vi "resha arc - v1.vi"() -> ()   [LabVIEW 2015]
doc: "This is the interface, the one VI which loads all the others. Run this one first.\n\n(the line below ensures settings are saved)\n[Red Tweezers Save Settings]"
uses:
  Matt Fall 2018 files/Matt working/Red Tweezers Image Processing Final 1-19/subvis/line_trapping.ctl
  Matt Fall 2018 files/Matt working/Red Tweezers Image Processing Final 1-19/subvis/spot.ctl
  <vilib>/userdefined/High Color/IMAQdx.ctl
  Matt Fall 2018 files/Matt working/Red Tweezers Image Processing Final 1-19/subvis/selection_element.ctl
  <vilib>/Analysis/Matrix/Datatypes/RealMatrix.ctl
  Matt Fall 2018 files/Matt working/Red Tweezers Image Processing Final 1-19/subvis/mouse_info.ctl
  <vilib>/Analysis/baseanly.llb/Real A x B.vi
  Matt Fall 2018 files/Matt working/Red Tweezers Image Processing Final 1-19/subvis/red_tweezers_globals_INTERNAL_VOLATILE.vi
  Matt Fall 2018 files/Matt working/Red Tweezers Image Processing Final 1-19/subvis/red_tweezers_globals.vi
  <vilib>/Analysis/Matrix/Numeric/Multiply/Multiply - RM,R.vi
  <vilib>/Analysis/Matrix/Numeric/Multiply/Multiply - R,RM.vi
  <vilib>/Analysis/NI_AALBase.lvlib
  <vilib>/vision/driver/NI_Vision_Acquisition_Software.lvlib
  <vilib>/vision/NI_Vision_Development_Module.lvlib
  <vilib>/Analysis/Matrix/NI_Matrix.lvlib
panel:
  out "Specific Point":cluster{i32, i32}
  out "bottomrx 3":dbl
  out "toply 3":dbl
  out "bottomry 3":dbl
  out "toplx 3":dbl
  out "Circles 2":T1(array[cluster]) {"Position"."Y" format="%.2f"; "Position"."X" format="%.2f"}
  out "Spot Storage":T2[](array[typedef]) {"Amplitude Correction" step=0.1; "Line Trapping"."Phase Gradient" step=0.05; "Line Trapping"."Vector"."x" step=1e-06 format="%#_6p"; "Line Trapping"."Vector"."y" step=1e-06 format="%#_6p"; "Line Trapping"."Vector"."z" step=1e-06 format="%#_6p"; "NA Position"."r" step=1e-06; "NA Position"."y" step=1e-06; "NA Position"."x" step=1e-06; "Position"."z" step=1e-06; "Position"."y" step=1e-06; "Position"."x" step=1e-06; "Phase" step=0.7753; "Intensity" step=0.1}
  out "# selected":i16
  out "Last Pattern":T2[](array[typedef]) {"Amplitude Correction" step=0.1; "Line Trapping"."Phase Gradient" step=0.05; "Line Trapping"."Vector"."x" step=1e-06 format="%#_6p"; "Line Trapping"."Vector"."y" step=1e-06 format="%#_6p"; "Line Trapping"."Vector"."z" step=1e-06 format="%#_6p"; "NA Position"."r" step=1e-06; "NA Position"."y" step=1e-06; "NA Position"."x" step=1e-06; "Position"."z" step=1e-06; "Position"."y" step=1e-06; "Position"."x" step=1e-06; "Phase" step=0.7753; "Intensity" step=0.1}
  out "Plugins":T4(array[cluster])=[{"Name"="ASI Stage", "Folder"=path "C:/Users/Richard Bowman/Dropbox/red_tweezers_1_4_rc4/plugins/ASI Stage.llb", "vi reference"=refnum, "Needs to be run"=TRUE, "Error"={"status"=FALSE, "code"=0, "source"=""}}, {"Name"="iTweezers", "Folder"=path "C:/Users/Richard Bowman/Dropbox/red_tweezers_1_4_rc4/plugins/iTweezers.llb", "vi reference"=refnum, "Needs to be run"=TRUE, "Error"={"status"=FALSE, "code"=0, "source"=""}}, {"Name"="MightexLED", "Folder"=path "C:/Users/Richard Bowman/Dropbox/red_tweezers_1_4_rc4/plugins/MightexLED.llb", "vi reference"=refnum, "Needs to be run"=TRUE, "Error"={"status"=FALSE, "code"=0, "source"=""}}]
  in  "Tab":T5(tab)
  out "Play Pressed":bool
  out "Y":dbl
  out "X":dbl
  in  "O Button":bool
  in  "OK Button":bool
  in  "Bubble Size":dbl=50.0002
  out "Hit Indicator":bool
  in  "On":bool
  out "Induce check":bool
  out "Area+ Buffer":dbl
  in  "Area to check":dbl=0.00025
  out "Prev Current Spot":dbl
  out "spots selected 2":i32=4
  out "Spot # Check":dbl
  out "Orig Y SC":dbl
  out "Orig X SC":dbl
  out "ID num check":dbl
  out "Value Check":dbl
  out "ID":dbl[](array[numeric])
  out "Null array":dbl[](array[numeric])
  out "Potential Collisions":dbl
  out "What to Check":dbl[](array[numeric])
  out "Num":dbl
  out "Old Y":dbl
  out "Old X":dbl
  out "init":dbl
  out "Looper":bool
  in  "Output to SLM":bool
  out "Maximum":dbl
  out "Projected Distance":dbl
  out "Previous Distance":dbl
  out "Group ID #":dbl
  in  "Buffer Zone":dbl=7e-05
  out "# of Spots":dbl
  out "Distance":dbl
  out "Hit":bool
  out "Y Displacement":dbl
  out "X Displacement":dbl
  out "Current Spot #":dbl
  out "spots selected":i32=4
  in  "lock aspect ratio":bool=TRUE
  in  "Size":cluster{"x":dbl, "y":dbl, "z":dbl} {"z" step=1e-06 format="%#_4p"; "y" step=1e-06 format="%#_4p"; "x" step=1e-06 format="%#_4p"}
  in  "phase":dbl step=0.7753
  in  "Vortex Charge":i8
  in  "Intensity":dbl=1.0 step=0.1
  in  "add to selection":bool
  in  "random position":bool
  in  "new spot":bool
  in  "delete":bool
  in  "rotate":bool
  in  "Rotation Axis":u16(ring)=2 items=["Z", "X", "Y", "Custom"]
  in  "Angle (degrees)":dbl=2.0
  in  "Custom Axis":cluster{dbl, dbl, dbl}
  in  "Spot Shape":enum32{"Normal", "Line", "NA", "Mixed"}(tab)=enum."Mixed"
  in  "Line Trapping":T3 {"Phase Gradient" step=0.05; "Vector"."x" step=1e-06 format="%#_4p"; "Vector"."y" step=1e-06 format="%#_4p"; "Vector"."z" step=1e-06 format="%#_4p"}
  in  "Scale back aperture":dbl=1.1 step=0.1
  in  "Scale BA":bool
  in  "Position on back aperture":cluster{"x":dbl, "y":dbl}={"x"=-5.84327907697451e-18, "y"=0.0} {"y" step=0.1 format="%#_4p"; "x" step=0.1 format="%#_4p"}
  in  "Radius on back aperture":dbl=1.1 step=0.1
  in  "Generate":bool
  in  "Pattern":T6(tab)
  in  "Spots across centre":i32=5
  in  "Reference Array?":bool
  in  "Fraction of SLM":dbl=1.0
  in  "Spots across centre":i32=5
  in  "N":cluster{i32, i32}
  in  "spacing/m":dbl=2.0
  in  "Iterations":i32=10
  out "non-uniformity":dbl(slide)=0.031119223416512406 scale=0.0..0.2
  out "efficiency":dbl(slide)=0.8985936267644501 scale=0.0..1.0
  in  "Optimise":bool
  in  "Reset Phase/Amplitude":bool
  in  "Fall-off/m":dbl=0.00025 min=0.0 step=1e-06 format="%#_4p"
  in  "Abort Plugin":bool
  in  "Plugin:":u16(ring)=1 items=["ASI Stage", "iTweezers", "MightexLED"]
  in  "Save Video":bool
  in  "Global ROI (requires restart)":i32[](array[numeric])=[0, 0, 1280, 512]
  in  "Zoom":bool
  in  "Draw ROI":bool
  in  "Zoom to Fit":bool
  out "Image Information":string="640x480 1.93X 8-bit image 255    (0,0)"
  in  "Camera":T7
  in  "Time per Frame (ms)":dbl
  in  "Edit Sequence Mode":bool
  in  "Manual Edit":bool
  in  "Bubble ID to Empty":dbl
  in  "Clearance Button":bool
  in  "Manual Sequence":bool
  in  "Play Sequence":bool
  in  "Reset":bool
  out "Sequence Instances":dbl
  out "Counter":dbl
  in  "Save State":bool
  out "Sequence On?":bool
  in  "Sequence Order":dbl
  out "Selection/Group":T8[](array[typedef])
  in  "Sequence Storer":T2[][](array[typedef]) {"Amplitude Correction" step=0.1; "Line Trapping"."Phase Gradient" step=0.05; "Line Trapping"."Vector"."x" step=1e-06 format="%#_6p"; "Line Trapping"."Vector"."y" step=1e-06 format="%#_6p"; "Line Trapping"."Vector"."z" step=1e-06 format="%#_6p"; "NA Position"."r" step=1e-06; "NA Position"."y" step=1e-06; "NA Position"."x" step=1e-06; "Position"."z" step=1e-06; "Position"."y" step=1e-06; "Position"."x" step=1e-06; "Phase" step=0.7753; "Intensity" step=0.1}
  in  "Object New Y":dbl
  in  "Object New X":dbl
  in  "Input Object Location":bool
  out "Time Elapsed(ms)":i32
  out "Start":i32
  out "Stop":i32
  out "Insert End":bool
  out "NewXYRates":dbl[][](array[numeric])
  out "NewXYArraySize":dbl
  out "NewXYArray":dbl[][](array[numeric])
  in  "Rates":dbl
  out "LCS Y":dbl
  out "LCS X":dbl
  in  "LCS":dbl
  in  "Play":bool
  out "Initiate Creation 2":dbl
  in  "Max Number of Bubbles 2":dbl
  in  "Number of Planned Sequence Frames 2":dbl
  in  "Add Additional Frames":bool
  in  "Frame Location":dbl
  in  "Additional Frames Wanted":dbl
  in  "Tab Control":enum32{"Line", "Arc"}(tab)
  out "X Rate":dbl
  out "Y Rate":dbl
  out "Original\nRadius":dbl
  out "Original\nD-Y":dbl
  out "Original\nD-X":dbl
  out "Original \nTheta":dbl
  out "Center Y":dbl
  out "Center X":dbl
  out "Center location":dbl[][](array[numeric])
  out "Degree Rate":dbl
  out "ROI-X":dbl
  out "ROI-Y":dbl
  in  "Lock Current Spot":bool
  out "Locked Current Spot":dbl
  out "Numeric":dbl
  out "probe":dbl
  in  "Insert":bool
  in  "Start at Which Frame?":dbl
  out "Original Y":dbl
  out "Original X":dbl
  in  "Mark Original Position":bool
  in  "How Many Frames?":dbl
  out "New Y":dbl
  out "New X":dbl
  out "Spot Storage 2":T2[](array[typedef]) {"Amplitude Correction" step=0.1; "Line Trapping"."Phase Gradient" step=0.05; "Line Trapping"."Vector"."x" step=1e-06 format="%#_6p"; "Line Trapping"."Vector"."y" step=1e-06 format="%#_6p"; "Line Trapping"."Vector"."z" step=1e-06 format="%#_6p"; "NA Position"."r" step=1e-06; "NA Position"."y" step=1e-06; "NA Position"."x" step=1e-06; "Position"."z" step=1e-06; "Position"."y" step=1e-06; "Position"."x" step=1e-06; "Phase" step=0.7753; "Intensity" step=0.1}
  in  "Numeric 2":dbl
  in  "Save":bool
  in  "Load":bool
  out "Current Y":dbl
  out "Current X":dbl
  out "Calc New  Y":dbl
  out "Calc New X":dbl
  out "distance bw y and rad":dbl
  out "distance  bw x and rad":dbl
  out "Object Y":dbl
  out "Object X":dbl
  in  "Camera Capture 2":bool
  out "Object y":dbl
  out "Object x":dbl
  out "Number of Matches Returned 2":dbl
  out "bottomry 2":dbl
  out "toply 2":dbl
  out "bottomrx 2":dbl
  out "toplx 2":dbl
  in  "Send Data":bool
  out "Camera 3":T9(plugin-control)
  in  "Circle Descriptor 2":cluster{"Min Radius":dbl, "Max Radius":dbl}={"Min Radius"=3.0, "Max Radius"=500.0}
  out "Video Frame Rate":dbl(knob)=50.00000000000003 scale=0.0..100.0 scale format="%.1f"
  out "Interface Frame Rate":dbl(knob)=97.23240312927678 scale=0.0..100.0 scale format="%.1f"
  in  "stop":bool=TRUE
  out "Numeric 4":dbl
  in  "Position":cluster{"x":dbl, "y":dbl, "z":dbl}={"x"=1e-06, "y"=-6.3e-06, "z"=0.0} {"z" step=1e-06 format="%#_4p"; "y" step=1e-06 format="%#_4p"; "x" step=1e-06 format="%#_4p"}
  out "Numeric 3":dbl
  out "ROI 1":T10
  out "ROI 0":T10
  out "MOP pressed":bool
  out "MOP pressed After":bool
  out "X Pos every 10 sec":dbl
  out "Elapsed Time":dbl
  out "Position Indicator":string
  out "Spot Checker":T2[](array[typedef]) {"Amplitude Correction" step=0.1; "Line Trapping"."Phase Gradient" step=0.05; "Line Trapping"."Vector"."x" step=1e-06 format="%#_6p"; "Line Trapping"."Vector"."y" step=1e-06 format="%#_6p"; "Line Trapping"."Vector"."z" step=1e-06 format="%#_6p"; "NA Position"."r" step=1e-06; "NA Position"."y" step=1e-06; "NA Position"."x" step=1e-06; "Position"."z" step=1e-06; "Position"."y" step=1e-06; "Position"."x" step=1e-06; "Phase" step=0.7753; "Intensity" step=0.1}
  out "Image":T9(plugin-control)
  # "Notes:\n\nIf you are doing non-sequence controls,\nthe delete function can be used as intended.\nHowever, do not use the delete function after\nrunning a sequence! Using it will prevent\nthe bubbles from appearing as the\nnumber of spots will change, which is\nessential for the sequence to work (it would\nbe displaying the maximum number of\nbubbles). \n\nIf you happen to delete a bubble, it can be \nrestored by inserting a new spot. Once enough\nspots have been restored, click on manual edit\nto correct the # of spots tracker. It should \nbe restored to where it originally was."
  # "The SLM can be used to shape spots; here you can restrict the NA of a spot (so it comes only from part of the back aperture), or create a line-trap"
  # "The traps do not have any spot-shaping applied (so they should just be diffraction-limited focal spots)."
  # "This shapes the amplitude (and phase) of the beam to create extended line traps.  The \"Phase Gradient\" control allows the Poynting vector to push things along the line.  Unfortunately, some work is needed on the scaling factors so the phase gradient control will need tweaking if the line trap has a nonzero z component."
  # "By default,each spot comes from the whole back aperture.  Here, you can limit a spot to come from a specific part of the back aperture."
  # "The control below allows you to scale the whole back aperture (i.e. the position and size of all the apertures).  It's a one-time operation, i.e. only changes things when you push \"ok\"."
  # "A Combination of line-trapping and NA restriction has been applied to these traps.  You can get at the line trap or NA parameters on the other tabs, switching to the NA tab does not delete the line-trap settings."
  # "This tab generates Shack-Hartmann type holograms, which are often useful when aligning the system, and arrays of spots."
  # "The controls above only work when using the \"IMAQdx with ROI Buttons\" case in the bottom loop.  You can save video regardless of camera code though."
  # "Manual Edit allows a user to\ngo to a specific sequence frame."
  # "To clear the sequence, you must\nclear the array. Right click on sequence\nstorer to do this."
  # "Use this to \"clear\" a \nspecific bubble. If\nworking on a sequence,\nuse this as your delete\nbutton! You can update\nthe view by using manual edit."
  # "Use the reset button\nto clear counter.\nIt becomes necessary\nwhen you clear the array,\nespecially in manual mode."
  # "Use the sequence creator tab to specify the\nnumber of bubbles you want along with\nthe number of frames.\n\nTo save at a specific interval, the sequence\norder can be used to place the state. If used\nto correct something, it will replace the\nentire sequence frame.\n\n\"Sequence On?\" is only used in auto mode."
  # "Multiple bubbles can  be done with the\nline function. One bubble at a time for the arc\nfunction."
  # "Using the Load/Save function:\n\nRed Tweezers itself is unable to save long \nsequences, but a separate program is able to\naccomplish this. To do this, follow these\nsteps:\n\n1. After creating your sequence, press the save\nbutton below.\n\n2. Then, go to the subvi folder and find\nSequenceSaver.vi.\n\n3. At the control \"Sequence Storer,\" right-click\nthe dimensions part of the array and go to\ndata operations.\n\n4. Press \"Make Current Values Default\" and save\nthe sequence.\n\n5. The next time you load the program, simply\npress load to re-acquire the sequence. You\nwill need to insert the bubbles again, but after\nthe first frame can be recovered by using\nSequenceControl.vi."
types:
  T1 = cluster{"Position":cluster{"X":sgl, "Y":sgl}, "Radius":dbl, "Score":dbl}[]
  T2 = typedef "spot.ctl" = cluster{"Position":cluster{"x":dbl, "y":dbl, "z":dbl}, "Intensity":dbl, "Vortex Charge":i8, "Phase":dbl, "NA Position":cluster{"x":dbl, "y":dbl, "r":dbl}, "Line Trapping":T3, "Amplitude Correction":dbl}
  T3 = typedef "line_trapping.ctl" = cluster{"Vector":cluster{"x":dbl, "y":dbl, "z":dbl}, "Phase Gradient":dbl}
  T4 = cluster{"Name":string, "Folder":path, "vi reference":refnum<vi>, "Needs to be run":bool, "Error":errorcluster}[]
  T5 = enum32{"Current Spot", "Rotate", "Spot Shape", "Patterns", "Plugins", "Video", "Sequence", "Sequence Creator", "Spot Control", "Load/Save", "Image Process"}
  T6 = enum32{"HCP Shack-Hartmann", "Square Shack-Hartmann", "Rectangular Grid"}
  T7 = typedef "IMAQdx.ctl" = refnum<k21>
  T8 = typedef "selection_element.ctl" = cluster{"Group ID":i32, "Selected":bool}
  T9 = typedef "IMAQ Image.ctl" = refnum<image>
  T10 = typedef "NI_Matrix.lvlib/RealMatrix.ctl" = dbl[][]
  T11 = typedef "mouse_info.ctl" = cluster{"Button Down":bool, "Dragging":bool, "Position (Image Pixels)":cluster{"X":dbl, "Y":dbl}, "Previous Position (Image Pixels)":cluster{"X":dbl, "Y":dbl}, "Button":u16, "Mods":cluster{"Double Click":bool, "Menu Key":bool}, "PlatMods":cluster{"Shift":bool, "Ctrl":bool, "Alt":bool, "Cmd":bool, "Opt":bool}}
  T12 = cluster{"Desired Font (Application)":enum16{"User-specified Font", "Application Font", "System Font", "Dialog Font"}, "[User-specified Font]":cluster{"Font Name":string, "Size":i16, "Strikeout?":bool, "Italic?":bool, "Underline?":bool, "Outline?":bool, "Shadow?":bool, "Bold?":bool, "Rotation Angle":dbl}, "Horizontal Alignment":i16, "Vertical Alignment":i16}
  T13 = cluster{"Position":cluster{"x":dbl, "y":dbl, "z":dbl}, "Intensity":dbl, "Vortex Charge":i8, "Phase":dbl, "NA Position":cluster{"x":dbl, "y":dbl, "r":dbl}, "Line Trapping":T3, "Amplitude Correction":dbl}
  T14 = enum16{"Set guide visibility", "Set grid visibility", "Show front panel", "Render on image"}
  T15 = enum32{"Current Spot", "Rotate", "Spot Shape", "Patterns", "Plugins", "Video"}
  T16 = enum16{"Left Button", "Center Button", "Right Button", "Window Close"}
  T17 = typedef "Image Type" = u32
  T18 = cluster{"number: 0 to 1":dbl, "number: 0 to 1":dbl}
  T19 = typedef "overlay_element.ctl" = cluster{"Tool":enum16{"Lines", "Oval", "Rectangle", "Text"}, "Points":cluster{"X":dbl, "Y":dbl}[], "Drawing Mode":u32, "Color":u32, "String":string}
  T20 = enum32{"Current Spot", "Rotate", "Spot Shape", "Patterns", "Plugins", "Video", "Particle Tracking", "Clamping", "Blank"}[]
  T21 = typedef "LVMenuShortCut.ctl" = cluster{"include Shift key?":bool, "include Ctrl key?":bool, "shortcut key":string}
  T22 = typedef "LVPoint32TypeDef.ctl" = cluster{"Horizontal":i32, "Vertical":i32}
  T23 = cluster{"Shift":bool, "Ctrl":bool, "Alt":bool, "Cmd":bool, "Opt":bool}
  T24 = cluster{"Button Down":bool, "Dragging":bool, "Mouse Coords (image pixels)":cluster{dbl, dbl}, "Mouse Coords (image pixels)":cluster{dbl, dbl}, "Button":u16, "Mods":cluster{"Double Click":bool, "Menu Key":bool}, "PlatMods":cluster{"Shift":bool, "Ctrl":bool, "Alt":bool, "Cmd":bool, "Opt":bool}}
  T25 = cluster{"Position":cluster{"X":sgl, "Y":sgl}, "Radius":dbl, "Score":dbl}
  T26 = cluster{"Global Rectangle":i32[], "Contours":cluster{"Contour Type":u32, "ROI Type":u32, "Points":i32[]}[]}
  T27 = cluster{"Contour Type":u32, "ROI Type":u32, "Points":i32[]}[]
  T28 = cluster{"Contour Type":u32, "ROI Type":u32, "Points":i32[]}
  T29 = cluster{"[0]":dbl, "[1]":dbl, "[2]":dbl, "[3]":dbl}
  T30 = cluster{"NewXYArray[0]":dbl, "NewXYArray[1]":dbl, "NewXYArray[2]":dbl, "NewXYArray[3]":dbl, "NewXYArray[4]":dbl, "NewXYArray[5]":dbl, "NewXYArray[6]":dbl, "NewXYArray[7]":dbl, "NewXYArray[8]":dbl}
  T31 = cluster{"Average Frame Time":dbl, "millisecond timer value":u32}
  T32 = cluster{"Position":cluster{"x":dbl, "y":dbl, "z":dbl}, "Intensity":dbl, "Vortex Charge":i8, "Phase":dbl, "NA Position":cluster{"x":dbl, "y":dbl, "r":dbl}, "Line Trapping":T3, "Amplitude Correction":dbl}[]
  T33 = enum32{"Bad", "Idle", "Run top level", "Running"}
  T34 = typedef "AviRefnum.ctl" = refnum<k1>
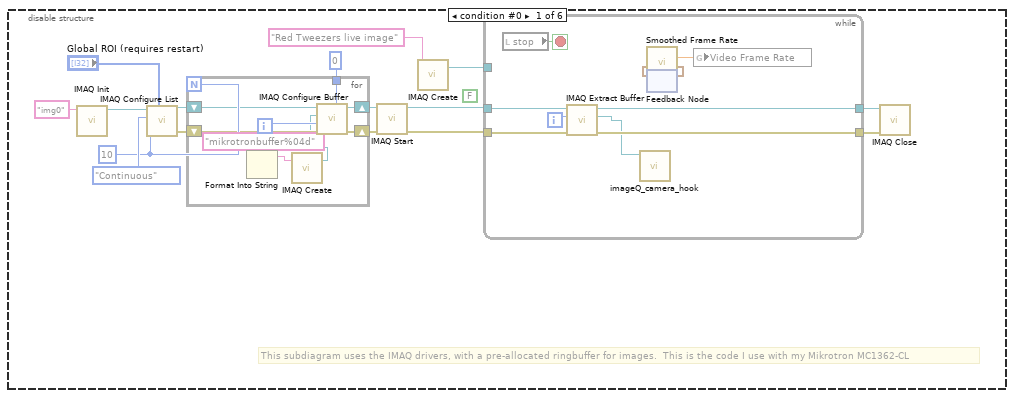
[diagram p3: hidden frame]
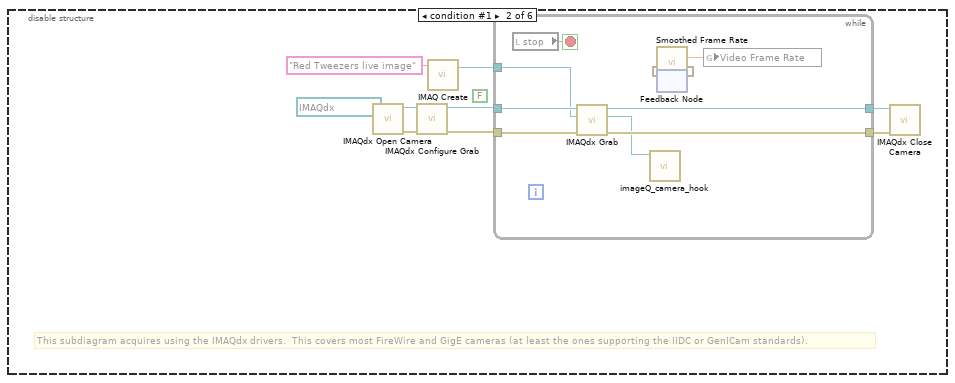
[diagram p4: hidden frame]
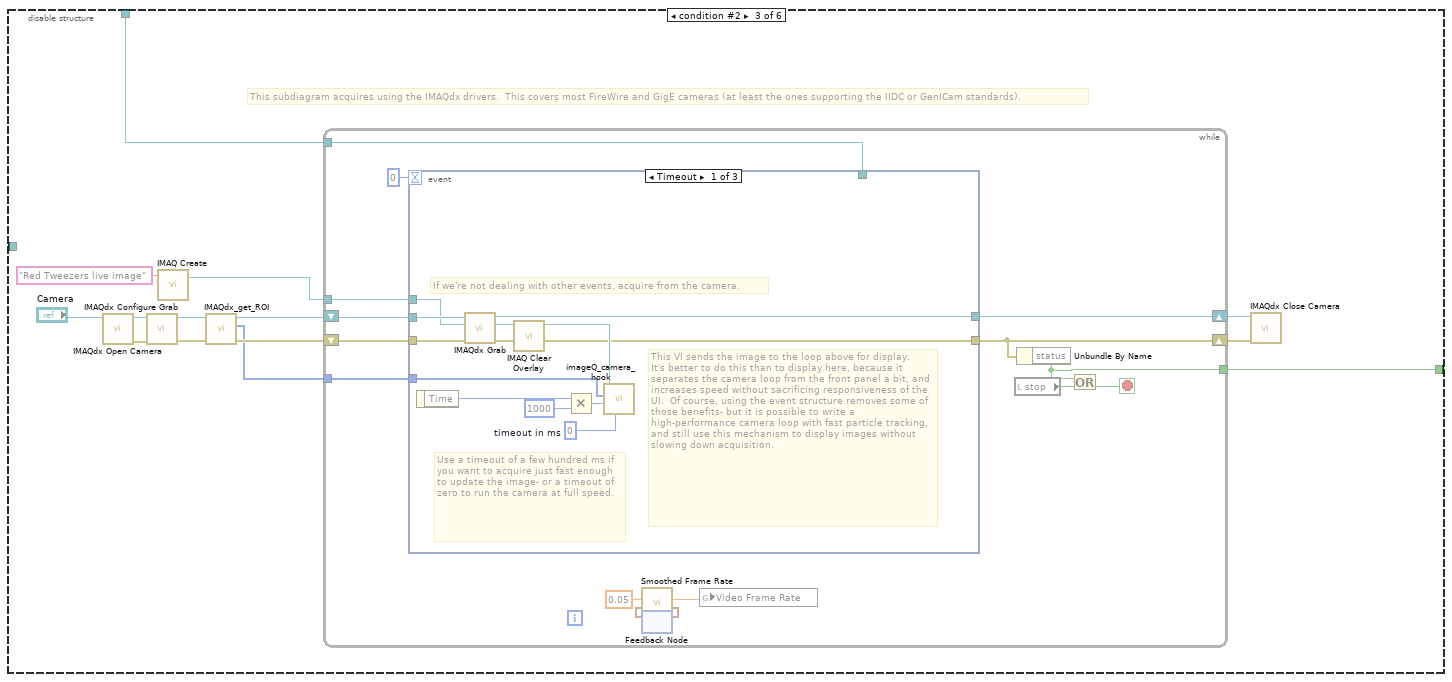
[diagram p5: hidden frame]
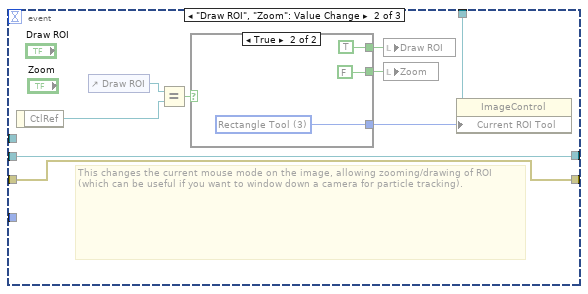
[diagram p6: hidden frame]
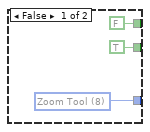
[diagram p7: hidden frame]
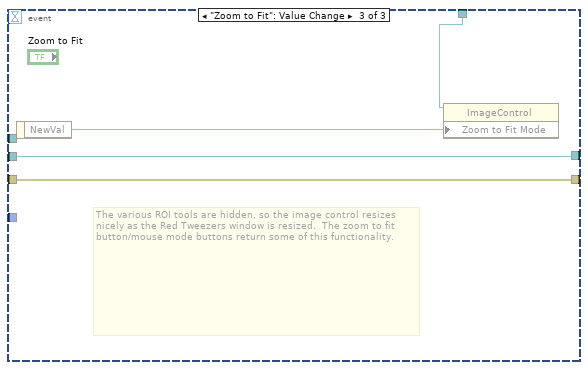
[diagram p8: hidden frame]
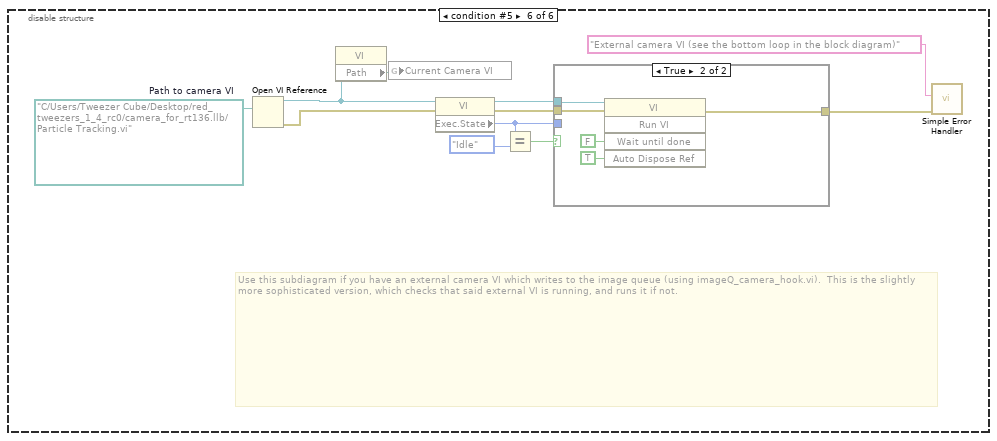
[diagram p10: hidden frame]
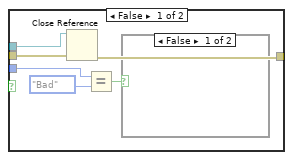
[diagram p11: hidden frame]
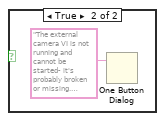
[diagram p12: hidden frame]
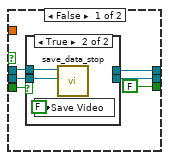
[diagram p13: hidden frame]
diagram:
  w11 = "red_tweezers_display_imageQ" ("Queue Name")
  w23 = T11 {"Button Down"=FALSE, "Dragging"=FALSE, "Position (Image Pixels)"={"X"=0.0, "Y"=0.0}, "Previous Position (Image Pixels)"={"X"=0.0, "Y"=0.0}, "Button"=0, "Mods"={"Double Click"=FALSE, "Menu Key"=FALSE}, "PlatMods"={"Shift"=FALSE, "Ctrl"=FALSE, "Alt"=FALSE, "Cmd"=FALSE, "Opt"=FALSE}}  # Mouse Information
  w24 = refnum<vi> refnum  # Image
  # "The funny looking feedback-node structure is deliberate (if odd).  We want to reload settings from the last used file (stored in the registry) only if this program has not been run since it was last loaded from file/recompiled.  That's why I use an uninitialised shift register: every time the program runs, it increments.  So, if it is zero, this is our first run (or we've been recently recompiled)."
  # "This loop handles the video that is displayed on-screen and saved to file."
  # "Initially, we only register to be told when the user clicks the image"
  # "This is the actual image control"
  # "This is a generic reference.\nIt is just a placeholder, so we can register for events later."
  # "This version of red tweezers uses two coordinate systems: \n1. Real Coordinates - corresponding to physical distances in 3D in microns\n2. Image Coordinates - position on the camera image, relative to the top left of the CURRENT ROI, measured in pixels. If the ROI changes, the relationship between \"real units\" and \"image pixels\" may change, so all values should be stored and presented to the user in REAL units unless there is a good reason to do otherwise."
  n1 = control-ref of="Plugin Pnl"() -> (w20:refnum<vi>)
  n2 = flat-sequence {
    tunnel: [w27] -> w6
    tunnel: w4 -> [_]
    frame #0 {
      n3 = vi-ref "red_tweezers_globals_INTERNAL.vi"() -> (w28:refnum<vi>)
      n4 = property class="VI"(reference=w28) -> ("Path"=w27:path)  [unwired: 1 in, 2 out]
      n5 = global write "red_tweezers_globals_INTERNAL_VOLATILE.vi" "Current Camera VI"(w27) -> ()
    }
  }
  n6 = control-ref of="Plugin:"() -> (w21:refnum<vi>)
  n7 = feedback #1() -> (w14:dbl)  [unwired: 1 in]
  n8 = Equal To 0?(x=w14) -> (x = 0?=w13:bool)
  n9 = Increment(x=w14) -> (x+1=w12:dbl)
  n10 = feedback-in #1(w12) -> ()
  n11 = call "plugins_load.vi"("Sub Panel"=w20, "Plugin Chooser"=w21) -> ("error out"=w15:errorcluster, "Plugins"=w17:T4)  [unwired: 2 in, 2 out]
  "Plugins" <- w17
  n12 = control-ref of="Image"() -> (w5:refnum<vi>)
  n13 = case shown="True" w13 {
    tunnel: w15 -> [_ w29]
    tunnel: [_ w29] -> w4
    frame False {
    }
    frame True {
      n14 = call "settings_load_default_file.vi"("error out"=w29) -> ()
    }
  }
  n15 = flat-sequence {
    tunnel: w4 -> [_]
    tunnel: w2 -> [w31]
    frame #0 {
      # "ensure we don't accidentally start saving video, and run UDP Sender to set up the hologram window."
      n16 = local write "Save Video"(FALSE ("background subtraction")) -> ()
      n17 = call "UDP Sender generic_2.vi"("Spots"=w31) -> ()  [unwired: 2 in, 1 out]
    }
  }
  n18 = global read "red_tweezers_globals.vi" "Selection/Group"() -> (w22:T8[])
  n19 = register-events(w5, w24, w24, w24) -> (reference out=w25:refnum<event-registration>)  [unwired: 2 in, 1 out]
  n20 = global read "red_tweezers_globals.vi" "Spots"() -> (w2:T2[])
  n21 = local write "stop"(FALSE ("STOP")) -> ()
  n22 = call "ensure_selection_matches_spots.vi"("Selection and Groups in"=w22, "Spots"=w2) -> ("Selection and Groups out"=w26:T8[], "Spots (duplicate)"=w1:T2[])  [unwired: 4 in]
  n23 = call "IMAQ Create"("Image Name"=w11) -> ("New Image"=w9:T9)  [unwired: 4 in, 1 out]
  n24 = call "imageQ_create_return_queue.vi"("Queue Name"=w11) -> ("queue out"=w10:refnum<queue>)
  n25 = while {
    shift-right: [w142] -> _
    shift-left: w1 -> [w162]
    shift-right: [w161] -> _
    shift-left: w26 -> [w160]
    shift-right: [w164] -> _
    shift-left: _ -> [w155]
    shift-right: [w163] -> _
    shift-left: _ -> [w154]
    tunnel: w5 -> [w159]
    shift-right: [w153] -> _
    shift-left: w23 -> [w152]
    shift-right: [w156] -> _
    shift-left: w25 -> [w157]
    border: errorcluster {"status"=FALSE, "code"=0, "source"=""} ("error out") -> [_]
    tunnel: [errorcluster {"status"=FALSE, "code"=0, "source"=""} ("error in (no error)")] -> w18
    border: w17 -> [_]
    tunnel: w1 -> [w143]
    stop <- w144 stop-if-true
    w59 = 7 items=["Red", "Green", "Blue", "Hue", "Saturation", "Luminance", "Value", "Intensity"] ("Color Plane")
    w62 = T17 0 items=["Grayscale (U8)", "Grayscale (I16)", "Grayscale (SGL)", "Complex (CSG)", "RGB (U32)", "HSL (U32)", "RGB (U64)", "Grayscale (U16)"] ("Image Type")
    # "ARRAY INICATORS ARE HIDDEN ON THE FRON PANNEL"
    # "CYCLE THROUGH THE NUMBERS ie. 0-6 \nFOR THE CASE OF 6 COORDINATES\nCURRENT CASE HAS 2 SETS OF COORDINATES"
    # "CASE STRUCTURE TO PLACE CODE INTO THE ARRAY"
    # "This is the calculation for the center of the detected circle, not sure where to put for now"
    # "This Play Function inserts bubbles from a given .mat file into the sequence storer"
    # "The function inserts the newly generated sequence for the automatic sequence generator. It also contains the code\nthe code necessary to check whether the bubbles will intersect with each other in the sequence."
    # "This calculates the size of the area including the buffer zone length.\nThe bubble diameter will also be included in the near future."
    # "The statement to the right controls the area that are being chcecked and checks\nwhich bubbles need to be checked.  There are two instances where this activates\nin this case:\n\nWhen a new bubble is selected\nWhen a bubble is deselected, reverting to the last current spot #\n\nThe other case, when the bubble moves out of the area specified, is located\ninside the while loop controlling the bubble movement with a mouse."
    # "Timer function example"
    # "These functions help with the calculations for the sequence generator."
    # "This loads the sequence from the \"saver\" VI. The save function below \"saves\" the sequence into the saver VI."
    # "The VI above is SequenceSaver.vi which contains the\ncode necessary to create a sequence."
    # "This case structure is the Save State structure. This stores\nthe current state of the bubbles (ie position)."
    # "Reset sets the counter back to zero. This is particularly useful \nwhen using the manual sequence."
    # "This case structure helps to continue the sequence.\nThis takes the true case of the Sequence On? function\nor the true case for the Manual Sequence function\nin order to go to the next sequence frame."
    # "This case structure allows for the playing of the sequence.\nThe amount of time it takes to go through the sequence\ncan be edited on the current spot menu."
    # "We only write to the image overlay when we are in one of the tabs, to prevent it disappearing when we are (for example) using the mouse."
    # "These wires control saving undo info. See the VI below's tip strips for details."
    # "Setting these wires to false means:\n(1) dragging moves the selection\n(2) clicking spots changes selection\nset them to true to stop the default mouse behaviour, don't wire them straight through!"
    n26 = event shown="[6] <Image>: Mouse Move" {
      selector: w157 -> [w618 w1289 w1294 w1516 w1544 w1561 w1658 _]
      dyn-events: [w618 w1288 w1294 w1514 w1541 w1562 w1658 _] -> w156
      timeout: 0 -> [_ _ _ _ _ _ _ _]
      tunnel: [w626 _ w1296 w1511 w1546 w1553 w1645 _] -> w164
      tunnel: [w625 _ w1295 w1510 w1545 w1552 w1649 _] -> w163
      tunnel: [w624 _ _ _ _ _ _ _] -> w115
      tunnel: w162 -> [w623 w1284 w1301 w1506 w1539 w1558 w1653 w1976]
      tunnel: [w622 w1284 w1299 w1506 w1539 w1549 w1651 w1976] -> w150
      tunnel: [w621 w1283 w1298 w1495 w1538 w1559 w1641 w1975] -> w149
      tunnel: w160 -> [w620 w1283 w1300 w1495 w1538 w1557 w1652 w1975]
      tunnel: w159 -> [w619 w1285 w1291 w1505 w1542 w1560 w1654 _]
      tunnel: [w617 _ w1293 w1515 T11 {"Button Down"=FALSE, "Dragging"=FALSE, "Position (Image Pixels)"={"X"=0.0, "Y"=0.0}, "Previous Position (Image Pixels)"={"X"=0.0, "Y"=0.0}, "Button"=0, "Mods"={"Double Click"=FALSE, "Menu Key"=FALSE}, "PlatMods"={"Shift"=FALSE, "Ctrl"=FALSE, "Alt"=FALSE, "Cmd"=FALSE, "Opt"=FALSE}} T11 {"Button Down"=FALSE, "Dragging"=FALSE, "Position (Image Pixels)"={"X"=0.0, "Y"=0.0}, "Previous Position (Image Pixels)"={"X"=0.0, "Y"=0.0}, "Button"=0, "Mods"={"Double Click"=FALSE, "Menu Key"=FALSE}, "PlatMods"={"Shift"=FALSE, "Ctrl"=FALSE, "Alt"=FALSE, "Cmd"=FALSE, "Opt"=FALSE}} w1657 _] -> w153
      tunnel: w152 -> [w617 _ w1293 _ _ w1556 w1648 _]
      tunnel: w155 -> [_ _ w1296 w1511 w1546 w1553 w1645 _]
      tunnel: w154 -> [_ _ w1295 w1510 w1545 w1552 w1649 _]
      tunnel: [w616 _ _ _ _ _ _ _] -> w151
      tunnel: [_ _ w1292 _ _ _ TRUE _] -> w148
      tunnel: [_ _ _ TRUE TRUE TRUE FALSE _] -> w147
      tunnel: [TRUE _ _ _ _ _ _ _] -> w145
      tunnel: [_ _ _ _ _ _ _ "stop"] -> w144
      tunnel: w143 -> [_ _ _ _ _ _ w1642 _]
      event Timeout {
        n27 = event-data() -> ()  [unwired: 1 in, 1 out]
        n28 = case shown="\"Current Spot\", Default" "Tab" {
          tunnel: [w641 w909 w1056 w1158 w1239 w1277] -> w622
          tunnel: w623 -> [w638 w911 w1057 w1160 w1239 w1277]
          tunnel: w620 -> [w627 w910 w1054 w1159 w1238 w1276]
          tunnel: [w640 w908 w1055 w1157 w1238 w1276] -> w621
          tunnel: [w628 _ TRUE _ _ _] -> w626
          tunnel: [w628 _ _ _ _ _] -> w625
          tunnel: [_ _ _ FALSE _ _] -> w624
          tunnel: w619 -> [_ _ _ _ _ w1273]
          tunnel: w617 -> [_ _ w1036 _ _ _]
          tunnel: [_ _ w1038 _ _ _] -> w616
          frame "Current Spot", Default {
            w628 = FALSE
            # "The function below contains the code necessary to use the automatic sequence generator to create specific movements. It also helps translate cases where the point is entered in not dragged.\nThis prevents bubbles from intersecting if the bubble is told not to intersect."
            # "If it's out of date, update front panel"
            n29 = call "find_centroid.vi"("Selection and Groups"=w627, "Spots"=w638) -> ("Mean Values"=w636:T2, "size"=w630:cluster{"x":dbl, "y":dbl, "z":dbl}, "centroid"=w631:cluster{"x":dbl, "y":dbl, "z":dbl}, "# selected"=w629:i16)  [unwired: 2 in, 1 out]
            n30 = stacked-sequence {
              tunnel: w629 -> [_ w643]
              frame #0 {
                n31 = local read "spots selected"() -> (→"spots selected 2":i32)
              }
              frame #1 {
                "spots selected" <- w643
              }
            }
            n32 = feedback-in #2(w636) -> ()
            n33 = feedback #2() -> (w637:T2)  [unwired: 1 in]
            n34 = feedback #3() -> (w635:cluster{"x":dbl, "y":dbl, "z":dbl})  [unwired: 1 in]
            n35 = feedback-in #3(w630) -> ()
            n36 = Not Equal?(x=w637, y=w636) -> (x != y?=w634:bool)
            n37 = Not Equal?(x=w635, y=w630) -> (x != y?=w633:bool)
            n38 = Or(x=w634, y=w633) -> (x .or. y?=w632:bool)
            n39 = case shown="True" w632 {
              tunnel: w636 -> [_ w649]
              tunnel: w630 -> [_ w645]
              frame False {
              }
              frame True {
                n40 = Unbundle By Name(w649) -> ("Position"=w644:cluster{"x":dbl, "y":dbl, "z":dbl}, "Intensity"=w647:dbl, "Vortex Charge"=w646:i8, "Phase"=w648:dbl)
                n41 = local write "Size"(w645) -> ()
                n42 = local write "Vortex Charge"(w646) -> ()
                n43 = local write "Intensity"(w647) -> ()
                n44 = local write "Position"(w644) -> ()
                n45 = local write "phase"(w648) -> ()
                n46 = Unbundle By Name(w644) -> ()  [unwired: 2 out]
              }
            }
            n47 = local write "Selection/Group"(w627) -> ()
            n48 = event shown="[0] Timeout" {
              selector: _ -> [_ _ _ _ _ _ _ _]
              dyn-events: _ -> [_ _ _ _ _ _ _ _]
              timeout: 10 -> [_ _ _ _ _ _ _ _]
              tunnel: w638 -> [w651 w655 w669 w692 w796 w841 w867 w890]
              tunnel: w627 -> [w650 w654 w672 w699 w783 w838 w864 w888]
              tunnel: [w651 w653 w670 w691 w784 w839 w865 w889] -> w641
              tunnel: [w650 w652 w671 w699 w783 w838 w864 w888] -> w640
              tunnel: w631 -> [_ _ _ _ w795 _ _ _]
              event Timeout {
                n49 = event-data() -> ()  [unwired: 3 out]
              }
              event "delete": Value Change {
                n50 = event-data() -> ()  [unwired: 7 out]
                n51 = call "delete_selected_spots.vi"("Selection/Group 3"=w654, "Spots 3"=w655) -> ("Selection/Group 2"=w652:T8[], "Spots 2"=w653:T2[])  [unwired: 4 in]
              }
              event "new spot": Value Change {
                # "If we're not adding it to the selection, de-select all the other spots"
                n52 = event-data() -> ()  [unwired: 7 out]
                n53 = call "coords_ROI_currentimage.vi"() -> ("Mono ROI"=w656:i32[])
                n54 = case shown="False" "add to selection" {
                  tunnel: w672 -> [w685 w690]
                  tunnel: [w684 w690] -> w667
                  frame False {
                    n55 = for {
                      tunnel: w685 -> [w688] mode=indexing
                      tunnel: [w689] -> w684 mode=indexing
                      n56 = Unbundle(w688) -> ("Group ID"=w687:i32)  [unwired: 1 out]
                      n57 = Bundle(cluster=w688, "Group ID"=w687, "Selected"=FALSE ("Label.Visible")) -> (w689:T8)
                    }
                  }
                  frame True {
                  }
                }
                n58 = Index Array(array=w656) -> (element #1=w662:i32, element #2=w663:i32, element #3=w661:i32, element #4=w660:i32)  [unwired: 4 in]
                n59 = Bundle("Numeric"=w662, "Numeric"=w663) -> (w657:cluster{"Numeric":i32, "Numeric":i32})  [unwired: 1 in]
                n60 = Bundle("Numeric"=w661, "Numeric"=w660) -> (w659:cluster{"Numeric":i32, "Numeric":i32})  [unwired: 1 in]
                n61 = Subtract(x=w659, y=w657) -> (x-y=w658:cluster{"Numeric":i32, "Numeric":i32})
                n62 = case shown="True" "random position" {
                  tunnel: [w674 w680] -> w665
                  tunnel: w658 -> [_ w676]
                  tunnel: w657 -> [_ w675]
                  frame False {
                    n63 = call "replace_position.vi"("Position"=cluster{"x":dbl, "y":dbl, "z":dbl} {"x"=0.0, "y"=0.0, "z"=0.0}) -> ("Spot"=w674:T2)  [unwired: 1 in, 2 out]
                  }
                  frame True {
                    n64 = Random Number (0-1)() -> (number: 0 to 1=w682:dbl)
                    n65 = Random Number (0-1)() -> (number: 0 to 1=w683:dbl)
                    n66 = Bundle("number: 0 to 1"=w683, "number: 0 to 1"=w682) -> (w681:T18)  [unwired: 1 out]
                    n67 = Multiply(x=w681, y=w676) -> (x*y=w678:cluster{dbl, dbl})
                    n68 = Add(x=w678, y=w675) -> (x+y=w677:cluster{dbl, dbl})
                    n69 = call "coords_image_to_real_currentimage.vi"("Position (pixels on image)"=w677) -> ("Position (real coords)"=w679:cluster{dbl, dbl, "Z":dbl})  [unwired: 9 in]
                    n70 = call "replace_position.vi"("Position"=w679) -> ("Spot"=w680:T2)  [unwired: 1 in, 2 out]
                  }
                }
                n71 = Build Array (concatenate)(w669, w665) -> (w670:T2[])
                n72 = Build Array (concatenate)(w667, cluster{i32, "Label.Visible":bool} {0, "Label.Visible"=TRUE}) -> (w671:T8[])
              }
              event "Position": Value Change {
                # "If the position has changed, translate the spots"
                n73 = event-data() -> ("OldVal"=w697:cluster{"x":dbl, "y":dbl, "z":dbl}, "NewVal"=w698:cluster{"x":dbl, "y":dbl, "z":dbl})  [unwired: 5 out]
                n74 = flat-sequence {
                  tunnel: w699 -> [w703]
                  tunnel: w696 -> [w702]
                  tunnel: w692 -> [w701]
                  tunnel: [w700] -> w693
                  frame #0 {
                    n75 = for {
                      tunnel: w701 -> [w708] mode=indexing
                      tunnel: w703 -> [w705] mode=indexing
                      tunnel: [w707] -> w700 mode=indexing
                      tunnel: w702 -> [w706]
                      n76 = Unbundle(w705) -> ("Selected"=w704:bool)  [unwired: 1 out]
                      n77 = case shown="True" w704 {
                        tunnel: w708 -> [w709 w714]
                        tunnel: [w709 w713] -> w707
                        tunnel: w706 -> [_ w710]
                        frame False {
                        }
                        frame True {
                          n78 = call "extract_position.vi"("Spot"=w714) -> ("Position"=w711:cluster{"x":dbl, "y":dbl, "z":dbl})
                          n79 = Add(x=w711, y=w710) -> (x+y=w712:cluster{"x":dbl, "y":dbl, "z":dbl})
                          n80 = call "replace_position.vi"("Position"=w712, "Spot in"=w714) -> ("Spot"=w713:T2)  [unwired: 2 out]
                        }
                      }
                    }
                  }
                }
                n81 = Subtract(x=w698, y=w697) -> (x-y=w696:cluster{"x":dbl, "y":dbl, "z":dbl})
                n82 = local read "# of Spots"() -> (w695:dbl)
                n83 = stacked-sequence {
                  tunnel: w692 -> [_ w719 _]
                  tunnel: w693 -> [_ w718 _]
                  tunnel: w695 -> [_ w717 _]
                  tunnel: [_ _ w766] -> w694
                  tunnel: w693 -> [_ _ w765]
                  tunnel: w692 -> [_ _ w764]
                  tunnel: [_ _ w763] -> w691
                  frame #0 {
                    n84 = local write "Looper"(FALSE) -> ()
                    "init" <- 0
                  }
                  frame #1 {
                    n85 = for {
                      N: w717 -> [_]
                      tunnel: w719 -> [w724]
                      tunnel: w718 -> [w729]
                      stop <- w730 stop-if-true
                      n86 = local read "init"() -> (w723:dbl)
                      n87 = Index Array(array=w729, index=w723) -> (element=w728:T2)
                      n88 = Index Array(array=w724, index=w723) -> (element=w722:T2)
                      n89 = Unbundle By Name(w728) -> ("Position.x"=w727:dbl, "Position.y"=w726:dbl)
                      n90 = local read "# of Spots"() -> (w725:dbl)
                      n91 = Unbundle By Name(w722) -> ("Position.x"=→"Old X":dbl, "Position.y"=→"Old Y":dbl)
                      n92 = local write "New X"(w727) -> ()
                      n93 = local write "New Y"(w726) -> ()
                      n94 = stacked-sequence {
                        tunnel: w724 -> [w735 _]
                        tunnel: w727 -> [w734 _]
                        tunnel: w726 -> [w733 _]
                        tunnel: w725 -> [w732 _]
                        tunnel: w723 -> [w731 _]
                        frame #0 {
                          n95 = for {
                            N: w732 -> [_]
                            tunnel: w735 -> [w757]
                            tunnel: w734 -> [w756]
                            tunnel: w733 -> [w754]
                            tunnel: w731 -> [w739]
                            i -> [w741]
                            stop <- w740 stop-if-true
                            n96 = Index Array(array=w757, index=w741) -> (element=w758:T2)
                            n97 = Unbundle By Name(w758) -> ("Position.x"=w755:dbl, "Position.y"=w753:dbl)
                            n98 = Subtract(x=w756, y=w755) -> (x-y=w752:dbl)
                            n99 = Subtract(x=w754, y=w753) -> (x-y=w751:dbl)
                            n100 = Square(x=w752) -> (x^2=w750:dbl)
                            n101 = Square(x=w751) -> (x^2=w749:dbl)
                            n102 = local read "# of Spots"() -> (w743:dbl)
                            n103 = Add(x=w750, y=w749) -> (x+y=w748:dbl)
                            n104 = local read "Buffer Zone"() -> (w738:dbl)
                            n105 = Square Root(x=w748) -> (sqrt(x)=w747:dbl)
                            n106 = Multiply(x=2, y=w738) -> (x*y=w736:dbl)
                            n107 = Less?(x=w747, y=w736) -> (x < y?=w745:bool)
                            n108 = Not Equal?(x=w739, y=w741) -> (x != y?=w744:bool)
                            n109 = Equal?(x=w743, y=w741) -> (x = y?=w746:bool)
                            n110 = And(x=w744, y=w745) -> (x .and. y?=w742:bool)
                            "Looper" <- w742
                            n111 = Or(x=w742, y=w746) -> (x .or. y?=w740:bool)
                          }
                        }
                        frame #1 {
                          n112 = local read "Looper"() -> (w759:bool)
                          n113 = case shown="False" w759 {
                            frame False {
                              n114 = local read "init"() -> (w760:dbl)
                              n115 = Add(x=w760, y=1) -> (x+y=w762:dbl)
                              n116 = local write "init"(w762) -> ()
                            }
                            frame True {
                            }
                          }
                        }
                      }
                      n117 = local read "Looper"() -> (w730:bool)
                    }
                  }
                  frame #2 {
                    n118 = local read "Looper"() -> (w767:bool)
                    n119 = case shown="True" w767 {
                      tunnel: w765 -> [w771 _]
                      tunnel: w764 -> [_ w779]
                      tunnel: ["This is an acceptable entry." "ERROR: A bubble will intersect the buffer zone."] -> w766
                      tunnel: [w771 w779] -> w763
                      frame False {
                        n120 = local write "Looper"(FALSE) -> ()
                        n121 = local read "Current Spot #"() -> (w772:dbl)
                        n122 = Index Array(array=w771, index=w772) -> (element=w770:T2)
                        n123 = Unbundle By Name(w770) -> ("Position.x"=w769:dbl, "Position.y"=w768:dbl)
                        n124 = local write "New Y"(w768) -> ()
                        n125 = local write "New X"(w769) -> ()
                      }
                      frame True {
                        # "Restore original position"
                        n126 = local write "Looper"(FALSE) -> ()
                        n127 = local read "Old Y"() -> (w776:dbl)
                        n128 = local read "Old X"() -> (w777:dbl)
                        n129 = local read "Position"() -> (w775:cluster{"x":dbl, "y":dbl, "z":dbl})
                        n130 = Bundle By Name(cluster=w775, "x"=w777, "y"=w776) -> (w778:cluster{"x":dbl, "y":dbl, "z":dbl})
                        n131 = local write "Position"(w778) -> ()
                      }
                    }
                  }
                }
                "Position Indicator" <- w694
              }
              event "Size": Value Change {
                # "If we were constraining the aspect ratio, or preventing a divide by zero, the size control on the FP may be incorrect.  We refresh it in here to stop it displaying a wrong value."
                # "If the size has changed, scale the spots"
                n132 = event-data() -> ("OldVal"=w788:cluster{"x":dbl, "y":dbl, "z":dbl}, "NewVal"=w794:cluster{"x":dbl, "y":dbl, "z":dbl})  [unwired: 5 out]
                n133 = Not Equal?(x=w788, y=w794) -> (x != y?=w787:cluster{"x":bool, "y":bool, "z":bool})
                n134 = Divide(x=w794, y=w788) -> (x/y=w793:cluster{"x":dbl, "y":dbl, "z":dbl})
                n135 = Not Equal To 0?(x=w788) -> (x != 0?=w786:cluster{"x":bool, "y":bool, "z":bool})
                n136 = And(x=w787, y=w786) -> (x .and. y?=w785:cluster{"x":bool, "y":bool, "z":bool})
                n137 = Cluster To Array(cluster=w785) -> (array=w792:bool[])
                n138 = Cluster To Array(cluster=w793) -> (array=w791:dbl[])
                n139 = case shown="True" "lock aspect ratio" {
                  tunnel: w792 -> [w800 w817]
                  tunnel: w791 -> [w799 w815]
                  tunnel: [w797 w807] -> w790
                  frame False {
                    # "We are not constraining the aspect ratio here, so just check we're not introducing NAs"
                    n140 = for {
                      tunnel: w800 -> [w806] mode=indexing
                      tunnel: w799 -> [w802] mode=indexing
                      tunnel: [w804] -> w798 mode=indexing
                      n141 = Not A Number/Path/Refnum?(number/path/refnum=w802) -> (NaN/Path/Refnum?=w803:bool)
                      n142 = Compound Arithmetic op=AND(w806, invert w803) -> (w805:bool)
                      n143 = Select(t=w802, s=w805, f=1.0) -> (s? t:f=w804:dbl)
                    }
                    n144 = Array To Cluster(array=w798) -> (cluster=w797:cluster{"[0]":dbl, "[1]":dbl, "[2]":dbl})
                  }
                  frame True {
                    # "Pick the first element that changed and use it.  Also need to make sure (1) an element did change and (2) everything's valid (no divide by zeros)"
                    n145 = Search 1D Array(1D array=w817, element=TRUE) -> (index of element=w814:i32)  [unwired: 1 in]
                    n146 = Index Array(array=w815, index=w814) -> (element=w810:dbl)
                    n147 = Not A Number/Path/Refnum?(number/path/refnum=w810) -> (NaN/Path/Refnum?=w813:bool)
                    n148 = Less Than 0?(x=w814) -> (x < 0?=w812:bool)
                    n149 = Or(x=w813, y=w812) -> (x .or. y?=w811:bool)
                    n150 = Select(t=1.0, s=w811, f=w810) -> (s? t:f=w808:dbl)
                    n151 = Bundle("x"=w808, "x"=w808, "x"=w808) -> (w807:cluster{"x":dbl, "x":dbl, "x":dbl})  [unwired: 1 in]
                  }
                }
                n152 = for {
                  tunnel: w796 -> [w823] mode=indexing
                  tunnel: w783 -> [w820] mode=indexing
                  tunnel: [w822] -> w784 mode=indexing
                  tunnel: w790 -> [w821]
                  tunnel: w795 -> [w818]
                  n153 = Unbundle(w820) -> ("Selected"=w819:bool)  [unwired: 1 out]
                  n154 = case shown="True" w819 {
                    tunnel: w823 -> [w824 w832]
                    tunnel: [w824 w831] -> w822
                    tunnel: w821 -> [_ w830]
                    tunnel: w818 -> [_ w826]
                    frame False {
                    }
                    frame True {
                      n155 = call "extract_position.vi"("Spot"=w832) -> ("Position"=w828:cluster{"x":dbl, "y":dbl, "z":dbl})
                      n156 = Subtract(x=w828, y=w826) -> (x-y=w829:cluster{"x":dbl, "y":dbl, "z":dbl})
                      n157 = Multiply(x=w829, y=w830) -> (x*y=w827:cluster{"x":dbl, dbl, dbl})
                      n158 = Add(x=w826, y=w827) -> (x+y=w825:cluster{"x":dbl, dbl, dbl})
                      n159 = call "replace_position.vi"("Position"=w825, "Spot in"=w832) -> ("Spot"=w831:T2)  [unwired: 2 out]
                    }
                  }
                }
                n160 = call "find_centroid.vi"("Selection and Groups"=w783, "Spots"=w784) -> ("size"=w782:cluster{"x":dbl, "y":dbl, "z":dbl})  [unwired: 2 in, 4 out]
                n161 = local write "Size"(w782) -> ()
              }
              event "Intensity": Value Change {
                # "When  the user changes intensity, scale all the spots selected so the new mean is correct but keep the ratio between the selected spots.\n\nThe exception to this is when the mean intensity is zero, in which case multiplying makes no sense- in that case we just replace with the new value."
                n162 = event-data() -> ("NewVal"=w833:dbl, "OldVal"=w840:dbl)  [unwired: 5 out]
                n163 = Equal To 0?(x=w840) -> (x = 0?=w836:bool)
                n164 = Not A Number/Path/Refnum?(number/path/refnum=w840) -> (NaN/Path/Refnum?=w835:bool)
                n165 = Or(x=w836, y=w835) -> (x .or. y?=w834:bool)
                n166 = Divide(x=w833, y=w840) -> (x/y=w837:dbl)
                n167 = for {
                  tunnel: w841 -> [w846] mode=indexing
                  tunnel: w838 -> [w848] mode=indexing
                  tunnel: [w845] -> w839 mode=indexing
                  tunnel: w837 -> [w844]
                  tunnel: w834 -> [w843]
                  tunnel: w833 -> [w842]
                  n168 = Unbundle(w848) -> ("Selected"=w847:bool)  [unwired: 1 out]
                  n169 = case shown="True" w847 {
                    tunnel: w846 -> [w849 w856]
                    tunnel: [w849 w853] -> w845
                    tunnel: w844 -> [_ w852]
                    tunnel: w843 -> [_ w851]
                    tunnel: w842 -> [_ w850]
                    frame False {
                    }
                    frame True {
                      n170 = Unbundle By Name(w856) -> ("Intensity"=w854:dbl)
                      n171 = case shown="True" w851 {
                        tunnel: [w859 w860] -> w855
                        tunnel: w854 -> [w858 _]
                        tunnel: w852 -> [w857 _]
                        tunnel: w850 -> [_ w860]
                        frame False {
                          n172 = Multiply(x=w858, y=w857) -> (x*y=w859:dbl)
                        }
                        frame True {
                        }
                      }
                      n173 = Bundle By Name(cluster=w856, "Intensity"=w855) -> (w853:T2)
                    }
                  }
                }
              }
              event "phase": Value Change {
                # "When  the user changes phase, translate the phase of all spots selectedd"
                n174 = event-data() -> ("NewVal"=w862:dbl, "OldVal"=w866:dbl)  [unwired: 5 out]
                n175 = Not A Number/Path/Refnum?(number/path/refnum=w866) -> (NaN/Path/Refnum?=w861:bool)
                n176 = Subtract(x=w862, y=w866) -> (x-y=w863:dbl)
                n177 = for {
                  tunnel: w867 -> [w872] mode=indexing
                  tunnel: w864 -> [w874] mode=indexing
                  tunnel: [w871] -> w865 mode=indexing
                  tunnel: w863 -> [w870]
                  tunnel: w861 -> [w869]
                  tunnel: w862 -> [w868]
                  n178 = Unbundle(w874) -> ("Selected"=w873:bool)  [unwired: 1 out]
                  n179 = case shown="False" w873 {
                    tunnel: w872 -> [w875 w882]
                    tunnel: [w875 w879] -> w871
                    tunnel: w870 -> [_ w878]
                    tunnel: w869 -> [_ w877]
                    tunnel: w868 -> [_ w876]
                    frame False {
                    }
                    frame True {
                      n180 = Unbundle By Name(w882) -> ("Phase"=w880:dbl)
                      n181 = case shown="False" w877 {
                        tunnel: [w885 w886] -> w881
                        tunnel: w880 -> [w884 _]
                        tunnel: w878 -> [w883 _]
                        tunnel: w876 -> [_ w886]
                        frame False {
                          n182 = Add(x=w884, y=w883) -> (x+y=w885:dbl)
                        }
                        frame True {
                        }
                      }
                      n183 = Bundle By Name(cluster=w882, "Phase"=w881) -> (w879:T2)
                    }
                  }
                }
              }
              event "Vortex Charge": Value Change {
                # "When  the user changes l, just set all selected spots to have that value of l."
                n184 = event-data() -> ("NewVal"=w887:i8)  [unwired: 6 out]
                n185 = for {
                  tunnel: w890 -> [w893] mode=indexing
                  tunnel: w888 -> [w895] mode=indexing
                  tunnel: [w892] -> w889 mode=indexing
                  tunnel: w887 -> [w891]
                  n186 = Unbundle(w895) -> ("Selected"=w894:bool)  [unwired: 1 out]
                  n187 = case shown="True" w894 {
                    tunnel: w893 -> [w896 w899]
                    tunnel: [w896 w898] -> w892
                    tunnel: w891 -> [_ w897]
                    frame False {
                    }
                    frame True {
                      n188 = Bundle By Name(cluster=w899, "Vortex Charge"=w897) -> (w898:T2)
                    }
                  }
                }
              }
            }
          }
          frame "Spot Shape" {
            # "We update the spot shape tab only when spots have changed OUTSIDE this tab.  This avoids unnecessary jumping about of the tab control."
            n189 = call "find_centroid.vi"("Selection and Groups"=w910, "Spots"=w911) -> ("Mean Values"=w906:T2)  [unwired: 2 in, 4 out]
            n190 = Wait (ms)(milliseconds to wait=u32 10) -> ()  [unwired: 1 out]
            n191 = call "spots_shape.vi"("Selection and Groups"=w910, "Spots"=w911) -> ("Spot Shape"=w913:enum32{"Normal", "Line", "NA", "Mixed"})  [unwired: 7 in]
            n192 = feedback-in #4(w906) -> ()
            n193 = feedback #4() -> (w907:T2)  [unwired: 1 in]
            n194 = Not Equal?(x=w907, y=w906) -> (x != y?=w912:bool)
            n195 = feedback #5() -> (w902:enum32{"Normal", "Line", "NA", "Mixed"})  [unwired: 1 in]
            n196 = feedback #6() -> (w904:T2)  [unwired: 1 in]
            n197 = Not Equal?(x=w904, y=w906) -> (x != y?=w903:bool)
            n198 = case shown="False" w903 {
              tunnel: w913 -> [_ w1032]
              tunnel: ["Spot Shape" w1032] -> w901
              frame False {
              }
              frame True {
                n199 = local write "Spot Shape"(w1032) -> ()
              }
            }
            n200 = feedback-in #5(w901) -> ()
            n201 = Not Equal?(x=w901, y=w902) -> (x != y?=w900:bool)
            n202 = case shown="\"Normal\", Default" w901 {
              tunnel: w911 -> [w917 w934 w960 w1030]
              tunnel: w910 -> [w916 w933 w959 w1029]
              tunnel: [w916 w932 w957 w1029] -> w908
              tunnel: [w915 w931 w958 w1030] -> w909
              tunnel: w906 -> [_ w930 w956 _]
              tunnel: w912 -> [_ w929 w955 _]
              tunnel: w900 -> [_ w927 w953 _]
              frame "Normal", Default {
                # "If \"normal\" is selected, don't allow any NA or line-trapping stuff"
                n203 = for {
                  tunnel: w917 -> [w920] mode=indexing
                  tunnel: w916 -> [w919] mode=indexing
                  tunnel: [w921] -> w915 mode=indexing
                  n204 = Unbundle(w919) -> ("Selected"=w918:bool)  [unwired: 1 out]
                  n205 = case shown="True" w918 {
                    tunnel: [w922 w926] -> w921
                    tunnel: w920 -> [w922 w925]
                    frame False {
                    }
                    frame True {
                      n206 = Bundle By Name(cluster=w925, "NA Position"=cluster{"x":dbl, "y":dbl, "r":dbl} {"x"=0.0, "y"=0.0, "r"=1.0} ("x"), "Line Trapping"=T3 {"Vector"={"x"=0.0, "y"=0.0, "z"=0.0}, "Phase Gradient"=0.0}) -> (w926:T2)
                    }
                  }
                }
              }
              frame "Line" {
                # "If it's out of date, update front panel"
                n207 = Or(x=w929, y=w927) -> (x .or. y?=w928:bool)
                n208 = case shown="True" w928 {
                  tunnel: w930 -> [_ w937]
                  frame False {
                  }
                  frame True {
                    n209 = Unbundle By Name(w937) -> ("Line Trapping"=w936:T3)
                    n210 = local write "Line Trapping"(w936) -> ()
                  }
                }
                n211 = event shown="[1] \"Line Trapping\": Value Change" {
                  selector: _ -> [_ _]
                  dyn-events: _ -> [_ _]
                  timeout: 10 -> [_ _]
                  tunnel: w934 -> [w939 w943]
                  tunnel: w933 -> [w938 w941]
                  tunnel: [w939 w942] -> w931
                  tunnel: [w938 w941] -> w932
                  event Timeout {
                    n212 = event-data() -> ()  [unwired: 3 out]
                  }
                  event Value Change {
                    # "If the line vector has changed, update it"
                    n213 = event-data() -> ("NewVal"=w940:T3)  [unwired: 6 out]
                    n214 = for {
                      tunnel: w943 -> [w948] mode=indexing
                      tunnel: w941 -> [w945] mode=indexing
                      tunnel: [w947] -> w942 mode=indexing
                      tunnel: w940 -> [w946]
                      n215 = Unbundle(w945) -> ("Selected"=w944:bool)  [unwired: 1 out]
                      n216 = case shown="True" w944 {
                        tunnel: w948 -> [w949 w951]
                        tunnel: [w949 w952] -> w947
                        tunnel: w946 -> [_ w950]
                        frame False {
                        }
                        frame True {
                          n217 = Bundle By Name(cluster=w951, "Line Trapping"=w950) -> (w952:T2)
                        }
                      }
                    }
                  }
                }
              }
              frame "NA" {
                n218 = Or(x=w953, y=w955) -> (x .or. y?=w954:bool)
                n219 = case shown="True" w954 {
                  tunnel: w956 -> [_ w965]
                  frame False {
                  }
                  frame True {
                    n220 = Unbundle By Name(w965) -> ("NA Position"=w964:cluster{"x":dbl, "y":dbl, "r":dbl})
                    n221 = call "xyz_to_xy.vi"("Position"=w964) -> ("Position (2D)"=w963:cluster{"x":dbl, "y":dbl}, "z"=w962:dbl)  [unwired: 6 out]
                    n222 = local write "Position on back aperture"(w963) -> ()
                    n223 = local write "Radius on back aperture"(w962) -> ()
                  }
                }
                n224 = event shown="[3] \"Scale BA\": Value Change" {
                  selector: _ -> [_ _ _ _]
                  dyn-events: _ -> [_ _ _ _]
                  timeout: 10 -> [_ _ _ _]
                  tunnel: w960 -> [w967 w973 w994 w1016]
                  tunnel: w959 -> [w966 w971 w991 w1017]
                  tunnel: [w967 w972 w992 w1014] -> w958
                  tunnel: [w966 w971 w991 w1017] -> w957
                  event Timeout {
                    n225 = event-data() -> ()  [unwired: 3 out]
                  }
                  event "Position on back aperture": Value Change {
                    # "If the position has changed, translate the spots"
                    n226 = event-data() -> ("OldVal"=w969:cluster{"x":dbl, "y":dbl}, "NewVal"=w970:cluster{"x":dbl, "y":dbl})  [unwired: 5 out]
                    n227 = Subtract(x=w970, y=w969) -> (x-y=w968:cluster{"x":dbl, "y":dbl})
                    n228 = for {
                      tunnel: w973 -> [w978] mode=indexing
                      tunnel: w971 -> [w975] mode=indexing
                      tunnel: [w977] -> w972 mode=indexing
                      tunnel: w968 -> [w976]
                      n229 = Unbundle(w975) -> ("Selected"=w974:bool)  [unwired: 1 out]
                      n230 = case shown="True" w974 {
                        tunnel: w978 -> [w979 w981]
                        tunnel: [w979 w982] -> w977
                        tunnel: w976 -> [_ w983]
                        frame False {
                        }
                        frame True {
                          n231 = Unbundle By Name(w981) -> ("NA Position"=w985:cluster{"x":dbl, "y":dbl, "r":dbl})
                          n232 = call "xy_to_xyz.vi"("Position (2D)"=w983) -> ("Position (3D)"=w984:cluster{dbl, dbl, dbl})  [unwired: 1 in, 2 out]
                          n233 = Add(x=w985, y=w984) -> (x+y=w980:cluster{dbl, dbl, dbl})
                          n234 = Bundle By Name(cluster=w981, "NA Position"=w980) -> (w982:T2)
                        }
                      }
                    }
                  }
                  event "Radius on back aperture": Value Change {
                    # "When  the user changes intensity, scale all the spots selected so the new mean is correct but keep the ratio between the selected spots.\n\nThe exception to this is when the mean intensity is zero, in which case multiplying makes no sense- in that case we just replace with the new value."
                    n235 = event-data() -> ("NewVal"=w986:dbl, "OldVal"=w993:dbl)  [unwired: 5 out]
                    n236 = Equal To 0?(x=w993) -> (x = 0?=w989:bool)
                    n237 = Not A Number/Path/Refnum?(number/path/refnum=w993) -> (NaN/Path/Refnum?=w988:bool)
                    n238 = Or(x=w989, y=w988) -> (x .or. y?=w987:bool)
                    n239 = Divide(x=w986, y=w993) -> (x/y=w990:dbl)
                    n240 = for {
                      tunnel: w994 -> [w999] mode=indexing
                      tunnel: w991 -> [w1001] mode=indexing
                      tunnel: [w998] -> w992 mode=indexing
                      tunnel: w990 -> [w997]
                      tunnel: w987 -> [w996]
                      tunnel: w986 -> [w995]
                      n241 = Unbundle(w1001) -> ("Selected"=w1000:bool)  [unwired: 1 out]
                      n242 = case shown="True" w1000 {
                        tunnel: w999 -> [w1002 w1009]
                        tunnel: [w1002 w1006] -> w998
                        tunnel: w997 -> [_ w1005]
                        tunnel: w996 -> [_ w1004]
                        tunnel: w995 -> [_ w1003]
                        frame False {
                        }
                        frame True {
                          n243 = Unbundle By Name(w1009) -> ("NA Position.r"=w1007:dbl)
                          n244 = case shown="False" w1004 {
                            tunnel: [w1012 w1013] -> w1008
                            tunnel: w1007 -> [w1011 _]
                            tunnel: w1005 -> [w1010 _]
                            tunnel: w1003 -> [_ w1013]
                            frame False {
                              n245 = Multiply(x=w1011, y=w1010) -> (x*y=w1012:dbl)
                            }
                            frame True {
                            }
                          }
                          n246 = Bundle By Name(cluster=w1009, "NA Position.r"=w1008) -> (w1006:T2)
                        }
                      }
                    }
                  }
                  event "Scale BA": Value Change {
                    n247 = event-data() -> ()  [unwired: 7 out]
                    n248 = for {
                      tunnel: w1017 -> [w1022] mode=indexing
                      tunnel: w1016 -> [w1020] mode=indexing
                      tunnel: "Scale back aperture" -> [w1019]
                      tunnel: [w1018] -> w1014 mode=indexing
                      n249 = Unbundle(w1022) -> ("Selected"=w1021:bool)  [unwired: 1 out]
                      n250 = case shown="True" w1021 {
                        tunnel: w1020 -> [w1023 w1024]
                        tunnel: w1019 -> [_ w1027]
                        tunnel: [w1023 w1025] -> w1018
                        frame False {
                        }
                        frame True {
                          n251 = Unbundle By Name(w1024) -> ("NA Position"=w1028:cluster{"x":dbl, "y":dbl, "r":dbl})
                          n252 = Multiply(x=w1027, y=w1028) -> (x*y=w1026:cluster{"x":dbl, "y":dbl, "r":dbl})
                          n253 = Bundle By Name(cluster=w1024, "NA Position"=w1026) -> (w1025:T2)
                        }
                      }
                    }
                  }
                }
              }
              frame "Mixed" {
              }
            }
            n254 = call "find_centroid.vi"("Selection and Groups"=w908, "Spots"=w909) -> ("Mean Values"=w905:T2)  [unwired: 2 in, 4 out]
            n255 = feedback-in #6(w905) -> ()
          }
          frame "Rotate" {
            w1043 = u32 0 items=["Frame", "Fill", "Highlight"] ("Drawing Mode")
            w1042 = u32 0 ("Color")
            w1039 = i16 100 ("radius")
            # "It's necessary to check this has changed to stop us unintentionally \"spinning\" the spots..."
            # "Draw the centroid as a spot, then a large circle+cross"
            # "It's important that this loop doesn't go too fast- it hogs the CPU.  However, each tab can have a different loop speed."
            n256 = Unbundle By Name(w1036) -> ("Position (Image Pixels)"=w1052:cluster{"X":dbl, "Y":dbl}, "Previous Position (Image Pixels)"=w1051:cluster{"X":dbl, "Y":dbl}, "Dragging"=w1053:bool)
            n257 = feedback-in #7(w1036) -> ()
            n258 = feedback #7() -> (w1037:T11)  [unwired: 1 in]
            n259 = call "find_centroid.vi"("Selection and Groups"=w1054, "Spots"=w1057) -> ("centroid"=w1050:cluster{"x":dbl, "y":dbl, "z":dbl})  [unwired: 2 in, 4 out]
            n260 = Not Equal?(x=w1036, y=w1037) -> (x != y?=w1034:bool)
            n261 = Wait (ms)(milliseconds to wait=u32 10) -> ()  [unwired: 1 out]
            n262 = And(x=w1034, y=w1053) -> (x .and. y?=w1035:bool)
            n263 = call "coords_real_to_image_currentview.vi"("Position (real coords)"=w1050) -> ("Position (pixels, relative to the top left of the image)"=w1033:cluster{dbl, dbl})  [unwired: 7 in, 1 out]
            n264 = case shown="True" w1035 {
              tunnel: w1057 -> [w1066 w1110]
              tunnel: [w1068 w1109] -> w1056
              tunnel: w1054 -> [w1067 w1111]
              tunnel: [w1067 w1111] -> w1055
              tunnel: w1050 -> [w1065 w1102]
              tunnel: w1052 -> [_ w1101]
              tunnel: w1051 -> [_ w1100]
              tunnel: w1033 -> [_ w1099]
              frame False {
                n265 = event shown="[1] Timeout" {
                  selector: _ -> [_ _]
                  dyn-events: _ -> [_ _]
                  timeout: 10 -> [_ _]
                  tunnel: [w1081 w1098] -> w1068
                  tunnel: w1067 -> [w1080 _]
                  tunnel: w1066 -> [w1079 w1098]
                  tunnel: w1065 -> [w1075 _]
                  event "rotate": Value Change {
                    n266 = event-data() -> ()  [unwired: 6 out]
                    n267 = case shown="3" "Rotation Axis" {
                      tunnel: [cluster{dbl, dbl, dbl} {0.0, 0.0, 1.0} ("Custom Axis") cluster{dbl, dbl, dbl} {1.0, 0.0, 0.0} ("Custom Axis") cluster{dbl, dbl, dbl} {0.0, 1.0, 0.0} ("Custom Axis") "Custom Axis"] -> w1076
                      frame 0, Default {
                        # "Z"
                      }
                      frame 1 {
                        # "X"
                      }
                      frame 2 {
                        # "Y"
                      }
                      frame 3 {
                      }
                    }
                    n268 = call "normalise_3d_vector.vi"("Vector"=w1076) -> ("Unit Vector"=w1078:cluster{dbl, dbl, dbl})  [unwired: 3 out]
                    n269 = Divide(x=6.283185307179586, y=360.0) -> (x/y=w1073:dbl)
                    n270 = Multiply(x="Angle (degrees)", y=w1073) -> (x*y=w1070:dbl)
                    n271 = call "arb_rotation_matrix.vi"("Unit Vector"=w1078, "theta"=w1070) -> ("Real Matrix"=w1082:T10)
                    n272 = for {
                      tunnel: w1080 -> [w1092] mode=indexing
                      tunnel: w1079 -> [w1087] mode=indexing
                      tunnel: [w1088] -> w1081 mode=indexing
                      tunnel: w1075 -> [w1090]
                      tunnel: w1082 -> [w1089]
                      n273 = Unbundle(w1092) -> ("Selected"=w1091:bool)  [unwired: 1 out]
                      n274 = case shown="True" w1091 {
                        tunnel: w1090 -> [_ w1097]
                        tunnel: [w1093 w1096] -> w1088
                        tunnel: w1087 -> [w1093 w1095]
                        tunnel: w1089 -> [_ w1094]
                        frame False {
                        }
                        frame True {
                          n275 = call "apply_matrix_transformation_to_spots.vi"("Transform centre (i.e. transform about this point)"=w1097, "Transformation Matrix (3x3)"=w1094, "Spot In"=w1095) -> ("Spot Out"=w1096:T2)  [unwired: 5 out]
                        }
                      }
                    }
                  }
                  event Timeout {
                    n276 = event-data() -> ()  [unwired: 4 out]
                  }
                }
              }
              frame True {
                # "if the mouse has not moved, stuff will be NaN, so let's make like a leopard and not change our spots"
                # "the magnitude of the change in our direction vector gives the rotation angle in radians"
                # "If it's within 100px of the centroid, pretend the mouse is on the surface of a sphere, and synthesize Z accordingly (z^2=100^2-x^2-y^2).  This allows rotation in 3d :)  The output should always be a unit vector."
                n277 = Build Array(w1101, w1100) -> (w1116:cluster{"X":dbl, "Y":dbl}[])
                n278 = for {
                  tunnel: w1099 -> [w1149]
                  tunnel: w1116 -> [w1145] mode=indexing
                  tunnel: [w1135] -> w1115 mode=indexing
                  n279 = Subtract(x=w1145, y=w1149) -> (x-y=w1140:cluster{dbl, dbl})
                  n280 = Divide(x=w1140, y=100.0 ("x")) -> (x/y=w1141:cluster{dbl, dbl})
                  n281 = Square(x=w1141) -> (x^2=w1148:cluster{dbl, dbl})
                  n282 = Unbundle(w1148) -> (w1146:dbl, w1147:dbl)
                  n283 = Add(x=w1146, y=w1147) -> (x+y=w1137:dbl)
                  n284 = Subtract(x=1.0, y=w1137) -> (x-y=w1143:dbl)
                  n285 = Square Root(x=w1137) -> (sqrt(x)=w1138:dbl)
                  n286 = Greater Than 0?(x=w1143) -> (x > 0?=w1144:bool)
                  n287 = case shown="False" w1144 {
                    tunnel: w1143 -> [_ w1156]
                    tunnel: [0.0 w1155] -> w1134
                    tunnel: w1141 -> [w1153 w1154]
                    tunnel: w1138 -> [w1152 _]
                    tunnel: [w1151 w1154] -> w1136
                    frame False {
                      n288 = Divide(x=w1153, y=w1152) -> (x/y=w1151:cluster{dbl, dbl})
                    }
                    frame True {
                      n289 = Square Root(x=w1156) -> (sqrt(x)=w1155:dbl)
                    }
                  }
                  n290 = call "xy_to_xyz.vi"("z"=w1134, "Position (2D)"=w1136) -> ("Position (3D)"=w1135:cluster{dbl, dbl, dbl})  [unwired: 2 out]
                }
                n291 = Index Array(array=w1115) -> (element #1=w1114:cluster{dbl, dbl, dbl}, element #2=w1105:cluster{dbl, dbl, dbl})  [unwired: 2 in]
                n292 = Add(x=w1114, y=w1105) -> (x+y=w1104:cluster{dbl, dbl, dbl})
                n293 = Subtract(x=w1114, y=w1105) -> (x-y=w1103:cluster{dbl, dbl, dbl})
                n294 = call "cross_product.vi"("b"=w1104, "a"=w1103) -> ("a cross b"=w1113:cluster{dbl, dbl, dbl})
                n295 = call "normalise_3d_vector.vi"("Vector"=w1113) -> ("Unit Vector"=w1112:cluster{dbl, dbl, dbl})  [unwired: 3 out]
                n296 = call "normalise_3d_vector.vi"("Vector"=w1103) -> ("magnitude"=w1107:dbl)  [unwired: 3 out]
                n297 = Not Equal To 0?(x=w1107) -> (x != 0?=w1106:bool)
                n298 = call "arb_rotation_matrix.vi"("Unit Vector"=w1112, "theta"=w1107) -> ("Real Matrix"=w1108:T10)
                n299 = case shown="True" w1106 {
                  tunnel: w1111 -> [_ w1122]
                  tunnel: w1110 -> [w1117 w1121]
                  tunnel: [w1117 w1120] -> w1109
                  tunnel: w1108 -> [_ w1119]
                  tunnel: w1102 -> [_ w1118]
                  frame False {
                  }
                  frame True {
                    n300 = for {
                      tunnel: w1122 -> [w1128] mode=indexing
                      tunnel: w1121 -> [w1125] mode=indexing
                      tunnel: [w1124] -> w1120 mode=indexing
                      tunnel: w1119 -> [w1126]
                      tunnel: w1118 -> [w1123]
                      n301 = Unbundle(w1128) -> ("Selected"=w1127:bool)  [unwired: 1 out]
                      n302 = case shown="True" w1127 {
                        tunnel: [w1129 w1132] -> w1124
                        tunnel: w1125 -> [w1129 w1133]
                        tunnel: w1126 -> [_ w1130]
                        tunnel: w1123 -> [_ w1131]
                        frame False {
                        }
                        frame True {
                          n303 = call "apply_matrix_transformation_to_spots.vi"("Transform centre (i.e. transform about this point)"=w1131, "Transformation Matrix (3x3)"=w1130, "Spot In"=w1133) -> ("Spot Out"=w1132:T2)  [unwired: 5 out]
                        }
                      }
                    }
                  }
                }
              }
            }
            n304 = call "coords_real_to_image_currentview.vi"("Position (real coords)"=w1050) -> ("Position (pixels, relative to the top left of the image)"=w1045:cluster{dbl, dbl}, "z (real coords)"=w1049:dbl)  [unwired: 7 in]
            n305 = expression code="z*1e7+20"(w1049) -> (w1061:dbl)
            n306 = In Range and Coerce(upper limit=100.0, x=w1061, lower limit=2.0) -> (coerced(x)=w1048:dbl)  [unwired: 1 out]
            n307 = Bundle("upper limit"=w1048, "upper limit"=w1048) -> (w1041:cluster{"upper limit":dbl, "upper limit":dbl})  [unwired: 1 in]
            n308 = call "myoverlay_oval.vi"("Color"=w1042, "Drawing Mode"=w1043, "Size"=w1041, "Centre Position (pixels on image)"=w1045) -> ("Overlay Elements Out"=w1047:T19[])  [unwired: 5 in]
            n309 = Bundle("radius"=w1039, "radius"=w1039) -> (w1040:cluster{"radius":i16, "radius":i16})  [unwired: 1 in]
            n310 = call "myoverlay_oval.vi"("Color"=w1042, "Drawing Mode"=w1043, "Size"=w1040, "Centre Position (pixels on image)"=w1045, "Overlay Elements In"=w1047) -> ("Overlay Elements Out"=w1046:T19[])  [unwired: 4 in]
            n311 = Multiply(x=w1039, y=cluster{dbl, dbl}[] [{0.0, 0.0}, {1.0, 0.0}, {0.0, 0.0}, {0.0, 1.0}, {0.0, 0.0}, {-1.0, 0.0}, {0.0, 0.0}, {0.0, -1.0}, {0.0, 0.0}]) -> (x*y=w1058:cluster{dbl, dbl}[])
            n312 = Add(x=w1045, y=w1058) -> (x+y=w1044:cluster{dbl, dbl}[])
            n313 = call "myoverlay_lines.vi"("Color"=w1042, "Drawing Mode"=w1043, "Line Endpoints"=w1044, "Overlay Elements In"=w1046) -> ("Overlay Elements Out"=w1038:T19[])  [unwired: 5 in]
          }
          frame "Patterns" {
            n314 = event shown="[3] \"Optimise\": Value Change" {
              selector: _ -> [_ _ _ _ _]
              dyn-events: _ -> [_ _ _ _ _]
              timeout: u32 10 ("milliseconds to wait") -> [_ _ _ _ _]
              tunnel: [w1175 w1205 w1209 w1212 w1223] -> w1158
              tunnel: [w1174 w1206 w1208 w1215 w1224] -> w1157
              tunnel: w1160 -> [w1173 w1205 w1209 w1213 w1222]
              tunnel: w1159 -> [w1172 w1206 w1208 w1215 w1224]
              event "Generate": Value Change {
                # "If there were previous spots, centre the pattern on the spots"
                n315 = event-data() -> ()  [unwired: 1 in, 1 out]
                n316 = call "find_centroid.vi"("Selection and Groups"=w1172, "Spots"=w1173) -> ("size"=w1168:cluster{"x":dbl, "y":dbl, "z":dbl}, "centroid"=w1164:cluster{"x":dbl, "y":dbl, "z":dbl}, "# selected"=w1170:i16)  [unwired: 2 in, 2 out]
                n317 = Greater?(x=w1170, y=i16 1) -> (0:w1165:bool)
                n318 = case shown="False" w1165 {
                  tunnel: w1168 -> [_ w1191]
                  tunnel: [cluster{"x":dbl, "y":dbl, "z":dbl} {"x"=2e-05, "y"=2e-05, "z"=2e-05} ("size") w1191] -> w1167
                  frame False {
                  }
                  frame True {
                  }
                }
                n319 = case shown="\"HCP Shack-Hartmann\"" "Pattern" {
                  tunnel: [w1193 w1196 w1202] -> w1166
                  tunnel: w1167 -> [_ w1195 _]
                  frame "Square Shack-Hartmann" {
                    n320 = call "patterns_square_shack_hartmann.vi"("N"="Spots across centre") -> ("Spots"=w1193:T2[])
                  }
                  frame "HCP Shack-Hartmann" {
                    n321 = Unbundle By Name(w1195) -> ("x"=w1194:dbl)
                    n322 = call "pattern_hcp_shack_hartmann.vi"("Width"=w1194, "Reference Array?"="Reference Array?", "Fraction of SLM"="Fraction of SLM", "N"="Spots across centre") -> ("Shack-Hartmann Spots"=w1196:T2[])  [unwired: 7 in]
                  }
                  frame "Rectangular Grid" {
                    n323 = call "patterns_rectangular_grid.vi"("spacing/m"="spacing/m", "N"="N") -> ("Spots"=w1202:T2[])
                  }
                }
                n324 = local write "Generate"(FALSE ("Generate")) -> ()
                n325 = case shown="True" w1165 {
                  tunnel: w1166 -> [w1178 w1182]
                  tunnel: w1164 -> [_ w1184]
                  tunnel: [w1178 w1180] -> w1176
                  frame False {
                  }
                  frame True {
                    n326 = call "find_centroid.vi"("Spots"=w1182) -> ("centroid"=w1183:cluster{"x":dbl, "y":dbl, "z":dbl}, "# selected"=→"# selected":i16)  [unwired: 3 in, 3 out]
                    n327 = Subtract(x=w1184, y=w1183) -> (x-y=w1181:cluster{"x":dbl, "y":dbl, "z":dbl})
                    n328 = for {
                      tunnel: w1182 -> [w1187] mode=indexing
                      tunnel: w1181 -> [w1186]
                      tunnel: [w1185] -> w1180 mode=indexing
                      n329 = call "extract_position.vi"("Spot"=w1187) -> ("Position"=w1188:cluster{"x":dbl, "y":dbl, "z":dbl})
                      n330 = Add(x=w1188, y=w1186) -> (x+y=w1189:cluster{"x":dbl, "y":dbl, "z":dbl})
                      n331 = call "replace_position.vi"("Position"=w1189, "Spot in"=w1187) -> ("Spot"=w1185:T2)  [unwired: 2 out]
                    }
                  }
                }
                "Last Pattern" <- w1176
                n332 = call "ensure_selection_matches_spots.vi"("Select All (default: no)"=TRUE ("Select All (default: true)"), "Spots"=w1176) -> ("Selection and Groups out"=w1174:T8[], "Spots (duplicate)"=w1175:T2[])  [unwired: 4 in]
              }
              event "Spots across centre", "Fraction of SLM", "Reference Array?", "N", "spacing/m", "Spots across centre": Value Change {
                n333 = event-data() -> ()  [unwired: 1 in, 1 out]
                n334 = local read "Last Pattern"() -> (w1204:T2[])
                n335 = Equal?(x=w1205, y=w1204) -> (x = y?=w1203:bool)
                n336 = case shown="True" w1203 {
                  selector: w1203 -> [_ w1207]
                  frame False {
                  }
                  frame True {
                    n337 = property on="Generate" class="Bool (strict)"("Val(Sgnl)"=w1207) -> ()  [unwired: 2 in, 2 out]
                  }
                }
              }
              event Timeout {
                n338 = event-data() -> ()  [unwired: 1 in, 1 out]
              }
              event "Optimise": Value Change {
                n339 = event-data() -> ()  [unwired: 1 in, 1 out]
                n340 = for {
                  N: "Iterations" -> [_]
                  tunnel: 203 ("Optimisation Resolution") -> [w1219]
                  shift-right: [w1220] -> w1212
                  shift-left: w1213 -> [w1221]
                  tunnel: "Fall-off/m" -> [w1216]
                  n341 = call "do_gsw_step.vi"("Optimisation Resolution"=w1219, "Sinc Zero"=w1216, "Spots In"=w1221) -> ("non-uniformity"=→"non-uniformity":dbl, "efficiency"=→"efficiency":dbl, "Spots Out"=w1220:T2[])  [unwired: 6 in]
                }
              }
              event "Reset Phase/Amplitude": Value Change {
                n342 = event-data() -> ()  [unwired: 1 in, 1 out]
                n343 = for {
                  tunnel: [w1227] -> w1223 mode=indexing
                  tunnel: w1222 -> [w1228] mode=indexing
                  n344 = Bundle By Name(cluster=w1228, "Phase"=0.0, "Amplitude Correction"=0.0) -> (w1227:T2)
                }
              }
            }
          }
          frame "Plugins" {
            # "The local variable ensures the references are  correct when they make it through to the \"close plugins\" block."
            # "This is the error from loading/unloading VIs on the front panel"
            n345 = control-ref of="Plugin Pnl"() -> (w1232:refnum<vi>)
            n346 = Wait (ms)(milliseconds to wait=u32 10) -> ()  [unwired: 1 out]
            n347 = feedback #8() -> (w1231:T4)
            n348 = feedback #9() -> (w1233:errorcluster)
            n349 = event shown="[1] \"Plugin:\": Value Change" {
              selector: _ -> [_ _ _]
              dyn-events: _ -> [_ _ _]
              timeout: 10 -> [_ _ _]
              tunnel: "Abort Plugin" -> [w1240 _ _]
              tunnel: "Plugin:" -> [w1245 _ w1261]
              tunnel: w1233 -> [w1244 w1259 w1263]
              tunnel: [w1243 w1254 w1262] -> w1234
              tunnel: [w1242 w1255 w1265] -> w1230
              tunnel: w1231 -> [w1246 w1256 w1264]
              tunnel: w1232 -> [_ w1257 _]
              event Timeout {
                n350 = event-data() -> ()  [unwired: 1 in, 2 out]
                n351 = Not(x=w1240) -> (.not. x?=w1241:bool)
                n352 = case shown="True" w1241 {
                  tunnel: w1246 -> [w1248 w1253]
                  tunnel: w1245 -> [_ w1252]
                  tunnel: w1244 -> [w1247 w1251]
                  tunnel: [w1247 w1250] -> w1243
                  tunnel: [w1248 w1249] -> w1242
                  frame False {
                  }
                  frame True {
                    n353 = call "plugins_run.vi"("Error In"=w1251, "Plugin Index"=w1252, "Plugins In"=w1253) -> ("Error Out"=w1250:errorcluster, "Plugins"=w1249:T4)  [unwired: 7 in]
                  }
                }
              }
              event "Plugin:": Value Change {
                n354 = event-data() -> ("NewVal"=w1258:u16)  [unwired: 1 in]
                n355 = call "plugins_switch.vi"("error in"=w1259, "Plugin Pnl"=w1257, "Plugin Index"=w1258, "Plugins In"=w1256) -> ("error out"=w1254:errorcluster, "Plugins Out"=w1255:T4)  [unwired: 4 in]
              }
              event "Abort Plugin": Value Change {
                n356 = event-data() -> ("NewVal"=w1260:bool)  [unwired: 1 in]
                n357 = case shown="True" w1260 {
                  tunnel: [w1267 w1272] -> w1265
                  tunnel: w1264 -> [w1267 w1271]
                  tunnel: w1263 -> [w1266 w1270]
                  tunnel: [w1266 w1269] -> w1262
                  tunnel: w1261 -> [_ w1268]
                  frame False {
                  }
                  frame True {
                    n358 = call "plugins_abort.vi"("Error In"=w1270, "Plugin Index"=w1268, "Plugins In"=w1271) -> ("Error Out"=w1269:errorcluster, "Plugins Out"=w1272:T4)  [unwired: 7 in]
                  }
                }
              }
            }
            n359 = feedback-in #8(w1230) -> ()
            n360 = feedback-in #9(w1234) -> ()
            n361 = local write "Plugins"(w1230) -> ()
          }
          frame "Video" {
            # "All the controls on this tab are in the bottom (camera) loop."
            n362 = Wait (ms)(milliseconds to wait=u32 10) -> ()  [unwired: 1 out]
            n363 = property on="Property Node" class="ImageControl"(reference=w1273) -> ("Image Information String"=→"Image Information":string)  [unwired: 1 in, 2 out]
          }
        }
      }
      event "Tab": Value Change {
        w1281 = T20 [enum."Video", enum."Particle Tracking"] items=["Current Spot", "Rotate", "Spot Shape", "Patterns", "Plugins", "Video", "Particle Tracking", "Clamping", "Blank"]
        w1286 = refnum<vi> refnum  # Image
        # "This allows us to disable custom mouse-handling for certain tabs.  It can also be done from within the \"mouse down\" event case."
        n364 = event-data() -> ("NewVal"=w1282:T5)  [unwired: 1 in, 3 out]
        n365 = Equal?(x=w1281, y=w1282) -> (x = y?=w1280:bool[])
        n366 = Or Array Elements(Boolean array=w1280) -> (logical OR=w1279:bool)
        n367 = Not(x=w1279) -> (.not. x?=w1278:bool)
        n368 = Select(t=w1285, s=w1278, f=w1286) -> (s? t:f=w1287:refnum<vi>)
        n369 = register-events(reference=w1289, w1287, w1286, w1286, w1286) -> (reference out=w1288:refnum<event-registration>)  [unwired: 1 in, 1 out]
      }
      event Menu Selection (User) {
        n370 = event-data() -> ("ItemTag"=w1297:string, "MenuRef"=w1290:refnum<k9>)  [unwired: 1 in]
        n371 = case shown="\"ToggleSavingData\"" w1297 {
          tunnel: w1301 -> [w1305 w1315 w1324 w1338 w1357 w1361 w1364 w1371 w1378 w1380 w1383 w1412 w1438 w1459 w1470 w1481 w1484 w1486 w1491 w1494]
          tunnel: w1300 -> [w1304 w1314 w1323 w1347 w1356 w1360 w1362 w1369 w1377 w1379 w1382 w1411 w1437 w1458 w1469 w1480 w1483 w1487 w1492 w1493]
          tunnel: [w1305 w1315 w1324 w1338 w1355 w1358 w1364 w1371 w1378 w1380 w1383 w1412 w1438 w1459 w1470 w1481 w1484 w1486 w1491 w1494] -> w1299
          tunnel: [w1304 w1314 w1323 w1347 w1354 w1359 w1363 w1370 w1376 w1381 w1384 w1411 w1437 w1458 w1469 w1480 w1483 w1487 w1492 w1493] -> w1298
          tunnel: [_ _ _ _ TRUE _ _ _ _ _ _ _ _ _ _ _ _ _ _ _] -> w1292
          tunnel: w1291 -> [_ _ _ _ _ _ _ _ _ _ _ w1410 w1436 w1450 _ _ _ _ _ _]
          tunnel: w1290 -> [_ _ _ _ _ _ _ _ _ _ _ w1401 w1430 w1453 w1464 w1475 _ _ _ _]
          frame "ToggleSavingData" {
            # "Data is saved from the middle loop: look there for an explanation."
            n372 = local read "Save Video"() -> (w1303:bool)
            n373 = Not(x=w1303) -> (.not. x?=w1302:bool)
            n374 = local write "Save Video"(w1302) -> ()
          }
          frame "SaveStateToFile" {
            # "Save the current settings (i.e. the values of all the controls in VIs that have [Red Tweezers Save Settings] in their documentation string) to a file."
            n375 = call "File Dialog"("prompt"="Please select a location to save the settings", "button label"="Save", "default name"="red_tweezers_settings.xml", "pattern (all files)"="*.xml" ("pattern label"), "pattern label"="XML Settings Files") -> ("selected path"=w1313:path, "cancelled"=w1306:bool)  [unwired: 7 in, 2 out]
            n376 = Not(x=w1306) -> (.not. x?=w1307:bool)
            n377 = case shown="True" w1307 {
              tunnel: w1313 -> [_ w1317]
              frame False {
              }
              frame True {
                n378 = Path To String(path=w1317) -> (string=w1316:string)
                n379 = call "settings_save_to_file.vi"("XML File Path"=w1317) -> ()  [unwired: 11 in]
                n380 = call "settings_filename_to_registry.vi"("Last Used Settings File"=w1316) -> ()  [unwired: 11 in]
              }
            }
          }
          frame "SaveStateToCurrentFile" {
            # "As SaveStateToFile, but using the current file (i.e. Save not Save As...)."
            n381 = global read "red_tweezers_globals_INTERNAL_VOLATILE.vi" "Current Settings File"() -> (w1322:path)
            n382 = call <vilib>:"Check if File or Folder Exists.vi"("path"=w1322) -> ("file or folder exists?"=w1321:bool, "dup path"=w1320:path)  [unwired: 8 in, 1 out]
            n383 = case shown="True" w1321 {
              selector: w1321 -> [_ w1335]
              tunnel: w1320 -> [_ w1336]
              tunnel: [w1327 w1336] -> w1319
              tunnel: [w1328 w1335] -> w1318
              frame False {
                n384 = call "File Dialog3"("prompt"="Please select a location to save the settings", "button label"="Save", "default name"="red_tweezers_settings.xml", "pattern (all files)"="*.xml" ("pattern label"), "pattern label"="XML Settings Files") -> ("selected path"=w1327:path, "cancelled"=w1334:bool)  [unwired: 7 in, 2 out]
                n385 = Not(x=w1334) -> (.not. x?=w1328:bool)
              }
              frame True {
              }
            }
            n386 = case shown="True" w1318 {
              tunnel: w1319 -> [_ w1326]
              frame False {
              }
              frame True {
                n387 = Path To String(path=w1326) -> (string=w1325:string)
                n388 = call "settings_save_to_file.vi"("XML File Path"=w1326) -> ()  [unwired: 11 in]
                n389 = call "settings_filename_to_registry.vi"("Last Used Settings File"=w1325) -> ()  [unwired: 11 in]
              }
            }
          }
          frame "LoadStateFromFile" {
            # "Load a file, and use it to reset the values of all the front panel controls."
            # "We need to re-run the initialisation stuff in UDP sender after changing settings\n(for example, this synchronises the settings like camera pixel size with the\nrelevant global variable)"
            n390 = call "File Dialog2"("prompt"="Please select a settings file", "button label"="Open", "default name"="red_tweezers_settings.xml", "pattern (all files)"="*.xml" ("pattern label"), "pattern label"="XML Settings Files") -> ("selected path"=w1339:path, "cancelled"=w1346:bool)  [unwired: 7 in, 2 out]
            n391 = Not(x=w1346) -> (.not. x?=w1345:bool)
            n392 = case shown="False" w1345 {
              selector: w1345 -> [w1348 w1349]
              tunnel: w1339 -> [_ w1350]
              tunnel: [w1348 w1349] -> w1337
              frame False {
              }
              frame True {
                n393 = call "settings_load_from_file.vi"("XML File Path"=w1350) -> ()  [unwired: 9 in, 2 out]
                n394 = Path To String(path=w1350) -> (string=w1351:string)
                n395 = call "settings_filename_to_registry.vi"("Last Used Settings File"=w1351) -> ()  [unwired: 11 in]
              }
            }
            n396 = call "UDP Sender generic_2.vi"("re-initialise"=w1337, "Spots"=w1338) -> ()  [unwired: 1 in, 1 out]
          }
          frame "Undo" {
            # "This should get the last undo vector and replace the spots with it :)"
            n397 = call "red_tweezers_UNDO.vi"("Selection/Group"=w1356, "Undo/Store (store, False)"=TRUE, "Spots"=w1357) -> ("Selection/Group Out (Undo only)"=w1354:T8[], "Spots Out (Undo only)"=w1355:T2[])  [unwired: 7 in]
          }
          frame "Delete" {
            n398 = call "delete_selected_spots.vi"("Selection/Group 3"=w1360, "Spots 3"=w1361) -> ("Selection/Group 2"=w1359:T8[], "Spots 2"=w1358:T2[])  [unwired: 4 in]
          }
          frame "SelectAllSpots" {
            n399 = for {
              tunnel: w1362 -> [w1367] mode=indexing
              tunnel: [w1368] -> w1363 mode=indexing
              n400 = Unbundle(w1367) -> ("Group ID"=w1366:i32)  [unwired: 1 out]
              n401 = Bundle(cluster=w1367, "Group ID"=w1366, "Selected"=TRUE ("Label.Visible")) -> (w1368:T8)
            }
          }
          frame "SelectNoSpots" {
            n402 = for {
              tunnel: w1369 -> [w1374] mode=indexing
              tunnel: [w1375] -> w1370 mode=indexing
              n403 = Unbundle(w1374) -> ("Group ID"=w1373:i32)  [unwired: 1 out]
              n404 = Bundle(cluster=w1374, "Group ID"=w1373, "Selected"=FALSE ("Label.Visible")) -> (w1375:T8)
            }
          }
          frame "SelectSpecificSpots" {
            n405 = call "select_by_id.vi"("Selection/Group"=w1377, "Spots"=w1378) -> ("Selection/Group Out"=w1376:T8[])  [unwired: 9 in]
          }
          frame "Group" {
            # "Group the currently selected spots"
            n406 = call "group_selected_spots.vi"("Selection/Group 2"=w1379) -> ("Array"=w1381:T8[])
          }
          frame "Ungroup" {
            # "Ungroup the currently selected spots"
            n407 = for {
              tunnel: [w1388] -> w1384 mode=indexing
              tunnel: w1382 -> [w1387] mode=indexing
              tunnel: 0 -> [w1386]
              n408 = Unbundle(w1387) -> ("Selected"=w1389:bool)  [unwired: 1 out]
              n409 = case shown="False" w1389 {
                tunnel: [w1390 w1393] -> w1388
                tunnel: w1387 -> [w1390 w1392]
                tunnel: w1386 -> [_ w1391]
                frame False {
                }
                frame True {
                  n410 = Unbundle(w1392) -> ("Selected"=w1394:bool)  [unwired: 1 out]
                  n411 = Bundle(cluster=w1392, "Group ID"=w1391, "Selected"=w1394) -> (w1393:T8)
                }
              }
            }
          }
          frame "ZoomIn" {
            w1395 = "ZoomToFit" ("item tag")
            # "turn off \"zoom to fit\""
            n412 = property class="ImageControl"(reference=w1410) -> (reference out=w1404:refnum<vi>, "ZoomSingle"=w1409:cluster{"X":sgl, "Y":sgl}, "Image Center Position"=w1402:cluster{"X":u32, "Y":u32})  [unwired: 1 in, 1 out]
            n413 = Unbundle(w1409) -> ("X"=w1407:sgl)  [unwired: 1 out]
            n414 = Round To Nearest(number=w1407) -> (nearest integer value=w1403:sgl)
            n415 = Greater Than 0?(x=w1403) -> (x > 0?=w1408:bool)
            n416 = case shown="True" w1408 {
              tunnel: w1407 -> [w1417 w1420]
              tunnel: [w1416 w1418] -> w1406
              frame False {
                n417 = Reciprocal(x=w1417) -> (1/x=w1414:sgl)
                n418 = Round Toward +Infinity(x=w1414) -> (ceil(x): smallest int >= x=w1415:sgl)
                n419 = Decrement(x=w1415) -> (x-1=w1413:sgl)
                n420 = Reciprocal(x=w1413) -> (1/x=w1416:sgl)
              }
              frame True {
                n421 = Round Toward -Infinity(1:w1420) -> (0:w1419:sgl)
                n422 = Increment(x=w1419) -> (x+1=w1418:sgl)
              }
            }
            n423 = Bundle(w1406, w1406) -> (w1405:cluster{sgl, sgl})  [unwired: 1 in]
            n424 = property class="ImageControl"(reference=w1404, "ZoomSingle"=w1405, "Image Center Position"=w1402) -> ()  [unwired: 1 in, 2 out]
            n425 = Get Menu Item Info(7:w1395, 11:w1401) -> (1:w1398:bool, 2:w1399:string, 3:w1400:refnum<k9>, 6:w1397:T21)  [unwired: 1 in, 3 out]
            n426 = Set Menu Item Info(4:w1397, 6:FALSE ("checked"), 7:w1395, 9:w1398, 10:w1399, 11:w1400) -> ()  [unwired: 1 in, 2 out]
          }
          frame "ZoomOut" {
            w1424 = "ZoomToFit" ("item tag")
            # "turn off \"zoom to fit\""
            n427 = property class="ImageControl"(reference=w1436) -> (reference out=w1432:refnum<vi>, "ZoomSingle"=w1435:cluster{"X":sgl, "Y":sgl}, "Image Center Position"=w1431:cluster{"X":u32, "Y":u32})  [unwired: 1 in, 1 out]
            n428 = Unbundle(w1435) -> ("X"=w1421:sgl)  [unwired: 1 out]
            n429 = Greater?(x=w1421, y=1.0) -> (0:w1423:bool)
            n430 = case shown="False" w1423 {
              tunnel: w1421 -> [w1445 w1448]
              tunnel: [w1444 w1446] -> w1434
              frame False {
                n431 = Reciprocal(x=w1445) -> (1/x=w1442:sgl)
                n432 = Add(x=w1442, y=sgl 0.01 ("x")) -> (x+y=w1440:sgl)
                n433 = Round Toward -Infinity(1:w1440) -> (0:w1443:sgl)
                n434 = Increment(x=w1443) -> (x+1=w1441:sgl)
                n435 = Reciprocal(x=w1441) -> (1/x=w1444:sgl)
              }
              frame True {
                n436 = Round Toward +Infinity(x=w1448) -> (ceil(x): smallest int >= x=w1447:sgl)
                n437 = Decrement(x=w1447) -> (x-1=w1446:sgl)
              }
            }
            n438 = Bundle(w1434, w1434) -> (w1433:cluster{sgl, sgl})  [unwired: 1 in]
            n439 = property class="ImageControl"(reference=w1432, "ZoomSingle"=w1433, "Image Center Position"=w1431) -> ()  [unwired: 1 in, 2 out]
            n440 = Get Menu Item Info(7:w1424, 11:w1430) -> (1:w1427:bool, 2:w1428:string, 3:w1429:refnum<k9>, 6:w1426:T21)  [unwired: 1 in, 3 out]
            n441 = Set Menu Item Info(4:w1426, 6:FALSE ("checked"), 7:w1424, 9:w1427, 10:w1428, 11:w1429) -> ()  [unwired: 1 in, 2 out]
          }
          frame "ZoomToFit" {
            w1454 = "ZoomToFit" ("item tag")
            # "and make sure the image obeys the result"
            # "Toggle menu checkmark"
            n442 = Get Menu Item Info(7:w1454, 11:w1453) -> (1:w1452:bool, 2:w1456:string, 3:w1457:refnum<k9>, 4:w1451:bool, 6:w1455:T21)  [unwired: 1 in, 2 out]
            n443 = Not(x=w1451) -> (.not. x?=w1449:bool)
            n444 = Set Menu Item Info(4:w1455, 6:w1449, 7:w1454, 9:w1452, 10:w1456, 11:w1457) -> ()  [unwired: 1 in, 2 out]
            n445 = property class="ImageControl"(reference=w1450, "Zoom to Fit Mode"=w1449) -> ()  [unwired: 1 in, 2 out]
          }
          frame "ShowGrid" {
            w1465 = "ShowGrid" ("item tag")
            # "Toggle menu checkmark"
            n446 = Get Menu Item Info(7:w1465, 11:w1464) -> (1:w1463:bool, 2:w1467:string, 3:w1468:refnum<k9>, 4:w1462:bool, 6:w1466:T21)  [unwired: 1 in, 2 out]
            n447 = Not(x=w1462) -> (.not. x?=w1461:bool)
            n448 = Set Menu Item Info(4:w1466, 6:w1461, 7:w1465, 9:w1463, 10:w1467, 11:w1468) -> ()  [unwired: 1 in, 2 out]
            n449 = call "grid_and_guides.vi"("Boolean"=w1461, "Operation"=T14."Set grid visibility") -> ()  [unwired: 9 in, 1 out]
          }
          frame "ShowGuides" {
            w1476 = "ShowGuides" ("item tag")
            # "Toggle menu checkmark"
            n450 = Get Menu Item Info(7:w1476, 11:w1475) -> (1:w1474:bool, 2:w1478:string, 3:w1479:refnum<k9>, 4:w1473:bool, 6:w1477:T21)  [unwired: 1 in, 2 out]
            n451 = Not(x=w1473) -> (.not. x?=w1472:bool)
            n452 = Set Menu Item Info(4:w1477, 6:w1472, 7:w1476, 9:w1474, 10:w1478, 11:w1479) -> ()  [unwired: 1 in, 2 out]
            n453 = call "grid_and_guides.vi"("Boolean"=w1472, "Operation"=T14."Set guide visibility") -> ()  [unwired: 9 in, 1 out]
          }
          frame "ConfigureGridAndGuides" {
            n454 = call "grid_and_guides.vi"("Operation"=T14."Show front panel") -> ()  [unwired: 10 in, 1 out]
          }
          frame "ShowSettings" {
            n455 = call "UDP Sender generic_2.vi"("Show panel"=TRUE, "Spots"=w1486) -> ()  [unwired: 1 in, 1 out]
          }
          frame "CameraSettings" {
            n456 = global read "red_tweezers_globals_INTERNAL_VOLATILE.vi" "Current Camera VI"() -> (w1489:path)
            n457 = Open VI Reference(vi path=w1489) -> (vi reference=w1488:refnum<vi>)  [unwired: 5 in, 1 out]
            n458 = property class="VI"(reference=w1488, "Front Panel.Open"=TRUE ("Front Panel Window:Open")) -> ()  [unwired: 1 in, 2 out]
          }
          frame Default {
          }
        }
      }
      event Mouse Down? {
        # "We don't process clicks when the user is on the video tab, so that we can set ROIs."
        # "When the mouse button goes down over the image, we save where it went down, etc. and wait to see what happens next.  We also register to be told when the mouse leaves the control, goes up, or moves.  \"click\" or \"drag\" are only detected once the mouse moves or goes up."
        n459 = event-data() -> ("Coords"=w1509:T22, "Button"=w1504:u16, "Mods"=w1513:cluster{"Double Click":bool, "Menu Key":bool}, "PlatMods"=w1512:T23)  [unwired: 1 in]
        n460 = call "mouse_to_image_coords.vi"("Mouse Coords (screen/pane units)"=w1509, "Image Control"=w1505) -> ("Cursor is on Display Area"=w1503:bool, "Mouse Coords (image pixels)"=w1508:cluster{dbl, dbl})  [unwired: 4 in]
        n461 = disable-structure shown="Enabled" {
          disable-tunnel: w1504 -> [w1521 _]
          disable-tunnel: w1503 -> [w1519 w1522]
          disable-tunnel: [w1518 w1522] -> w1499
          frame Enabled {
            n462 = Equal?(x=u16 1, y=w1521) -> (x = y?=w1520:bool)
            n463 = And(x=w1519, y=w1520) -> (x .and. y?=w1518:bool)
          }
          frame Disabled {
            # "use other pane to allow right-clicking on image"
          }
        }
        n464 = local read "Tab"() -> (w1500:T5)
        n465 = Not Equal?(x=w1500, y=T15."Video" ("Tab")) -> (x != y?=w1498:bool)
        n466 = And(x=w1499, y=w1498) -> (x .and. y?=w1497:bool)
        n467 = case shown="False" w1497 {
          tunnel: w1516 -> [w1525 w1536]
          tunnel: [T11 {"Button Down"=FALSE, "Dragging"=FALSE, "Position (Image Pixels)"={"X"=0.0, "Y"=0.0}, "Previous Position (Image Pixels)"={"X"=0.0, "Y"=0.0}, "Button"=0, "Mods"={"Double Click"=FALSE, "Menu Key"=FALSE}, "PlatMods"={"Shift"=FALSE, "Ctrl"=FALSE, "Alt"=FALSE, "Cmd"=FALSE, "Opt"=FALSE}} w1535] -> w1515
          tunnel: [w1525 w1532] -> w1514
          tunnel: w1504 -> [_ w1531]
          tunnel: w1513 -> [_ w1530]
          tunnel: w1512 -> [_ w1529]
          tunnel: w1508 -> [_ w1528]
          tunnel: [FALSE TRUE] -> w1507
          tunnel: w1505 -> [_ w1526]
          frame False {
            # "If the user clicked on a scrollbar, ignore it and let LabVIEW handle it. (this keeps the scrollbars working)"
          }
          frame True {
            w1534 = FALSE  # Dragging
            w1533 = TRUE  # Button Down
            n468 = register-events(reference=w1536, w1526, w1526, w1526, w1526) -> (reference out=w1532:refnum<event-registration>)  [unwired: 1 in, 1 out]
            n469 = Bundle("Button Down"=w1533, "Dragging"=w1534, "Mouse Coords (image pixels)"=w1528, "Mouse Coords (image pixels)"=w1528, "Button"=w1531, "Mods"=w1530, "PlatMods"=w1529) -> (w1535:T24)  [unwired: 1 in]
          }
        }
        n470 = Array Size(array=w1495) -> (size(s)=w1496:i32)
        n471 = local write "# of Spots"(w1496) -> ()
        n472 = local write "Selection/Group"(w1495) -> ()
        n473 = event-data("Discard?"=w1507) -> ()  [unwired: 4 in, 1 out]
      }
      event Mouse Leave {
        w1543 = refnum<vi> refnum  # Dummy
        # "When the mouse leaves, we reset things."
        n474 = event-data() -> ()  [unwired: 1 in, 2 out]
        n475 = register-events(reference=w1544, w1542, w1543, w1543, w1543) -> (reference out=w1541:refnum<event-registration>)  [unwired: 1 in, 1 out]
      }
      event Mouse Up {
        w1563 = refnum<vi> refnum  # Dummy
        # "Double clicking adds a spot at the mouse position."
        # "deregister"
        # "If we get here the mouse has gone down and up again.  If we've not moved in between, we have a Click.\nEither way we're no longer interested in mouse leave/move/up events."
        n476 = event-data() -> ("Mods"=w1550:cluster{"Double Click":bool, "Menu Key":bool})  [unwired: 1 in, 5 out]
        n477 = Unbundle By Name(w1556) -> ("Dragging"=w1565:bool)
        n478 = Unbundle By Name(w1550) -> ("Double Click"=w1547:bool)
        n479 = Not(x=w1565) -> (.not. x?=w1564:bool)
        n480 = Not(x=w1552) -> (.not. x?=w1554:bool)
        n481 = And(x=w1564, y=w1554) -> (x .and. y?=w1548:bool)
        n482 = case shown="True" w1548 {
          tunnel: w1556 -> [_ w1571]
          tunnel: w1558 -> [w1566 w1570]
          tunnel: w1557 -> [w1567 w1573]
          tunnel: [w1567 w1572] -> w1559
          tunnel: w1547 -> [_ w1568]
          tunnel: [w1566 w1569] -> w1549
          frame False {
          }
          frame True {
            n483 = case shown="True" w1568 {
              tunnel: w1573 -> [w1580 w1630]
              tunnel: [w1578 w1636] -> w1572
              tunnel: w1570 -> [w1574 w1637]
              tunnel: w1571 -> [w1577 w1632]
              tunnel: [w1574 w1628] -> w1569
              frame False {
                w1584 = 400.0  # 20^2 px
                # "If the user clicked, determine which spots should be selected: if we've clicked a spot/group then select it.  Shift-clicking toggles selection for that spot, and leaves the rest of the selection unchanged."
                # "check we're close enough"
                # "find closest"
                n484 = Unbundle By Name(w1577) -> ("Position (Image Pixels)"=w1576:cluster{"X":dbl, "Y":dbl}, "PlatMods.Shift"=w1575:bool)
                n485 = for {
                  tunnel: [w1620] -> w1582 mode=indexing
                  tunnel: w1576 -> [w1619]
                  tunnel: w1574 -> [w1618] mode=indexing
                  # "calculate distances between mouse position and spot positions"
                  n486 = call "extract_position.vi"("Spot"=w1618) -> ("Position"=w1617:cluster{"x":dbl, "y":dbl, "z":dbl})
                  n487 = call "coords_real_to_image_currentview.vi"("Position (real coords)"=w1617) -> ("Position (pixels, relative to the top left of the image)"=w1616:cluster{dbl, dbl})  [unwired: 7 in, 1 out]
                  n488 = Subtract(x=w1616, y=w1619) -> (x-y=w1623:cluster{dbl, dbl})
                  n489 = Multiply(x=w1623, y=w1623) -> (x*y=w1622:cluster{dbl, dbl})
                  n490 = Cluster To Array(cluster=w1622) -> (array=w1621:dbl[])
                  n491 = Add Array Elements(numeric array=w1621) -> (sum=w1620:dbl)
                }
                n492 = Array Max & Min(array=w1582) -> (min value=w1583:dbl, min index (indices)=w1579:i32)  [unwired: 2 out]
                n493 = Less Or Equal?(x=w1583, y=w1584) -> (x <= y?=w1581:bool)
                n494 = case shown="True" w1581 {
                  tunnel: w1580 -> [w1585 w1592]
                  tunnel: w1579 -> [_ w1586]
                  tunnel: w1575 -> [_ w1588]
                  tunnel: [w1585 w1587] -> w1578
                  frame False {
                    # "If we didn't click a spot, do nothing."
                  }
                  frame True {
                    # "If the spot is in a group, act on all spots in that group, not just the spot we clicked."
                    # "This case statement toggles the selection of the spot/group we clicked, and leaves other spots unchanged if we're holding shift.  Otherwise, we select the spot/group that was clicked and deselect everything else."
                    n495 = stacked-sequence {
                      tunnel: w1586 -> [_ w1594]
                      frame #0 {
                        n496 = local read "Current Spot #"() -> (→"Prev Current Spot":dbl)
                      }
                      frame #1 {
                        "Current Spot #" <- w1594
                      }
                    }
                    n497 = Index Array(array=w1592, index=w1586) -> (element=w1591:T8)
                    n498 = Unbundle(w1591) -> ("Group ID"=w1589:i32)  [unwired: 1 out]
                    n499 = Greater Than 0?(x=w1589) -> (x > 0?=w1590:bool)
                    n500 = for {
                      tunnel: w1592 -> [w1605] mode=indexing
                      tunnel: w1590 -> [w1602]
                      tunnel: w1589 -> [w1601]
                      tunnel: w1586 -> [w1600]
                      tunnel: w1588 -> [w1598]
                      tunnel: [w1596] -> w1587 mode=indexing
                      i -> [w1599]
                      n501 = Unbundle(w1605) -> ("Group ID"=w1595:i32, "Selected"=w1603:bool)
                      n502 = case shown="True" w1602 {
                        tunnel: w1595 -> [_ w1609]
                        tunnel: [w1607 w1611] -> w1597
                        tunnel: w1601 -> [_ w1610]
                        tunnel: w1600 -> [w1608 _]
                        tunnel: w1599 -> [w1606 _]
                        frame False {
                          n503 = Equal?(x=w1606, y=w1608) -> (x = y?=w1607:bool)
                        }
                        frame True {
                          n504 = Equal?(x=w1609, y=w1610) -> (x = y?=w1611:bool)
                        }
                      }
                      n505 = case shown="True" w1598 {
                        tunnel: [w1612 w1613] -> w1604
                        tunnel: w1603 -> [_ w1614]
                        tunnel: w1597 -> [w1612 w1615]
                        frame False {
                        }
                        frame True {
                          n506 = Exclusive Or(1:w1615, 2:w1614) -> (0:w1613:bool)
                        }
                      }
                      n507 = Bundle("Group ID"=w1595, w1604) -> (w1596:cluster{"Group ID":i32, bool})  [unwired: 1 out]
                    }
                  }
                }
              }
              frame True {
                # "convert mouse position to real coords, and add a spot there."
                # "Double-click detected"
                n508 = Unbundle By Name(w1632) -> ("Position (Image Pixels)"=w1631:cluster{"X":dbl, "Y":dbl})
                n509 = for {
                  tunnel: w1630 -> [w1640] mode=indexing
                  tunnel: [w1639] -> w1629 mode=indexing
                  n510 = Bundle(cluster=w1640, "Selected"=FALSE) -> (w1639:T8)  [unwired: 1 in]
                }
                n511 = call "coords_image_to_real_currentimage.vi"("Position (pixels on image)"=w1631) -> ("Position (real coords)"=w1633:cluster{dbl, dbl, "Z":dbl})  [unwired: 9 in]
                n512 = call "replace_position.vi"("Position"=w1633) -> ("Spot"=w1635:T2)  [unwired: 3 in]
                n513 = Build Array (concatenate)(w1637, w1635) -> (w1628:T2[])
                n514 = Build Array (concatenate)(w1629, T8 {"Group ID"=0, "Selected"=TRUE} ("selection_element")) -> (w1636:T8[])
                n515 = Array Size(array=w1628) -> (size(s)=w1627:i32)
                n516 = local write "Induce check"(TRUE) -> ()
                n517 = Subtract(x=w1627, y=1) -> (x-y=w1626:i32)
                n518 = local write "Current Spot #"(w1626) -> ()
              }
            }
          }
        }
        n519 = register-events(reference=w1561, w1560, w1563, w1563, w1563) -> (reference out=w1562:refnum<event-registration>)  [unwired: 1 in, 1 out]
      }
      event Mouse Move {
        n520 = event-data() -> ("Coords"=w1655:T22)  [unwired: 1 in, 2 out]
        n521 = call "mouse_to_image_coords.vi"("Mouse Coords (screen/pane units)"=w1655, "Image Control"=w1654) -> ("Mouse Coords (image pixels)"=w1646:cluster{dbl, dbl})  [unwired: 4 in, 1 out]
        n522 = Not(x=w1645) -> (.not. x?=w1650:bool)
        n523 = case shown="True" w1650 {
          tunnel: w1648 -> [_ w1668]
          tunnel: w1653 -> [w1660 w1670]
          tunnel: w1652 -> [w1659 w1669]
          tunnel: [w1659 w1669] -> w1641
          tunnel: [w1660 w1671] -> w1651
          tunnel: w1646 -> [_ w1662]
          tunnel: w1642 -> [_ w1661]
          frame False {
          }
          frame True {
            # "this is the displacement of the mouse, since the last iteration, in \"real\" coordinates (NB the conversions go before subtracting, as it may involve adding a constant as well as multiplying, which would confuse things as we're only interested in displacements here."
            # "The \"position\" local variable is there just in case we're on the \"current spot\" tab, so that the position updates nicely"
            # "If the user is dragging, translate the spots.\nHolding down shift causes the mouse's motion to be transformed into scaling about the centroid of the spots and rotation about the same point"
            n524 = Unbundle By Name(w1668) -> ("Position (Image Pixels)"=w1663:cluster{"X":dbl, "Y":dbl})
            n525 = call "find_centroid.vi"("Selection and Groups"=w1669, "Spots"=w1670) -> ("centroid"=w1664:cluster{"x":dbl, "y":dbl, "z":dbl})  [unwired: 2 in, 4 out]
            n526 = Unbundle By Name(w1668) -> ("PlatMods.Shift"=w1667:bool)
            n527 = disable-structure shown="Disabled" {
              disable-tunnel: w1664 -> [w1672 _]
              frame Disabled {
                n528 = local write "Position"(w1672) -> ()
              }
              frame Enabled {
              }
            }
            n529 = call "coords_image_to_real_currentimage.vi"("Position (pixels on image)"=w1662) -> ("Position (real coords)"=w1665:cluster{dbl, dbl, "Z":dbl})  [unwired: 9 in]
            n530 = call "coords_image_to_real_currentimage.vi"("Position (pixels on image)"=w1663) -> ("Position (real coords)"=w1666:cluster{dbl, dbl, "Z":dbl})  [unwired: 9 in]
            n531 = case shown="False" w1667 {
              tunnel: [w1677 w1951] -> w1671
              tunnel: w1670 -> [w1683 w1952]
              tunnel: w1669 -> [w1682 w1950]
              tunnel: w1666 -> [w1681 w1937]
              tunnel: w1664 -> [_ w1947]
              tunnel: w1665 -> [w1678 w1938]
              tunnel: w1661 -> [_ _]
              frame False {
                # "Spot Checker passes on information for the bubble collision,system so proper calculations can be made."
                n532 = while {
                  tunnel: w1681 -> [w1722]
                  tunnel: [w1712] -> w1679
                  tunnel: w1678 -> [w1711]
                  i -> [w1705]
                  stop <- w1707 stop-if-true
                  w1697 = 0
                  # "This while loop statement makes sure\nthat every spot gets checked before \nallowing any spot to move."
                  # "Buffer zone controls the amount of space between the\ncenter of a spot compared to the center of another spot.\nThis is used to prevent bubbles from colliding with each other."
                  # "Projected distance calculates the distance between two spots- this is used for when a \"hit\" occurs. If the projected distance becomes larger than the previous distance, the program will assume that the spot is being pulled from the buffer zone and as a result will allow the bubble to exit."
                  # "This subVI leads to the distance function, which outputs the distance between a spot being checked compared to the current spot number."
                  n533 = control-ref of="Value Check"() -> (w1702:refnum<vi>)
                  n534 = control-ref of="ID num check"() -> (w1701:refnum<vi>)
                  n535 = control-ref of="Spot Checker"() -> (w1718:refnum<vi>)
                  n536 = Subtract(x=w1711, y=w1722) -> (x-y=w1712:cluster{dbl, dbl, "Z":dbl})
                  n537 = call "DistanceFunction.vi"("Condition Driver"=FALSE, "Position (real coords)"=w1722, "Current Spot Number"=w1701, "Spot Checker"=w1718, "Spot Number Being Checked"=w1702) -> ("Distance"=w1686:dbl)  [unwired: 6 in]
                  n538 = stacked-sequence {
                    tunnel: w1686 -> [_ w1727]
                    frame #0 {
                      n539 = local read "Distance"() -> (→"Previous Distance":dbl)
                    }
                    frame #1 {
                      "Distance" <- w1727
                    }
                  }
                  n540 = Unbundle(w1712) -> (→"X Displacement":dbl, →"Y Displacement":dbl)  [unwired: 1 out]
                  n541 = control-ref of="ID num check"() -> (w1703:refnum<vi>)
                  n542 = control-ref of="Spot Checker"() -> (w1716:refnum<vi>)
                  n543 = control-ref of="Y Displacement"() -> (w1714:refnum<vi>)
                  n544 = control-ref of="Value Check"() -> (w1704:refnum<vi>)
                  n545 = control-ref of="X Displacement"() -> (w1715:refnum<vi>)
                  n546 = call "ProjectedDistance.vi"("X Displacement"=w1715, "Spot Number Check"=w1704, "Current Spot #"=w1703, "Spot Checker"=w1716, "Y Displacement"=w1714) -> ("Numeric"=→"Projected Distance":dbl)  [unwired: 6 in]
                  n547 = Multiply(x="Buffer Zone", y=2) -> (x*y=w1721:dbl)
                  n548 = local read "ID num check"() -> (w1698:dbl)
                  n549 = local read "Value Check"() -> (w1699:dbl)
                  n550 = local read "Projected Distance"() -> (w1690:dbl)
                  n551 = Equal?(x=w1686, y=0) -> (x = y?=w1687:bool)
                  n552 = case shown="False" w1687 {
                    frame False {
                      n553 = local read "Hit"() -> (w1724:bool)
                      n554 = local write "Hit Indicator"(w1724) -> ()
                    }
                    frame True {
                      "Hit Indicator" <- FALSE
                    }
                  }
                  n555 = Not Equal?(x=w1690, y=0) -> (x != y?=w1688:bool)
                  n556 = Less Or Equal?(x=w1686, y=w1721) -> (x <= y?=w1691:bool)
                  n557 = Equal?(x=w1698, y=w1697) -> (x = y?=w1696:bool)
                  n558 = And(x=w1691, y=w1688) -> (x .and. y?=w1684:bool)
                  "Hit" <- w1684
                  n559 = Equal?(x=w1697, y=w1699) -> (x = y?=w1695:bool)
                  n560 = Not(x=w1684) -> ()  [unwired: 1 out]
                  n561 = And(x=w1696, y=w1695) -> (x .and. y?=w1694:bool)
                  n562 = Or(x=w1684, y=w1694) -> (x .or. y?=w1700:bool)
                  n563 = case shown="False" w1700 {
                    frame False {
                      n564 = stacked-sequence {
                        frame #0 {
                          n565 = local read "Potential Collisions"() -> (w1730:dbl)
                          n566 = local read "Spot # Check"() -> (w1732:dbl)
                          n567 = Subtract(x=w1730, y=1) -> (x-y=w1728:dbl)
                          n568 = Less Or Equal?(x=w1732, y=w1728) -> (x <= y?=w1731:bool)
                          n569 = case shown="True" w1731 {
                            frame False {
                              # "Spot # Check resets if the the number of potential collisons is more than Spot # Check."
                              n570 = local write "Spot # Check"(0) -> ()
                            }
                            frame True {
                              n571 = stacked-sequence {
                                frame #0 {
                                # "Spot # Check increments by 1 every time it is greater than the # of potential collisions."
                                n572 = local read "Spot # Check"() -> (w1736:dbl)
                                n573 = Add(x=w1736, y=1) -> (x+y=→"Spot # Check":dbl)
                                }
                                frame #1 {
                                # "Spot # Check resets if the Spot # Check is eqaul to the # of potential collisions."
                                n574 = local read "Potential Collisions"() -> (w1737:dbl)
                                n575 = local read "Spot # Check"() -> (w1738:dbl)
                                n576 = Equal?(x=w1738, y=w1737) -> (x = y?=w1739:bool)
                                n577 = case shown="True" w1739 {
                                frame False {
                                }
                                frame True {
                                n578 = local write "Spot # Check"(0) -> ()
                                }
                                }
                                }
                                frame #2 {
                                n579 = local read "Spot Checker"() -> (w1754:T2[])
                                n580 = local read "Current Spot #"() -> (w1755:dbl)
                                n581 = local read "Area to check"() -> (w1741:dbl)
                                n582 = Index Array(array=w1754, index=w1755) -> (element=w1753:T2)
                                n583 = local read "Orig Y SC"() -> (w1750:dbl)
                                n584 = Unbundle By Name(w1753) -> ("Position.x"=w1751:dbl, "Position.y"=w1749:dbl)
                                n585 = local read "Orig X SC"() -> (w1752:dbl)
                                n586 = Subtract(x=w1749, y=w1750) -> (x-y=w1742:dbl)
                                n587 = Absolute Value(x=w1742) -> (abs(x)=w1743:dbl)
                                n588 = Subtract(x=w1751, y=w1752) -> (x-y=w1745:dbl)
                                n589 = Greater?(x=w1743, y=w1741) -> (0:w1747:bool)
                                n590 = Absolute Value(x=w1745) -> (abs(x)=w1744:dbl)
                                n591 = Greater?(x=w1744, y=w1741) -> (0:w1746:bool)
                                n592 = Or(x=w1746, y=w1747) -> (x .or. y?=w1748:bool)
                                n593 = case shown="True" w1748 {
                                frame False {
                                }
                                frame True {
                                n594 = stacked-sequence {
                                frame #0 {
                                n595 = local read "Null array"() -> (w1760:dbl[])
                                n596 = local write "What to Check"(w1760) -> ()
                                n597 = local write "ID"(w1760) -> ()
                                n598 = local read "Current Spot #"() -> (w1762:dbl)
                                n599 = local write "Potential Collisions"(0) -> ()
                                n600 = local read "Spot Checker"() -> (w1761:T2[])
                                n601 = Index Array(array=w1761, index=w1762) -> (element=w1763:T2)
                                n602 = Wait (ms)(milliseconds to wait=100) -> ()  [unwired: 1 out]
                                n603 = Unbundle By Name(w1763) -> ("Position.x"=w1757:dbl, "Position.y"=w1758:dbl)
                                n604 = local write "Orig Y SC"(w1758) -> ()
                                n605 = local write "Orig X SC"(w1757) -> ()
                                }
                                frame #1 {
                                # "All this is a  statement checking whether the microrobot is within the area being checked using absolute value statements. The number of potential collisions gets added by 1 every time a bubble is detected within the area."
                                n606 = local read "# of Spots"() -> (w1764:dbl)
                                n607 = for {
                                N: w1764 -> [_]
                                tunnel: w1764 -> [w1769]
                                i -> [w1765]
                                n608 = local read "Selection/Group"() -> (w1768:T8[])
                                n609 = Index Array(array=w1768, index=w1765) -> (element=w1767:T8)
                                n610 = Unbundle By Name(w1767) -> ("Selected"=w1766:bool)
                                n611 = case shown="True" w1766 {
                                tunnel: w1769 -> [_ w1771]
                                tunnel: w1765 -> [_ w1770]
                                frame False {
                                }
                                frame True {
                                n612 = for {
                                N: w1771 -> [_]
                                tunnel: w1770 -> [w1772]
                                i -> [w1773]
                                n613 = local read "Selection/Group"() -> (w1777:T8[])
                                n614 = Index Array(array=w1777, index=w1773) -> (element=w1776:T8)
                                n615 = Unbundle By Name(w1776) -> ("Selected"=w1774:bool)
                                n616 = Not(x=w1774) -> (.not. x?=w1775:bool)
                                n617 = case shown="True" w1775 {
                                tunnel: w1773 -> [_ w1781]
                                tunnel: w1772 -> [_ w1780]
                                tunnel: w1772 -> [_ w1779]
                                frame False {
                                }
                                frame True {
                                n618 = local read "Spot Checker"() -> (w1798:T2[])
                                n619 = Index Array(array=w1798, index=w1781) -> (element=w1799:T2)
                                n620 = Index Array(array=w1798, index=w1780) -> (element=w1797:T2)
                                n621 = Unbundle By Name(w1797) -> ("Position.x"=w1794:dbl, "Position.y"=w1790:dbl)
                                n622 = Unbundle By Name(w1799) -> ("Position.x"=w1791:dbl, "Position.y"=w1787:dbl)
                                n623 = local read "Area+ Buffer"() -> (w1778:dbl)
                                n624 = Subtract(x=w1794, y=w1778) -> (x-y=w1795:dbl)
                                n625 = Greater Or Equal?(x=w1791, y=w1795) -> (x >= y?=w1796:bool)
                                n626 = Add(x=w1790, y=w1778) -> (x+y=w1789:dbl)
                                n627 = Subtract(x=w1790, y=w1778) -> (x-y=w1788:dbl)
                                n628 = Add(x=w1794, y=w1778) -> (x+y=w1792:dbl)
                                n629 = Less Or Equal?(x=w1787, y=w1789) -> (x <= y?=w1786:bool)
                                n630 = Greater Or Equal?(x=w1787, y=w1788) -> (x >= y?=w1785:bool)
                                n631 = Less Or Equal?(x=w1791, y=w1792) -> (x <= y?=w1793:bool)
                                n632 = And(x=w1796, y=w1793) -> (x .and. y?=w1783:bool)
                                n633 = And(x=w1786, y=w1785) -> (x .and. y?=w1784:bool)
                                n634 = And(x=w1783, y=w1784) -> (x .and. y?=w1782:bool)
                                n635 = case shown="True" w1782 {
                                tunnel: w1781 -> [_ _]
                                tunnel: w1781 -> [_ w1801]
                                tunnel: w1779 -> [_ w1800]
                                frame False {
                                }
                                frame True {
                                n636 = stacked-sequence {
                                tunnel: w1801 -> [w1802 _]
                                tunnel: w1800 -> [w1803 _]
                                frame #0 {
                                n637 = local read "Potential Collisions"() -> (w1806:dbl)
                                n638 = local read "What to Check"() -> (w1807:dbl[])
                                n639 = Insert Into Array(array=w1807, index=w1806, new element=w1802) -> (w1808:dbl[])
                                n640 = local read "ID"() -> (w1805:dbl[])
                                n641 = local write "What to Check"(w1808) -> ()
                                n642 = Insert Into Array(array=w1805, index=w1806, new element=w1803) -> (w1804:dbl[])
                                n643 = local write "ID"(w1804) -> ()
                                }
                                frame #1 {
                                n644 = local read "Potential Collisions"() -> (w1811:dbl)
                                n645 = Add(x=w1811, y=1) -> (x+y=w1809:dbl)
                                n646 = local write "Potential Collisions"(w1809) -> ()
                                }
                                }
                                }
                                }
                                }
                                }
                                }
                                }
                                }
                                }
                                }
                                frame #2 {
                                n647 = local read "Current Spot #"() -> (w1812:dbl)
                                n648 = local write "Prev Current Spot"(w1812) -> ()
                                }
                                }
                                }
                                }
                                }
                              }
                            }
                          }
                        }
                        frame #1 {
                          # "This updates the ID and Value being checked at the beginning of IDs and values being checked."
                          n649 = local read "Spot # Check"() -> (w1815:dbl)
                          n650 = local read "What to Check"() -> (w1816:dbl[])
                          n651 = local read "ID"() -> (w1817:dbl[])
                          n652 = Index Array(array=w1817, index=w1815) -> (element=w1814:dbl)
                          n653 = Index Array(array=w1816, index=w1815) -> (element=w1813:dbl)
                          n654 = local write "Value Check"(w1813) -> ()
                          n655 = local write "ID num check"(w1814) -> ()
                        }
                      }
                    }
                    frame True {
                      n656 = stacked-sequence {
                        frame #0 {
                          # "This section activate a case statement which allows us to change the area being checked. Orig X/Y SC holds the position of the area to check and changes after the bubble exits the area beig checked."
                          # "This statement controls the areas selected and finds which bubbles needs to be checked. This activates when the bubble\nmoves out of the area specified."
                          n657 = local read "# of Spots"() -> (w1837:dbl)
                          n658 = local read "Current Spot #"() -> (w1836:dbl)
                          n659 = Subtract(x=w1837, y=1) -> (x-y=w1838:dbl)
                          n660 = Equal?(x=w1836, y=w1838) -> (x = y?=w1834:bool)
                          n661 = case shown="True" w1834 {
                            tunnel: [w1897 w1900] -> w1835
                            frame True {
                              n662 = local read "# of Spots"() -> (w1898:dbl)
                              n663 = Subtract(x=w1898, y=2) -> (x-y=w1897:dbl)
                            }
                            frame False {
                              n664 = local read "# of Spots"() -> (w1899:dbl)
                              n665 = Subtract(x=w1899, y=1) -> (x-y=w1900:dbl)
                            }
                          }
                          "Maximum" <- w1835
                          n666 = local read "Spot Checker"() -> (w1833:T2[])
                          n667 = local read "Current Spot #"() -> (w1832:dbl)
                          n668 = Index Array(array=w1833, index=w1832) -> (element=w1831:T2)
                          n669 = Unbundle By Name(w1831) -> ("Position.x"=w1830:dbl, "Position.y"=w1829:dbl)
                          n670 = local read "Orig Y SC"() -> (w1827:dbl)
                          n671 = local read "Orig X SC"() -> (w1828:dbl)
                          n672 = Subtract(x=w1829, y=w1827) -> (x-y=w1824:dbl)
                          n673 = Subtract(x=w1830, y=w1828) -> (x-y=w1826:dbl)
                          n674 = Absolute Value(x=w1824) -> (abs(x)=w1823:dbl)
                          n675 = Absolute Value(x=w1826) -> (abs(x)=w1825:dbl)
                          n676 = local read "Area to check"() -> (w1819:dbl)
                          n677 = local read "Area to check"() -> (w1818:dbl)
                          n678 = Greater?(x=w1825, y=w1819) -> (0:w1822:bool)
                          n679 = Greater?(x=w1823, y=w1818) -> (0:w1821:bool)
                          n680 = Or(x=w1822, y=w1821) -> (x .or. y?=w1820:bool)
                          n681 = case shown="True" w1820 {
                            frame False {
                            }
                            frame True {
                              n682 = stacked-sequence {
                                frame #0 {
                                # "A small time delay of 100 ms is provided to allow the data to pass throguh properly."
                                n683 = Wait (ms)(milliseconds to wait=100) -> ()  [unwired: 1 out]
                                n684 = local read "Null array"() -> (→"What to Check" →"ID":dbl[])
                                n685 = local read "Spot Checker"() -> (w1845:T2[])
                                n686 = local read "Current Spot #"() -> (w1844:dbl)
                                n687 = Index Array(array=w1845, index=w1844) -> (element=w1843:T2)
                                n688 = Unbundle By Name(w1843) -> ("Position.x"=→"Orig X SC":dbl, "Position.y"=→"Orig Y SC":dbl)
                                "Potential Collisions" <- 0
                                }
                                frame #1 {
                                n689 = local read "# of Spots"() -> (w1848:dbl)
                                n690 = for {
                                N: w1848 -> [_]
                                tunnel: w1848 -> [w1853]
                                i -> [w1849]
                                n691 = local read "Selection/Group"() -> (w1852:T8[])
                                n692 = Index Array(array=w1852, index=w1849) -> (element=w1851:T8)
                                n693 = Unbundle By Name(w1851) -> ("Selected"=w1850:bool)
                                n694 = case shown="True" w1850 {
                                tunnel: w1853 -> [_ w1855]
                                tunnel: w1849 -> [_ w1854]
                                frame False {
                                }
                                frame True {
                                n695 = for {
                                N: w1855 -> [_]
                                tunnel: w1854 -> [w1856]
                                i -> [w1857]
                                n696 = local read "Selection/Group"() -> (w1861:T8[])
                                n697 = Index Array(array=w1861, index=w1857) -> (element=w1860:T8)
                                n698 = Unbundle By Name(w1860) -> ("Selected"=w1858:bool)
                                n699 = Not(x=w1858) -> (.not. x?=w1859:bool)
                                n700 = case shown="True" w1859 {
                                tunnel: w1857 -> [_ w1865]
                                tunnel: w1856 -> [_ w1864]
                                tunnel: w1856 -> [_ w1863]
                                frame False {
                                }
                                frame True {
                                n701 = local read "Spot Checker"() -> (w1882:T2[])
                                n702 = Index Array(array=w1882, index=w1865) -> (element=w1883:T2)
                                n703 = Index Array(array=w1882, index=w1864) -> (element=w1881:T2)
                                n704 = Unbundle By Name(w1881) -> ("Position.x"=w1878:dbl, "Position.y"=w1874:dbl)
                                n705 = Unbundle By Name(w1883) -> ("Position.x"=w1875:dbl, "Position.y"=w1871:dbl)
                                n706 = local read "Area+ Buffer"() -> (w1862:dbl)
                                n707 = Subtract(x=w1878, y=w1862) -> (x-y=w1879:dbl)
                                n708 = Greater Or Equal?(x=w1875, y=w1879) -> (x >= y?=w1880:bool)
                                n709 = Add(x=w1874, y=w1862) -> (x+y=w1873:dbl)
                                n710 = Subtract(x=w1874, y=w1862) -> (x-y=w1872:dbl)
                                n711 = Add(x=w1878, y=w1862) -> (x+y=w1876:dbl)
                                n712 = Less Or Equal?(x=w1871, y=w1873) -> (x <= y?=w1870:bool)
                                n713 = Greater Or Equal?(x=w1871, y=w1872) -> (x >= y?=w1869:bool)
                                n714 = Less Or Equal?(x=w1875, y=w1876) -> (x <= y?=w1877:bool)
                                n715 = And(x=w1880, y=w1877) -> (x .and. y?=w1867:bool)
                                n716 = And(x=w1870, y=w1869) -> (x .and. y?=w1868:bool)
                                n717 = And(x=w1867, y=w1868) -> (x .and. y?=w1866:bool)
                                n718 = case shown="True" w1866 {
                                tunnel: w1865 -> [_ _]
                                tunnel: w1865 -> [_ w1885]
                                tunnel: w1863 -> [_ w1884]
                                frame False {
                                }
                                frame True {
                                n719 = stacked-sequence {
                                tunnel: w1885 -> [w1886 _]
                                tunnel: w1884 -> [w1887 _]
                                frame #0 {
                                n720 = local read "Potential Collisions"() -> (w1890:dbl)
                                n721 = local read "What to Check"() -> (w1891:dbl[])
                                n722 = Insert Into Array(array=w1891, index=w1890, new element=w1886) -> (w1892:dbl[])
                                n723 = local read "ID"() -> (w1889:dbl[])
                                n724 = Insert Into Array(array=w1889, index=w1890, new element=w1887) -> (w1888:dbl[])
                                n725 = local write "What to Check"(w1892) -> ()
                                n726 = local write "ID"(w1888) -> ()
                                }
                                frame #1 {
                                n727 = local read "Potential Collisions"() -> (w1895:dbl)
                                n728 = Add(x=w1895, y=1) -> (x+y=w1893:dbl)
                                n729 = local write "Potential Collisions"(w1893) -> ()
                                }
                                }
                                }
                                }
                                }
                                }
                                }
                                }
                                }
                                }
                                }
                              }
                            }
                          }
                        }
                        frame #1 {
                          n730 = local read "# of Spots"() -> (w1904:dbl)
                          n731 = Not Equal?(x=w1904, y=1) -> (x != y?=w1902:bool)
                          n732 = case shown="True" w1902 {
                            frame False {
                            }
                            frame True {
                              n733 = stacked-sequence {
                                frame #0 {
                                n734 = local read "Potential Collisions"() -> (w1907:dbl)
                                n735 = local read "Spot # Check"() -> (w1909:dbl)
                                n736 = Subtract(x=w1907, y=1) -> (x-y=w1905:dbl)
                                n737 = Less Or Equal?(x=w1909, y=w1905) -> (x <= y?=w1908:bool)
                                n738 = case shown="False" w1908 {
                                frame False {
                                n739 = local write "Spot # Check"(0) -> ()
                                }
                                frame True {
                                }
                                }
                                }
                                frame #1 {
                                n740 = local read "What to Check"() -> (w1915:dbl[])
                                n741 = local read "ID"() -> (w1913:dbl[])
                                n742 = local read "Spot # Check"() -> (w1911:dbl)
                                n743 = Index Array(array=w1915, index=w1911) -> (element=→"Value Check":dbl)
                                n744 = Index Array(array=w1913, index=w1911) -> (element=→"ID num check":dbl)
                                }
                              }
                            }
                          }
                        }
                      }
                    }
                  }
                  n745 = local read "Potential Collisions"() -> (w1692:dbl)
                  n746 = Subtract(x=w1692, y=1) -> (x-y=w1693:dbl)
                  n747 = local read "Hit"() -> (w1710:bool)
                  n748 = Equal?(x=w1705, y=w1693) -> (x = y?=w1709:bool)
                  n749 = Or(x=w1710, y=w1709) -> (x .or. y?=w1707:bool)
                }
                n750 = for {
                  tunnel: w1682 -> [w1929] mode=indexing
                  tunnel: w1683 -> [w1926] mode=indexing
                  tunnel: [w1928] -> w1677 mode=indexing
                  tunnel: w1679 -> [w1927]
                  # "If the projected distance is greater than the\nprevious distance, then the selected spots will move. \nThis situation only occurs if the bubble is about to/crossing \nthe buffer zone of another bubble. \n\nThe selected spots will also move if none of the bubbles\nare near/crossing the buffer zone of another bubble."
                  n751 = local read "Hit"() -> (w1919:bool)
                  n752 = Unbundle By Name(w1926) -> ()  [unwired: 1 out]
                  n753 = local read "Projected Distance"() -> (w1918:dbl)
                  n754 = Unbundle(w1929) -> ("Group ID"=→"Group ID #":i32, "Selected"=w1923:bool)
                  n755 = local read "Previous Distance"() -> (w1921:dbl)
                  n756 = Not(x=w1919) -> (.not. x?=w1917:bool)
                  n757 = Greater?(x=w1918, y=w1921) -> (0:w1920:bool)
                  n758 = And(x=w1919, y=w1920) -> (x .and. y?=w1916:bool)
                  n759 = Or(x=w1917, y=w1916) -> (x .or. y?=w1922:bool)
                  n760 = And(x=w1923, y=w1922) -> (x .and. y?=w1924:bool)
                  n761 = case shown="True" w1924 {
                    tunnel: w1926 -> [w1930 w1934]
                    tunnel: [w1930 w1933] -> w1928
                    tunnel: w1927 -> [_ w1935]
                    frame False {
                      # "otherwise, leave it alone!"
                    }
                    frame True {
                      # "If the spot is selected, move it by the same amount as the mouse"
                      n762 = call "extract_position.vi"("Spot"=w1934) -> ("Position"=w1932:cluster{"x":dbl, "y":dbl, "z":dbl})
                      n763 = Add(x=w1932, y=w1935) -> (x+y=w1931:cluster{dbl, dbl, dbl})
                      n764 = call "replace_position.vi"("Position"=w1931, "Spot in"=w1934) -> ("Spot"=w1933:T2)  [unwired: 2 out]
                    }
                  }
                }
                "Spot Checker" <- w1677
                n765 = local read "Locked Current Spot"() -> (w1673:dbl)
                n766 = Index Array(array=w1677, index=w1673) -> (element=w1676:T2)
                n767 = Unbundle By Name(w1676) -> ("Position.x"=→"New X":dbl, "Position.y"=→"New Y":dbl)  [unwired: 1 out]
                n768 = Array Size(array=w1677) -> (size(s)=→"# of Spots":i32)
              }
              frame True {
                # "coordinate conversion to find the rotation and scaling done by the mouse, about the centroid of the spots"
                n769 = Subtract(x=w1937, y=w1947) -> (x-y=w1956:cluster{dbl, dbl, dbl})
                n770 = Subtract(x=w1938, y=w1947) -> (x-y=w1955:cluster{dbl, dbl, dbl})
                n771 = Unbundle(w1955) -> (w1941:dbl, w1942:dbl)  [unwired: 1 out]
                n772 = Unbundle(w1956) -> (w1946:dbl, w1945:dbl)  [unwired: 1 out]
                n773 = Re/Im To Polar(2:w1942, 3:w1941) -> (0:w1939:dbl, 1:w1940:dbl)
                n774 = Re/Im To Polar(2:w1945, 3:w1946) -> (0:w1943:dbl, 1:w1944:dbl)
                n775 = Divide(x=w1940, y=w1944) -> (x/y=w1936:dbl)
                n776 = Subtract(x=w1939, y=w1943) -> (x-y=w1948:dbl)
                n777 = Bundle(w1936, w1936, w1936) -> (w1958:cluster{dbl, dbl, dbl})  [unwired: 1 out]
                n778 = call "scale_matrix.vi"("Scale Factors"=w1958) -> ("Scale Matrix"=w1954:T10)
                n779 = call "arb_rotation_matrix.vi"("Unit Vector"=cluster{dbl, dbl, dbl} {0.0, 0.0, 1.0}, "theta"=w1948) -> ("Real Matrix"=w1953:T10)
                n780 = call-poly <vilib>:"A x B.vi"("B"=w1953, "A"=w1954) -> ("A x B"=w1949:T10)  [unwired: 1 out]
                n781 = for {
                  tunnel: w1952 -> [w1964] mode=indexing
                  tunnel: [w1963] -> w1951 mode=indexing
                  tunnel: w1950 -> [w1962] mode=indexing
                  tunnel: w1947 -> [w1960]
                  tunnel: w1949 -> [w1959]
                  n782 = Unbundle(w1962) -> ("Selected"=w1961:bool)  [unwired: 1 out]
                  n783 = case shown="True" w1961 {
                    tunnel: w1964 -> [w1965 w1969]
                    tunnel: [w1965 w1968] -> w1963
                    tunnel: w1960 -> [_ w1967]
                    tunnel: w1959 -> [_ w1966]
                    frame False {
                    }
                    frame True {
                      n784 = call "apply_matrix_transformation_to_spots.vi"("Transform centre (i.e. transform about this point)"=w1967, "Transformation Matrix (3x3)"=w1966, "Spot In"=w1969) -> ("Spot Out"=w1968:T2)  [unwired: 5 out]
                    }
                  }
                }
              }
            }
          }
        }
        "Selection/Group" <- w1641
        n785 = Unbundle By Name(w1648) -> ("Position (Image Pixels)"=w1647:cluster{"X":dbl, "Y":dbl})
        n786 = Bundle By Name(cluster=w1648, "Dragging"=TRUE, "Previous Position (Image Pixels)"=w1647, "Position (Image Pixels)"=w1646) -> (w1657:T11)
      }
      event "stop": Value Change {
        n787 = event-data() -> ()  [unwired: 1 in, 4 out]
        n788 = global read "red_tweezers_globals_INTERNAL_VOLATILE.vi" "Current Settings File"() -> (w1973:path)
        n789 = call <vilib>:"Check if File or Folder Exists.vi"("path"=w1973) -> ("file or folder exists?"=w1972:bool)  [unwired: 8 in, 2 out]
        n790 = case shown="False" w1972 {
          tunnel: [w1980 w1984] -> w1974
          frame False {
            n791 = Two Button Dialog(message="Save current settings?", 1:"Don't Save" ("F button name (\"Cancel\")"), 2:"Save As..." ("T button name (\"OK\")")) -> (T button?=w1977:bool)
            n792 = Select(t=T16."Center Button" ("Which Button?"), s=w1977, f=T16."Right Button" ("Which Button?")) -> (s? t:f=w1980:T16)
          }
          frame True {
            n793 = call <vilib>:"Three Button Dialog.vi"("Allow user to close window? (TRUE)"=TRUE, "Window Title (\"\")"="Save Settings?" ("Window Title (\"\")"), "Right Button Text (\"Cancel\")"="No" ("Right Button Text (\"Cancel\")"), "Center Button Text (\"No\")"="Save As..." ("Center Button Text (\"No\")"), "Left Button Text (\"Yes\")"="Save" ("Left Button Text (\"Yes\")"), "message"="Would you like to save the current settings? You can choose to use the current settings file or save to a new location.") -> ("Which Button?"=w1984:T16)  [unwired: 5 in]
          }
        }
        n794 = case shown="\"Center Button\"" w1974 {
          tunnel: [TRUE TRUE FALSE FALSE] -> w1971
          frame "Left Button", Default {
          }
          frame "Center Button" {
            n795 = call "File Dialog5"("prompt"="Please select a location to save the settings", "button label"="Save", "default name"="red_tweezers_settings.xml", "pattern (all files)"="*.xml" ("pattern label"), "pattern label"="XML Settings Files") -> ("selected path"=w1992:path)  [unwired: 7 in, 3 out]
            n796 = global write "red_tweezers_globals_INTERNAL_VOLATILE.vi" "Current Settings File"(w1992) -> ()
          }
          frame "Right Button" {
          }
          frame "Window Close" {
          }
        }
        n797 = global write "red_tweezers_globals_INTERNAL_VOLATILE.vi" "Save Settings On Exit"(w1971) -> ()
      }
    }
    n798 = call "IMAQ Create"("Image Name"="untitled", "Image Type"=w62) -> ("New Image"=w61:T9)  [unwired: 3 in, 1 out]
    n799 = call "Vision Acquisition"() -> ("Image Out"=w60:T9)  [unwired: 24 in, 3 out]
    n800 = local read "Number of Matches Returned 2"() -> (w54:dbl)
    n801 = Add(x=w54, y=1.0 ("x+y")) -> (x+y=w58:dbl)
    n802 = call "IMAQ ExtractSingleColorPlane"("Color Plane"=w59, "Image Dst"=w61, "Image Src"=w60) -> ("Image Dst Out"=w33:T9)  [unwired: 7 in, 1 out]
    n803 = for {
      N: w58 -> [_]
      tunnel: w33 -> [w192]
      i -> [w220]
      # "ROI CODE TO SELECT SPECIFIC POINTS"
      n804 = local read "Circles 2"() -> (w207:T1)
      n805 = Number To Decimal String(number=w220) -> (decimal integer string=w219:string)  [unwired: 1 in]
      n806 = Index Array(array=w207) -> (element=w224:T25)  [unwired: 1 in]
      n807 = Unbundle(w224) -> ("Position"=w218:cluster{"X":sgl, "Y":sgl}, "Radius"=w206:dbl)  [unwired: 1 out]
      n808 = property on="Camera 3" class="ImageControl"() -> ("ROI"=w202:T26)  [unwired: 2 in, 2 out]
      n809 = Unbundle(w218) -> ("X"=w222:sgl, "Y"=w221:sgl)
      n810 = Unbundle By Name(w202) -> ("Contours"=w193:T27)
      n811 = Subtract(x=w222, y=w206) -> (x-y=→"toplx 2":dbl)
      n812 = Add(x=w222, y=w206) -> (x+y=→"bottomrx 2":dbl)
      n813 = Add(x=w221, y=w206) -> (x+y=→"bottomry 2":dbl)
      n814 = Subtract(x=w221, y=w206) -> (x-y=→"toply 2":dbl)
      n815 = Index Array(array=w193) -> (element=w194:T28)  [unwired: 1 in]
      n816 = Unbundle By Name(w194) -> ("Points"=w195:i32[])
      n817 = Index Array(array=w195, index #1=0 ("index"), index #2=1 ("index")) -> (element #1=w203:i32, element #2=w204:i32)
      "ROI-X" <- w203
      "ROI-Y" <- w204
      n818 = local read "toply 2"() -> (w210:dbl)
      n819 = local read "bottomrx 2"() -> (w209:dbl)
      n820 = Bundle(w203, w204) -> (w198:cluster{i32, i32})  [unwired: 1 in]
      "Specific Point" <- w198
      n821 = local read "toplx 2"() -> (w211:dbl)
      n822 = local read "bottomry 2"() -> (w208:dbl)
      n823 = Build Array(w211, w210, w209, w208) -> (w216:dbl[])
      n824 = call "IMAQ Overlay Text"("Text Color (black)"=u32 1703680, "Font, Size & Style"=T12 {"Desired Font (Application)"=enum."Application Font", "[User-specified Font]"={"Font Name"="", "Size"=40, "Strikeout?"=FALSE, "Italic?"=FALSE, "Underline?"=FALSE, "Outline?"=FALSE, "Shadow?"=FALSE, "Bold?"=FALSE, "Rotation Angle"=0.0}, "Horizontal Alignment"=0, "Vertical Alignment"=0}, "String"="ROI", "Origin"=w198, "Image"=w192) -> ()  [unwired: 5 in, 2 out]
      n825 = Array To Cluster(array=w216) -> (cluster=w223:T29)
      n826 = call "IMAQ Overlay Oval"("Bounding Rectangle"=w223, "Image"=w192) -> ("Image Out"=w217:T9)  [unwired: 8 in, 1 out]
      n827 = call "IMAQ Overlay Text"("String"=w219, "Origin"=w218, "Image"=w217) -> ("Image Out"=→"Camera 3":T9)  [unwired: 7 in, 1 out]
    }
    n828 = call-poly "IMAQ Detect Shapes"("Circle Descriptor"="Circle Descriptor 2", "Image"=w33) -> ("Number of Matches Returned"=→"Number of Matches Returned 2":i32, "Circles"=→"Circles 2":T1)  [unwired: 7 in, 1 out]
    n829 = case shown="True" "Camera Capture 2" {
      frame False {
      }
      frame True {
        n830 = local read "Circles 2"() -> (w180:T1)
        n831 = Index Array(array=w180) -> (element=w181:T25)  [unwired: 1 in]
        n832 = Index Array(array=w180) -> (element=w191:T25)  [unwired: 1 in]
        n833 = Unbundle(w181) -> ("Position"=w189:cluster{"X":sgl, "Y":sgl}, "Radius"=w182:dbl)  [unwired: 1 out]
        n834 = Unbundle(w191) -> ("Position"=w190:cluster{"X":sgl, "Y":sgl})  [unwired: 2 out]
        n835 = Unbundle(w189) -> ("X"=w187:sgl, "Y"=w188:sgl)
        n836 = Unbundle(w190) -> ("X"=→"Object x":sgl, "Y"=→"Object y":sgl)
        n837 = Subtract(x=w187, y=w182) -> (x-y=→"toplx 3":dbl)
        n838 = Add(x=w187, y=w182) -> (x+y=→"bottomrx 3":dbl)
        n839 = Add(x=w188, y=w182) -> (x+y=→"bottomry 3":dbl)
        n840 = Subtract(x=w188, y=w182) -> (x-y=→"toply 3":dbl)
      }
    }
    n841 = case shown="1" "Numeric 2" {
      frame 0, Default {
        n842 = local read "ROI-X"() -> (w172:dbl)
        n843 = local read "ROI-Y"() -> (w171:dbl)
        n844 = Build Array(w172, w171) -> (w169:T10)
        n845 = call-poly <vilib>:"Multiply.vi"("Real Scalar c"=1e-07 ("y"), "Real Matrix A"=w169) -> ("A * c"=→"ROI 0":T10)
      }
      frame 1 {
        n846 = local read "ROI-X"() -> (w177:dbl)
        n847 = local read "ROI-Y"() -> (w176:dbl)
        n848 = Build Array(w177, w176) -> (w174:T10)
        n849 = call-poly <vilib>:"Multiply.vi"("Real Matrix A"=w174, "Real Scalar c"=1e-07 ("y")) -> ("c * A"=→"ROI 1":T10)
      }
    }
    n850 = local read "Stop"() -> (w65:i32)
    n851 = local read "Start"() -> (w64:i32)
    n852 = Subtract(x=w65, y=w64) -> (x-y=→"Time Elapsed(ms)":i32)
    n853 = case shown="True" "Play" {
      frame False {
      }
      frame True {
        n854 = stacked-sequence {
          frame #0 {
            n855 = Tick Count (ms)() -> (millisecond timer value=→"Start":u32)
          }
          frame #1 {
            n856 = case shown="False" "Input Object Location" {
              frame False {
                # "If Play is pressed, but user input is not, will surround object \n(a circle right now)"
                n857 = local read "Object X"() -> (w400:dbl)
                n858 = local read "bottomry 2"() -> (w402:dbl)
                n859 = local read "toply 2"() -> (w397:dbl)
                n860 = local read "toplx 2"() -> (w410:dbl)
                n861 = local read "Object Y"() -> (w409:dbl)
                n862 = local read "Object X"() -> (w393:dbl)
                n863 = local read "bottomrx 2"() -> (w415:dbl)
                n864 = local read "Object Y"() -> (w414:dbl)
                n865 = Multiply(x=w410, y=1e-07) -> (x*y=w411:dbl)
                n866 = Multiply(x=w400, y=1e-07) -> (x*y=w403:dbl)
                n867 = Multiply(x=w409, y=1e-07) -> (x*y=w412:dbl)
                n868 = Multiply(x=w414, y=1e-07) -> (x*y=w413:dbl)
                n869 = Multiply(x=w402, y=1e-07) -> (x*y=w404:dbl)
                n870 = Multiply(x=w397, y=1e-07) -> (x*y=w398:dbl)
                n871 = Multiply(x=w415, y=1e-07) -> (x*y=w416:dbl)
                n872 = Multiply(x=w393, y=1e-07) -> (x*y=w395:dbl)
                n873 = Build Array(w395, w398) -> (w389:T10)
                n874 = Build Array(w403, w404) -> (w390:T10)
                n875 = Build Array(w416, w413) -> (w391:T10)
                n876 = Build Array(w411, w412) -> (w392:T10)
                n877 = Build Array (concatenate)(w389, w390, w391, w392) -> (w388:T10)
                n878 = local write "NewXYArray"(w388) -> ()
              }
              frame True {
                n879 = local read "distance  bw x and rad"() -> (w418:dbl)
                n880 = local read "distance  bw x and rad"() -> (w421:dbl)
                n881 = local read "Object New Y"() -> (w428:dbl)
                n882 = local read "Object New Y"() -> (w425:dbl)
                n883 = local read "Object New X"() -> (w422:dbl)
                n884 = local read "distance bw y and rad"() -> (w427:dbl)
                n885 = local read "Object New X"() -> (w419:dbl)
                n886 = local read "distance bw y and rad"() -> (w424:dbl)
                n887 = local read "Object New X"() -> (w443:dbl)
                n888 = local read "Object New X"() -> (w453:dbl)
                n889 = Subtract(x=w419, y=w418) -> (x-y=w417:dbl)
                n890 = local read "Object New Y"() -> (w431:dbl)
                n891 = Add(x=w422, y=w421) -> (x+y=w420:dbl)
                n892 = Subtract(x=w428, y=w427) -> (x-y=w426:dbl)
                n893 = Add(x=w425, y=w424) -> (x+y=w423:dbl)
                n894 = local read "Object New Y"() -> (w436:dbl)
                n895 = Multiply(x=w417, y=1e-07) -> (x*y=w433:dbl)
                n896 = Multiply(x=w426, y=1e-07) -> (x*y=w449:dbl)
                n897 = Multiply(x=w453, y=1e-07) -> (x*y=w450:dbl)
                n898 = Multiply(x=w423, y=1e-07) -> (x*y=w440:dbl)
                n899 = Multiply(x=w443, y=1e-07) -> (x*y=w444:dbl)
                n900 = Multiply(x=w420, y=1e-07) -> (x*y=w439:dbl)
                n901 = Multiply(x=w436, y=1e-07) -> (x*y=w435:dbl)
                n902 = Multiply(x=w431, y=1e-07) -> (x*y=w430:dbl)
                n903 = Build Array(w450, w449) -> (w448:T10)
                n904 = Build Array(w444, w440) -> (w447:T10)
                n905 = Build Array(w439, w435) -> (w446:T10)
                n906 = Build Array(w433, w430) -> (w445:T10)
                n907 = Build Array (concatenate)(w448, w447, w446, w445) -> (w429:T10)
                n908 = local write "NewXYArray"(w429) -> ()
              }
            }
            n909 = local write "Max Number of Bubbles 2"("Max Number of Bubbles 2") -> ()
            n910 = local write "LCS"("LCS") -> ()
            n911 = local write "Rates"("Rates") -> ()
            n912 = local write "How Many Frames?"("Number of Planned Sequence Frames 2") -> ()
            "Initiate Creation 2" <- 1.0
          }
          frame #2 {
            n913 = local read "NewXYArray"() -> (w457:dbl[][])
            n914 = Array Size(array=w457) -> (size(s)=w456:i32[])
            n915 = Index Array(array=w456, index=0) -> (element=w454:i32)
            "NewXYArraySize" <- w454
            n916 = for {
              N: w454 -> [w459]
              i -> [w460]
              stop <- w458 stop-if-true
              n917 = stacked-sequence {
                tunnel: w460 -> [w462 _]
                tunnel: w459 -> [w461 _]
                tunnel: [_ w465] -> w458
                frame #0 {
                  n918 = local write "Locked Current Spot"(w462) -> ()
                  n919 = local write "# of Spots"(w461) -> ()
                  n920 = local write "Rates"(1) -> ()
                  n921 = local write "LCS"(0) -> ()
                }
                frame #1 {
                  n922 = local read "Insert"() -> (w465:bool)
                  n923 = local write "Insert"(TRUE) -> ()
                }
              }
            }
          }
        }
      }
    }
    n924 = local read "toplx 2"() -> (w45:dbl)
    n925 = local read "bottomrx 2"() -> (w46:dbl)
    n926 = Subtract(x=w45, y=w46) -> (x-y=w48:dbl)
    n927 = local read "toplx 2"() -> (w50:dbl)
    n928 = Absolute Value(x=w48) -> (abs(x)=w49:dbl)
    n929 = Divide(x=w49, y=2.0) -> (x/y=w37:dbl)
    "distance  bw x and rad" <- w37
    n930 = Add(x=w37, y=w50) -> (x+y=→"Object X":dbl)
    n931 = local write "Object New X"("Object New X") -> ()
    n932 = local write "Object New Y"("Object New Y") -> ()
    n933 = local read "bottomry 2"() -> (w44:dbl)
    n934 = local read "toply 2"() -> (w43:dbl)
    n935 = Subtract(x=w44, y=w43) -> (x-y=w42:dbl)
    n936 = local read "toply 2"() -> (w39:dbl)
    n937 = Absolute Value(x=w42) -> (abs(x)=w41:dbl)
    n938 = Divide(x=w41, y=2.0) -> (x/y=w36:dbl)
    "distance bw y and rad" <- w36
    n939 = Add(x=w36, y=w39) -> (x+y=→"Object Y":dbl)
    n940 = case shown="True" "Lock Current Spot" {
      frame False {
      }
      frame True {
        n941 = global read "red_tweezers_globals.vi" "Spots"() -> (w544:T2[])
        n942 = local read "Current Spot #"() -> (w545:dbl)
        "Locked Current Spot" <- w545
        n943 = Index Array(array=w544, index=w545) -> (element=w546:T2)
        n944 = Unbundle By Name(w546) -> ("Position.x"=→"LCS X":dbl, "Position.y"=→"LCS Y":dbl)
        n945 = local write "LCS"(0) -> ()
      }
    }
    n946 = local read "Rates"() -> (w70:dbl)
    n947 = Equal?(x=w70, y=1.0) -> (x = y?=w68:bool)
    n948 = case shown="True" w68 {
      frame False {
      }
      frame True {
        n949 = stacked-sequence {
          frame #0 {
            n950 = local read "Number of Planned Sequence Frames 2"() -> (w310:dbl)
            n951 = local read "Tab Control"() -> (w311:enum32{"Line", "Arc"})
            n952 = case shown="\"Arc\"" w311 {
              tunnel: w310 -> [w313 w351]
              frame "Arc" {
                w324 = 1e-07 ("x")
                w346 = 2
                n953 = Subtract(x=w313, y=1.0) -> (x-y=w312:dbl)
                n954 = expression code="(x/180.0)*pi" "degrees to radians"(180.0) -> (w341:dbl)
                n955 = local read "Current Y"() -> (w335:dbl)
                n956 = local read "Current X"() -> (w337:dbl)
                n957 = local read "Center Y"() -> (w336:dbl)
                n958 = local read "Center X"() -> (w338:dbl)
                n959 = Subtract(x=w336, y=w335) -> (x-y=w318:dbl)
                "Original\nD-Y" <- w318
                n960 = Subtract(x=w338, y=w337) -> (x-y=w319:dbl)
                "Original\nD-X" <- w319
                n961 = Divide(x=w341, y=w312) -> (x/y=→"Degree Rate":dbl)
                n962 = Divide(x=w318, y=w319) -> (x/y=w334:dbl)
                n963 = Inverse Tangent(1:w334) -> (0:w317:dbl)
                n964 = Add(x=w317, y=3.141592653589793) -> (x+y=→"Original \nTheta":dbl)
                n965 = local read "ROI-Y"() -> (w322:dbl)
                n966 = local read "ROI-X"() -> (w323:dbl)
                n967 = local read "Current Y"() -> (w348:dbl)
                n968 = local read "Current X"() -> (w344:dbl)
                n969 = Multiply(x=w324, y=w322) -> (x*y=w321:dbl)
                n970 = Multiply(x=w324, y=w323) -> (x*y=w320:dbl)
                n971 = local read "Original\nD-X"() -> (w333:dbl)
                n972 = local read "Original\nD-Y"() -> (w332:dbl)
                n973 = Add(x=w321, y=w348) -> (x+y=w347:dbl)
                n974 = Add(x=w320, y=w344) -> (x+y=w345:dbl)
                n975 = Divide(x=w347, y=w346) -> (x/y=w339:dbl)
                "Center Y" <- w339
                n976 = Divide(x=w345, y=w346) -> (x/y=w340:dbl)
                "Center X" <- w340
                n977 = Build Array(w340, w339) -> (→"Center location":T10)
                n978 = Square(x=w333) -> (x^2=w331:dbl)
                n979 = Square(x=w332) -> (x^2=w330:dbl)
                n980 = Add(x=w331, y=w330) -> (x+y=w329:dbl)
                n981 = Square Root(x=w329) -> (sqrt(x)=→"Original\nRadius":dbl)
                n982 = local read "Position"() -> (w327:cluster{"x":dbl, "y":dbl, "z":dbl})
                n983 = Unbundle(w327) -> ("x"=→"Current X":dbl, "y"=→"Current Y":dbl)  [unwired: 1 out]
              }
              frame "Line" {
                n984 = local read "Max Number of Bubbles 2"() -> (w350:dbl)
                n985 = for {
                  N: w350 -> [_]
                  tunnel: w351 -> [w353]
                  i -> [w352]
                  n986 = stacked-sequence {
                    tunnel: w353 -> [_ w371]
                    tunnel: w352 -> [w357 w368]
                    frame #0 {
                      n987 = local read "NewXYArray"() -> (w363:dbl[][])
                      n988 = Index Array(array=w363, index (row)=w357) -> (element=w362:dbl[])  [unwired: 1 in]
                      n989 = Array To Cluster(array=w362) -> (cluster=w361:T30)
                      n990 = global read "red_tweezers_globals.vi" "Spots"() -> (w358:T2[])
                      n991 = Unbundle By Name(w361) -> ("NewXYArray[0]"=w360:dbl, "NewXYArray[1]"=w359:dbl)
                      n992 = Index Array(array=w358, index=w357) -> (element=w356:T2)
                      n993 = local write "New Y"(w359) -> ()
                      n994 = local write "New X"(w360) -> ()
                      n995 = Unbundle By Name(w356) -> ("Position.x"=w355:dbl, "Position.y"=w354:dbl)
                      n996 = local write "Original X"(w355) -> ()
                      n997 = local write "Original Y"(w354) -> ()
                    }
                    frame #1 {
                      n998 = local read "Original X"() -> (w372:dbl)
                      n999 = local read "Original Y"() -> (w374:dbl)
                      n1000 = Subtract(x=w371, y=1) -> (x-y=w378:dbl)
                      n1001 = local read "New Y"() -> (w375:dbl)
                      n1002 = local read "New X"() -> (w373:dbl)
                      n1003 = Subtract(x=w374, y=w375) -> (x-y=w377:dbl)
                      n1004 = Subtract(x=w372, y=w373) -> (x-y=w376:dbl)
                      n1005 = Divide(x=w377, y=w378) -> (x/y=w366:dbl)
                      "Y Rate" <- w366
                      n1006 = Divide(x=w376, y=w378) -> (x/y=w367:dbl)
                      "X Rate" <- w367
                      n1007 = Bundle(w367, w366) -> (w365:cluster{dbl, dbl})  [unwired: 1 in]
                      n1008 = local read "NewXYRates"() -> (w369:dbl[][])
                      n1009 = Cluster To Array(cluster=w365) -> (array=w364:dbl[])
                      n1010 = Insert Into Array(array=w369, index (row)=w368, new element=w364) -> (w370:dbl[][])  [unwired: 1 in]
                      n1011 = local write "NewXYRates"(w370) -> ()
                    }
                  }
                }
              }
            }
          }
          frame #1 {
            n1012 = local write "Rates"(0) -> ()
          }
        }
      }
    }
    n1013 = case shown="True" "Mark Original Position" {
      frame False {
      }
      frame True {
        w547 = TRUE
        n1014 = local write "Mark Original Position"(FALSE) -> ()
        n1015 = local read "New X"() -> (→"Original X":dbl)
        n1016 = local read "New Y"() -> (→"Original Y":dbl)
        "MOP pressed After" <- w547
        "MOP pressed" <- w547
      }
    }
    n1017 = local read "Sequence Instances"() -> (w126:dbl)
    n1018 = case shown="True" w145 {
      tunnel: w151 -> [_ w613]
      frame False {
      }
      frame True {
        n1019 = global write "red_tweezers_globals_INTERNAL.vi" "Image Overlay (extras from control loop)"(w613) -> ()
      }
    }
    n1020 = local read "Counter"() -> (w125:dbl)
    n1021 = call "red_tweezers_UNDO.vi"("Force Save"=w147, "This change is inconsequential (don't save it)"=w148, "Selection/Group"=w149, "Spots"=w150) -> ()  [unwired: 6 in, 2 out]
    n1022 = call "sync_with_globals.vi"("Selection/Group"=w149, "Spots"=w150) -> ("Selection/Group 2"=w161:T8[], "Spots 2"=w112:T2[])  [unwired: 4 in]
    n1023 = local read "Sequence Storer"() -> (w121:T2[][])
    n1024 = local read "Sequence On?"() -> (w124:bool)
    n1025 = local read "Sequence On?"() -> (w139:bool)
    n1026 = call "SequenceControl.vi"("Sequence On? 2"=w124, "Counter 2"=w125, "Sequence Instances 2"=w126, "Sequence Storer"=w121) -> ("Time per Frame (ms) 2"=w119:dbl, "Sequence Order 2"=w122:dbl, "Reset 2"=w123:bool, "Sequence Storer 2"=w134:T2[][], "Clearance Button 2"=w133:bool, "Manual Edit 2"=w132:bool, "Save State 2"=w131:bool, "Play Sequence 2"=w128:bool, "Bubble ID to Empty 2"=w127:dbl, "Manual Sequence 2"=w129:bool, "Edit Sequence Mode 2"=w130:bool)  [unwired: 1 in]
    n1027 = local write "Play Sequence"(w128) -> ()
    n1028 = local write "Bubble ID to Empty"(w127) -> ()
    n1029 = local write "Manual Sequence"(w129) -> ()
    n1030 = local write "Reset"(w123) -> ()
    n1031 = local write "Edit Sequence Mode"(w130) -> ()
    n1032 = local write "Clearance Button"(w133) -> ()
    n1033 = local write "Sequence Storer"(w134) -> ()
    n1034 = local write "Save State"(w131) -> ()
    n1035 = local write "Manual Edit"(w132) -> ()
    n1036 = Or(x=w139, y="Manual Sequence") -> (x .or. y?=w138:bool)
    n1037 = local write "Time per Frame (ms)"(w119) -> ()
    n1038 = feedback #10() -> (w166:T31)  [unwired: 1 out]
    n1039 = call "Smoothed Frame Rate.vi"("Feedback In"=w166) -> ("Feedback Out"=w165:T31, "Frame Rate"=→"Interface Frame Rate":dbl)  [unwired: 1 in, 4 out]
    n1040 = feedback-in #10(w165) -> ()
    n1041 = local write "Sequence Order"(w122) -> ()
    n1042 = Not(x=w115) -> (.not. x?=w116:bool)
    n1043 = Not(x="Output to SLM") -> (.not. x?=w117:bool)
    n1044 = case shown="True" w138 {
      tunnel: [w583 w588] -> w142
      tunnel: w112 -> [w582 _]
      frame False {
        n1045 = Or(x="Manual Edit", y="Edit Sequence Mode") -> (x .or. y?=w581:bool)
        n1046 = case shown="False" w581 {
          tunnel: w582 -> [w584 _]
          tunnel: [w584 w585] -> w583
          frame False {
          }
          frame True {
            n1047 = local read "Sequence Order"() -> (w586:dbl)
            n1048 = local read "Sequence Storer"() -> (w587:T2[][])
            n1049 = Index Array(array=w587, index (row)=w586) -> (element=w585:T2[])  [unwired: 1 in]
          }
        }
      }
      frame True {
        n1050 = stacked-sequence {
          tunnel: [w590 _] -> w588
          frame #0 {
            n1051 = local read "Counter"() -> (w591:dbl)
            n1052 = local read "Sequence Storer"() -> (w592:T2[][])
            n1053 = Index Array(array=w592, index (row)=w591) -> (element=w590:T2[])  [unwired: 1 in]
            n1054 = Wait (ms)(milliseconds to wait="Time per Frame (ms)") -> ()  [unwired: 1 out]
          }
          frame #1 {
            n1055 = local read "Sequence Instances"() -> (w594:dbl)
            n1056 = local read "Counter"() -> (w597:dbl)
            n1057 = Subtract(x=w594, y=1) -> (x-y=w595:dbl)
            n1058 = Equal?(x=w597, y=w595) -> (x = y?=w596:bool)
            n1059 = case shown="True" w596 {
              frame False {
                n1060 = local read "Counter"() -> (w600:dbl)
                n1061 = Add(x=w600, y=1) -> (x+y=→"Counter":dbl)
              }
              frame True {
                w601 = FALSE
                n1062 = local write "Counter"(0) -> ()
                n1063 = local write "Play Sequence"(w601) -> ()
                n1064 = local write "Sequence On?"(w601) -> ()
              }
            }
          }
        }
      }
    }
    n1065 = case shown="True" "Save State" {
      tunnel: w112 -> [_ w604]
      frame False {
      }
      frame True {
        n1066 = local write "Save State"(FALSE) -> ()
        n1067 = stacked-sequence {
          tunnel: w604 -> [w605 _]
          frame #0 {
            "Spot Storage" <- w605
          }
          frame #1 {
            n1068 = local read "Spot Storage"() -> (w611:T2[])
            n1069 = Replace Array Subset(array="Sequence Storer", new element=w611, index (row)="Sequence Order") -> (w609:T2[][])  [unwired: 1 in]
            n1070 = Array Size(array=w609) -> (size(s)=w608:i32[])
            n1071 = local write "Sequence Storer"(w609) -> ()
            n1072 = Index Array(array=w608, index=0) -> (element=→"Sequence Instances":i32)
          }
        }
      }
    }
    n1073 = case shown="True" "Clearance Button" {
      frame False {
      }
      frame True {
        # "This is the Bubble ID to Empty tool- this \"deletes\" the bubble in a sequence."
        n1074 = local read "Sequence Order"() -> (w574:dbl)
        n1075 = local read "Sequence Storer"() -> (w575:T2[][])
        n1076 = Replace Array Subset(array=w575, new element=T13 {"Position"={"x"=nan, "y"=nan, "z"=nan}, "Intensity"=1.0, "Vortex Charge"=1, "Phase"=1.0, "NA Position"={"x"=0.0, "y"=0.0, "r"=1.0}, "Line Trapping"={"Vector"={"x"=0.0, "y"=0.0, "z"=0.0}, "Phase Gradient"=0.0}, "Amplitude Correction"=0.0} ("Cluster"), index (row)=w574, index (col)="Bubble ID to Empty") -> (w571:T2[][])
        n1077 = local write "Sequence Storer"(w571) -> ()
      }
    }
    n1078 = case shown="True" "Save" {
      frame False {
      }
      frame True {
        n1079 = local read "Sequence Storer"() -> (w540:T2[][])
        n1080 = call "SequenceSaver.vi"("Sequence Storer"=w540) -> ()  [unwired: 10 in, 1 out]
      }
    }
    n1081 = And(x=w117, y=w116) -> (x .and. y?=w120:bool)
    n1082 = case shown="True" "Load" {
      frame False {
      }
      frame True {
        n1083 = call "SequenceSaver.vi"() -> ("Sequence Storer 2"=w539:T2[][])  [unwired: 11 in]
        n1084 = local write "Sequence Storer"(w539) -> ()
      }
    }
    n1085 = local read "Initiate Creation 2"() -> (w73:dbl)
    n1086 = case shown="True" w120 {
      tunnel: w112 -> [w2001 _]
      frame False {
        n1087 = call "UDP Sender generic_2.vi"("Spots"=w2001) -> ()  [unwired: 2 in, 1 out]
      }
      frame True {
      }
    }
    n1088 = case shown="True" "Reset" {
      frame False {
      }
      frame True {
        n1089 = local write "Counter"(0) -> ()
      }
    }
    n1090 = case shown="True" "Add Additional Frames" {
      frame False {
      }
      frame True {
        # "This adds additional frames to the sequence."
        n1091 = for {
          N: "Additional Frames Wanted" -> [_]
          i -> [w553]
          n1092 = local read "Max Number of Bubbles 2"() -> (w557:dbl)
          n1093 = Add(x=1, y=w553) -> (x+y=w554:i32)
          n1094 = Add(x="Frame Location", y=w554) -> (x+y=w555:dbl)
          n1095 = Initialize Array(T13 {"Position"={"x"=nan, "y"=nan, "z"=nan}, "Intensity"=1.0, "Vortex Charge"=1, "Phase"=1.0, "NA Position"={"x"=0.0, "y"=0.0, "r"=1.0}, "Line Trapping"={"Vector"={"x"=0.0, "y"=0.0, "z"=0.0}, "Phase Gradient"=0.0}, "Amplitude Correction"=0.0} ("Cluster"), w557) -> (w558:T32)
          n1096 = local read "Sequence Storer"() -> (w559:T2[][])
          n1097 = Insert Into Array(array=w559, index (row)=w555, new element=w558) -> (w560:T2[][])  [unwired: 1 in]
          n1098 = local write "Sequence Storer"(w560) -> ()
        }
      }
    }
    n1099 = case shown="1" w73 {
      frame 0, Default {
      }
      frame 1 {
        # "This create the array needed for a sequential\narray."
        n1100 = local read "Number of Planned Sequence Frames 2"() -> (w564:dbl)
        n1101 = local read "Max Number of Bubbles 2"() -> (w563:dbl)
        n1102 = for {
          N: w564 -> [_]
          tunnel: w563 -> [w565]
          i -> [w568]
          n1103 = Initialize Array(T13 {"Position"={"x"=nan, "y"=nan, "z"=nan}, "Intensity"=1.0, "Vortex Charge"=1, "Phase"=1.0, "NA Position"={"x"=0.0, "y"=0.0, "r"=1.0}, "Line Trapping"={"Vector"={"x"=0.0, "y"=0.0, "z"=0.0}, "Phase Gradient"=0.0}, "Amplitude Correction"=0.0} ("Cluster"), w565) -> (w566:T32)
          n1104 = local read "Sequence Storer"() -> (w569:T2[][])
          n1105 = Insert Into Array(array=w569, index (row)=w568, new element=w566) -> (w570:T2[][])  [unwired: 1 in]
          n1106 = local write "Sequence Storer"(w570) -> ()
        }
        n1107 = local write "Initiate Creation 2"(0) -> ()
      }
    }
    n1108 = case shown="False" "Play Sequence" {
      frame False {
        n1109 = local write "Sequence On?"(FALSE) -> ()
      }
      frame True {
        "Sequence On?" <- TRUE
      }
    }
    n1110 = local read "Current Spot #"() -> (w95:dbl)
    n1111 = local read "Selection/Group"() -> (w96:T8[])
    n1112 = local read "# of Spots"() -> (w111:dbl)
    n1113 = Not Equal?(x=w95, y=-1) -> (x != y?=w97:bool)
    n1114 = local read "spots selected 2"() -> (w85:i32)
    n1115 = Index Array(array=w96, index=w95) -> (element=w94:T8)
    n1116 = Unbundle By Name(w94) -> ("Selected"=w93:bool)
    n1117 = local read "spots selected"() -> (w86:i32)
    n1118 = Not(x=w93) -> (.not. x?=w92:bool)
    n1119 = And(x=w92, y=w97) -> (x .and. y?=w87:bool)
    n1120 = Less?(x=w86, y=w85) -> (x < y?=w83:bool)
    n1121 = case shown="True" "Insert" {
      tunnel: w112 -> [_ w226]
      tunnel: w111 -> [_ w225]
      frame False {
      }
      frame True {
        n1122 = for {
          N: w225 -> [_]
          tunnel: w226 -> [w228]
          i -> [w227]
          n1123 = stacked-sequence {
            tunnel: w228 -> [w230 w235 _]
            tunnel: w227 -> [_ w231 _]
            frame #0 {
              n1124 = local read "Start at Which Frame?"() -> (→"Num":dbl)
              "Spot Storage 2" <- w230
            }
            frame #1 {
              n1125 = local read "Selection/Group"() -> (w234:T8[])
              n1126 = Index Array(array=w234, index=w231) -> (element=w233:T8)
              n1127 = Unbundle By Name(w233) -> ("Selected"=w232:bool)
              n1128 = case shown="True" w232 {
                tunnel: w235 -> [_ _]
                frame False {
                }
                frame True {
                  n1129 = stacked-sequence {
                    frame #0 {
                      n1130 = case shown="\"Arc\"" "Tab Control" {
                        frame "Arc" {
                          n1131 = local read "How Many Frames?"() -> (w239:dbl)
                          n1132 = Subtract(x=w239, y=1) -> (x-y=w237:dbl)
                          n1133 = for {
                            N: w239 -> [_]
                            tunnel: w237 -> [w241]
                            i -> [w243]
                            # "What is this ^\n\nFor # of sequence\nframes, don't worry\nabout it"
                            # "How to make position x and y?\nIt's called a cluster, inser the new position to Position.x and Position.y"
                            n1134 = Equal?(x=w241, y=w243) -> (x = y?=w242:bool)
                            n1135 = case shown="False" w242 {
                              tunnel: [w265 w278] -> w245
                              tunnel: [w264 w277] -> w244
                              tunnel: w243 -> [w262 _]
                              frame False {
                                # "calculating new position"
                                n1136 = local read "Original \nTheta"() -> (w274:dbl)
                                n1137 = local read "Degree Rate"() -> (w276:dbl)
                                n1138 = Add(x=w262, y=1.0) -> (x+y=w261:dbl)
                                n1139 = Multiply(x=w276, y=w261) -> (x*y=w275:dbl)
                                n1140 = Add(x=w274, y=w275) -> (x+y=w273:dbl)
                                n1141 = local read "Original\nRadius"() -> (w270:dbl)
                                n1142 = Cosine(x=w273) -> (cos(x)=w272:dbl)
                                n1143 = Sine(x=w273) -> (sin(x)=w271:dbl)
                                n1144 = Multiply(x=w271, y=w270) -> (x*y=w267:dbl)
                                n1145 = Multiply(x=w272, y=w270) -> (x*y=w269:dbl)
                                n1146 = local read "Center X"() -> (w268:dbl)
                                n1147 = local read "Center Y"() -> (w266:dbl)
                                n1148 = Subtract(x=w268, y=w269) -> (x-y=w265:dbl)
                                n1149 = Add(x=w266, y=w267) -> (x+y=w264:dbl)
                              }
                              frame True {
                                n1150 = global read "red_tweezers_globals.vi" "Spots"() -> (w281:T2[])
                                n1151 = local read "Numeric"() -> (w280:dbl)
                                n1152 = Index Array(array=w281, index=w280) -> (element=w279:T2)
                                n1153 = Unbundle By Name(w279) -> ("Position.x"=w278:dbl, "Position.y"=w277:dbl)
                              }
                            }
                            n1154 = local read "Spot Storage 2"() -> (w260:T2[])
                            n1155 = local read "Numeric"() -> (w259:dbl)
                            n1156 = Index Array(array=w260, index=w259) -> (element=w247:T2)
                            n1157 = local read "Start at Which Frame?"() -> (w240:dbl)
                            "Numeric 4" <- w240
                            n1158 = Bundle By Name(cluster=w247, "Position.x"=w245, "Position.y"=w244) -> (w246:T2)
                            n1159 = local read "How Many Frames?"() -> (w248:dbl)
                            n1160 = Subtract(x=w240, y=w243) -> (x-y=w257:dbl)
                            n1161 = local read "Sequence Storer"() -> (w258:T2[][])
                            n1162 = local read "Numeric"() -> (w253:dbl)
                            n1163 = Add(x=w257, y=w248) -> (x+y=w256:dbl)
                            n1164 = Subtract(x=w256, y=1) -> (x-y=w254:dbl)
                            n1165 = Replace Array Subset(array=w258, new element=w246, index (row)=w254, index (col)=w253) -> (w252:T2[][])
                            n1166 = Array Size(array=w252) -> (size(s)=w251:i32[])
                            n1167 = local write "Sequence Storer"(w252) -> ()
                            n1168 = Index Array(array=w251, index=0) -> (element=w249:i32)
                            n1169 = local write "Sequence Instances"(w249) -> ()
                          }
                        }
                        frame "Line" {
                          # "This is the automatic sequence generator which allows for the creation of the sequence. This calculates the LAST coordinates of each bubble first\nbefore going for the first few coordinates of the sequence."
                          n1170 = local read "How Many Frames?"() -> (w282:dbl)
                          n1171 = for {
                            N: w282 -> [_]
                            i -> [w290]
                            # "For why do we multiply?"
                            n1172 = local read "Spot Storage 2"() -> (w300:T2[])
                            n1173 = local read "Numeric"() -> (w287:dbl)
                            n1174 = local read "NewXYRates"() -> (w288:dbl[][])
                            n1175 = Index Array(array=w288, index (row)=w287, index (col)=1) -> (element=w283:dbl)
                            n1176 = Index Array(array=w288, index (row)=w287, index (col)=0) -> (element=w284:dbl)
                            n1177 = Index Array(array=w300, index=w287) -> (element=w298:T2)
                            n1178 = Unbundle By Name(w298) -> ("Position.x"=w305:dbl, "Position.y"=w303:dbl)
                            n1179 = Multiply(x=w284, y=w290) -> (x*y=w304:dbl)
                            n1180 = Multiply(x=w283, y=w290) -> (x*y=w299:dbl)
                            "probe" <- w299
                            n1181 = Subtract(x=w305, y=w304) -> (x-y=w302:dbl)
                            n1182 = Subtract(x=w303, y=w299) -> (x-y=w301:dbl)
                            n1183 = Bundle By Name(cluster=w298, "Position.x"=w302, "Position.y"=w301) -> (w293:T2)
                            n1184 = local read "Sequence Storer"() -> (w306:T2[][])
                            n1185 = local read "Numeric"() -> (w292:dbl)
                            n1186 = Add(x="Start at Which Frame?", y=w290) -> (x+y=w289:dbl)
                            n1187 = Replace Array Subset(array=w306, new element=w293, index (row)=w289, index (col)=w292) -> (w297:T2[][])
                            n1188 = Array Size(array=w297) -> (size(s)=w296:i32[])
                            n1189 = local write "Sequence Storer"(w297) -> ()
                            n1190 = Index Array(array=w296, index=0) -> (element=w294:i32)
                            n1191 = local write "Sequence Instances"(w294) -> ()
                          }
                        }
                      }
                    }
                    frame #1 {
                      w308 = FALSE
                      n1192 = Tick Count (ms)() -> (millisecond timer value=→"Stop":u32)
                      n1193 = local write "Play Pressed"(w308) -> ()
                      "Insert End" <- w308
                    }
                  }
                }
              }
              "Numeric" <- w231
            }
            frame #2 {
              n1194 = local write "Insert"(FALSE) -> ()
            }
          }
        }
      }
    }
    n1195 = And(x=w83, y=w87) -> (x .and. y?=w88:bool)
    n1196 = case shown="True" w88 {
      frame False {
      }
      frame True {
        n1197 = local read "# of Spots"() -> (w474:dbl)
        n1198 = for {
          N: w474 -> [_]
          i -> [w476]
          stop <- w475 stop-if-true
          n1199 = local read "Selection/Group"() -> (w478:T8[])
          n1200 = Index Array(array=w478, index=w476) -> (element=w477:T8)
          n1201 = Unbundle By Name(w477) -> ("Selected"=w475:bool)
          n1202 = case shown="True" w475 {
            tunnel: w476 -> [_ w480]
            frame False {
            }
            frame True {
              n1203 = local write "Current Spot #"(w480) -> ()
              "Induce check" <- TRUE
            }
          }
        }
      }
    }
    n1204 = local read "spots selected"() -> (w98:i32)
    n1205 = local read "spots selected 2"() -> (w99:i32)
    n1206 = local read "Prev Current Spot"() -> (w107:dbl)
    n1207 = local read "Current Spot #"() -> (w108:dbl)
    n1208 = Not Equal?(x=w108, y=w107) -> (x != y?=w106:bool)
    n1209 = Greater?(x=w99, y=w98) -> (0:w100:bool)
    n1210 = local read "Induce check"() -> (w89:bool)
    n1211 = Or(x=w106, y=w100) -> (x .or. y?=w91:bool)
    n1212 = Or(x=w91, y=w89) -> (x .or. y?=w90:bool)
    n1213 = case shown="True" w90 {
      frame False {
      }
      frame True {
        n1214 = stacked-sequence {
          frame #0 {
            # "A small 100 ms delay is given to provide enough time for the data to be processed properly."
            n1215 = local read "Null array"() -> (w486:dbl[])
            n1216 = local write "What to Check"(w486) -> ()
            n1217 = local write "ID"(w486) -> ()
            n1218 = local read "Current Spot #"() -> (w488:dbl)
            n1219 = local write "Potential Collisions"(0) -> ()
            n1220 = local read "Spot Checker"() -> (w487:T2[])
            n1221 = Index Array(array=w487, index=w488) -> (element=w489:T2)
            n1222 = Wait (ms)(milliseconds to wait=10) -> ()  [unwired: 1 out]
            n1223 = Unbundle By Name(w489) -> ("Position.x"=w483:dbl, "Position.y"=w484:dbl)
            n1224 = local write "Orig Y SC"(w484) -> ()
            n1225 = local write "Orig X SC"(w483) -> ()
            n1226 = local write "Induce check"(FALSE) -> ()
          }
          frame #1 {
            n1227 = local read "# of Spots"() -> (w490:dbl)
            n1228 = for {
              N: w490 -> [_]
              tunnel: w490 -> [w495]
              i -> [w491]
              n1229 = local read "Selection/Group"() -> (w494:T8[])
              n1230 = Index Array(array=w494, index=w491) -> (element=w493:T8)
              n1231 = Unbundle By Name(w493) -> ("Selected"=w492:bool)
              n1232 = case shown="True" w492 {
                tunnel: w495 -> [_ w497]
                tunnel: w491 -> [_ w496]
                frame False {
                }
                frame True {
                  n1233 = for {
                    N: w497 -> [_]
                    tunnel: w496 -> [w498]
                    i -> [w499]
                    # "If the bubble is not selected, find difference of bubble to bubble\nbeing checked"
                    n1234 = local read "Selection/Group"() -> (w503:T8[])
                    n1235 = Index Array(array=w503, index=w499) -> (element=w502:T8)
                    n1236 = Unbundle By Name(w502) -> ("Selected"=w500:bool)
                    n1237 = Not(x=w500) -> (.not. x?=w501:bool)
                    n1238 = case shown="True" w501 {
                      tunnel: w499 -> [_ w507]
                      tunnel: w498 -> [_ w506]
                      tunnel: w498 -> [_ w505]
                      frame False {
                      }
                      frame True {
                        n1239 = local read "Spot Checker"() -> (w524:T2[])
                        n1240 = Index Array(array=w524, index=w507) -> (element=w525:T2)
                        n1241 = Index Array(array=w524, index=w506) -> (element=w523:T2)
                        n1242 = Unbundle By Name(w523) -> ("Position.x"=w520:dbl, "Position.y"=w516:dbl)
                        n1243 = Unbundle By Name(w525) -> ("Position.x"=w517:dbl, "Position.y"=w513:dbl)
                        n1244 = local read "Area+ Buffer"() -> (w504:dbl)
                        n1245 = Subtract(x=w520, y=w504) -> (x-y=w521:dbl)
                        n1246 = Greater Or Equal?(x=w517, y=w521) -> (x >= y?=w522:bool)
                        n1247 = Add(x=w516, y=w504) -> (x+y=w515:dbl)
                        n1248 = Subtract(x=w516, y=w504) -> (x-y=w514:dbl)
                        n1249 = Add(x=w520, y=w504) -> (x+y=w518:dbl)
                        n1250 = Less Or Equal?(x=w513, y=w515) -> (x <= y?=w512:bool)
                        n1251 = Greater Or Equal?(x=w513, y=w514) -> (x >= y?=w511:bool)
                        n1252 = Less Or Equal?(x=w517, y=w518) -> (x <= y?=w519:bool)
                        n1253 = And(x=w522, y=w519) -> (x .and. y?=w509:bool)
                        n1254 = And(x=w512, y=w511) -> (x .and. y?=w510:bool)
                        n1255 = And(x=w509, y=w510) -> (x .and. y?=w508:bool)
                        n1256 = case shown="True" w508 {
                          tunnel: w507 -> [_ _]
                          tunnel: w507 -> [_ w527]
                          tunnel: w505 -> [_ w526]
                          frame False {
                          }
                          frame True {
                            n1257 = stacked-sequence {
                              tunnel: w527 -> [w528 _]
                              tunnel: w526 -> [w529 _]
                              frame #0 {
                                n1258 = local read "Potential Collisions"() -> (w532:dbl)
                                n1259 = local read "What to Check"() -> (w533:dbl[])
                                n1260 = Insert Into Array(array=w533, index=w532, new element=w528) -> (w534:dbl[])
                                n1261 = local read "ID"() -> (w531:dbl[])
                                n1262 = local write "What to Check"(w534) -> ()
                                n1263 = Insert Into Array(array=w531, index=w532, new element=w529) -> (w530:dbl[])
                                n1264 = local write "ID"(w530) -> ()
                              }
                              frame #1 {
                                n1265 = local read "Potential Collisions"() -> (w537:dbl)
                                n1266 = Add(x=w537, y=1) -> (x+y=w535:dbl)
                                n1267 = local write "Potential Collisions"(w535) -> ()
                              }
                            }
                          }
                        }
                      }
                    }
                  }
                }
              }
            }
          }
          frame #2 {
            n1268 = local read "Current Spot #"() -> (w538:dbl)
            n1269 = local write "Prev Current Spot"(w538) -> ()
          }
        }
      }
    }
    n1270 = local read "Buffer Zone"() -> (w104:dbl)
    n1271 = Multiply(x=w104, y=2) -> (x*y=w105:dbl)
    n1272 = Add(x="Area to check", y=w105) -> (x+y=→"Area+ Buffer":dbl)
    n1273 = feedback #11() -> (w77:dbl)  [unwired: 1 in]
    n1274 = Equal?(x=w77, y=10000) -> (x = y?=w78:bool)
    n1275 = call "Elapsed Time"("Reset"=w78) -> ("Elapsed Time (s)"=w76:dbl, "Time has Elapsed"=w81:bool)  [unwired: 11 in, 6 out]
    "Elapsed Time" <- w76
    n1276 = feedback-in #11(w76) -> ()
    n1277 = And(x="On", y=w81) -> (x .and. y?=w82:bool)
    n1278 = case shown="True" w82 {
      frame False {
      }
      frame True {
        n1279 = local read "Position"() -> (w473:cluster{"x":dbl, "y":dbl, "z":dbl})
        n1280 = Unbundle By Name(w473) -> ("x"=→"X Pos every 10 sec":dbl)
      }
    }
    n1281 = case shown="True" "OK Button" {
      frame False {
      }
      frame True {
        n1282 = script code="clear all;\nclc;\n\ng = gigecam('169.254.154.83');\n\ng.PixelFormat= 'BayerGR8'\n\nimg = snapshot(g);\n\nimshow(img);"() -> ()  [unwired: 1 in, 1 out]
      }
    }
    n1283 = case shown="True" "O Button" {
      frame False {
      }
      frame True {
        n1284 = script code="%\n    rslt = Hough1_data(img);\n\n    % Frame translation\n    %- omit this as of now \n    \n    % Control method\n    increment = 10; %assuming the diamiter of the agent around 20 pic \n    \n    %- NewLoc = [x,y] whose unit is px\n    %- update new location based on current location obtained by the camera\n    NewLoc(1)= rslt(1);\n    NewLoc(2)= rslt(2);\n    \n    \n    % Update microrobot location with NewLoc\n    % the single robot would move to oblique downword\n    \n    % wait seconds"() -> ("NewLoc"=w469:dbl[])  [unwired: 1 in, 1 out]
        n1285 = Index Array(array=w469, index=1) -> (element=→"Y":dbl)
        n1286 = Index Array(array=w469, index=0) -> (element=→"X":dbl)
      }
    }
  }
  n1287 = flat-sequence {
    tunnel: w6 -> [w2004]
    tunnel: w5 -> [w2003]
    tunnel: [w2002] -> w3
    frame #0 {
      n1288 = disable-structure shown="\"White Image (stub)\"" {
        disable-tunnel: w2004 -> [_ _ _ _ _ _]
        disable-tunnel: w2003 -> [_ _ w2062 _ _ _]
        disable-tunnel: [_ _ w2061 _ _ _] -> w2002
        frame condition #0 {
          w2006 = u32 10 ("Number of buffers")
          (unwired) FALSE ("background subtraction")
          # "This subdiagram uses the IMAQ drivers, with a pre-allocated ringbuffer for images.  This is the code I use with my Mikrotron MC1362-CL"
          n1289 = call <vilib>:"IMAQ Init.vi"("Interface Name"="img0") -> ("IMAQ Session Out"=w2013:refnum<k11>)  [unwired: 9 in, 1 out]
          n1290 = call <vilib>:"IMAQ Configure List.vi"("Region of interest"="Global ROI (requires restart)", "Number of buffers"=w2006, "Continuous?"=enum16{"One-Shot", "Continuous"}."Continuous", "IMAQ Session In"=w2013) -> ("error out"=w2007:errorcluster, "IMAQ Session Out"=w2009:refnum<k11>)  [unwired: 6 in]
          n1291 = for {
            N: w2006 -> [_]
            tunnel: 0 ("Channel") -> [w2026]
            shift-right: [w2029] -> w2011
            shift-left: w2007 -> [w2025]
            shift-right: [w2028] -> w2010
            shift-left: w2009 -> [w2027]
            i -> [w2024]
            n1292 = Format Into String(format string="mikrotronbuffer%04d", w2024) -> (resulting string=w2022:string)  [unwired: 2 in, 1 out]
            n1293 = call "IMAQ Create"("Image Name"=w2022) -> ("New Image"=w2021:T9)  [unwired: 4 in, 1 out]
            n1294 = call <vilib>:"IMAQ Configure Buffer.vi"("Channel"=w2026, "error in (no error)"=w2025, "Buffer Number"=w2024, "Image In"=w2021, "IMAQ Session In"=w2027) -> ("error out"=w2029:errorcluster, "IMAQ Session Out"=w2028:refnum<k11>)  [unwired: 5 in]
          }
          n1295 = call <vilib>:"IMAQ Start.vi"("error in (no error)"=w2011, "IMAQ Session In"=w2010) -> ("error out"=w2017:errorcluster, "IMAQ Session Out"=w2018:refnum<k11>)  [unwired: 8 in]
          n1296 = call "IMAQ Create"("Image Name"="Red Tweezers live image") -> ("New Image"=w2019:T9)  [unwired: 3 in, 2 out]
          n1297 = while {
            tunnel: w2018 -> [w2037]
            tunnel: w2017 -> [w2036]
            tunnel: w2019 -> [_]
            tunnel: [w2038] -> w2015
            tunnel: [w2031] -> w2016
            i -> [w2033]
            stop <- w2039 stop-if-true
            n1298 = local read "stop"() -> (w2039:bool)
            n1299 = call <vilib>:"IMAQ Extract Buffer.vi"("error in (no error)"=w2036, "Buffer to extract"=w2033, "IMAQ Session In"=w2037) -> ("error out"=w2031:errorcluster, "Image Out"=w2030:T9, "IMAQ Session Out"=w2038:refnum<k11>)  [unwired: 3 in, 3 out]
            n1300 = call "imageQ_camera_hook.vi"("Image"=w2030) -> ()  [unwired: 11 in]
            n1301 = feedback #12() -> (w2034:T31)  [unwired: 1 in]
            n1302 = call "Smoothed Frame Rate.vi"("Feedback In"=w2034) -> ("Feedback Out"=w2035:T31, "Frame Rate"=w2032:dbl)  [unwired: 1 in, 4 out]
            n1303 = feedback-in #12(w2035) -> ()
            n1304 = global write "red_tweezers_globals_INTERNAL_VOLATILE.vi" "Video Frame Rate"(w2032) -> ()
          }
          n1305 = call <vilib>:"IMAQ Close.vi"("error in (no error)"=w2016, "IMAQ Session In"=w2015) -> ()  [unwired: 9 in, 1 out]
        }
        frame condition #1 {
          (unwired) FALSE ("background subtraction")
          # "This subdiagram acquires using the IMAQdx drivers.  This covers most FireWire and GigE cameras (at least the ones supporting the IIDC or GenICam standards)."
          n1306 = call <vilib>:"IMAQdx Open Camera.vi"("Session In"=T7 "dalsaGenie") -> ("error out"=w2042:errorcluster, "Session Out"=w2041:T7)  [unwired: 9 in]
          n1307 = call <vilib>:"IMAQdx Configure Grab.vi"("error in"=w2042, "Session In"=w2041) -> ("error out"=w2043:errorcluster, "Session Out"=w2044:T7)  [unwired: 8 in]
          n1308 = call "IMAQ Create"("Image Name"="Red Tweezers live image") -> ("New Image"=w2047:T9)  [unwired: 3 in, 2 out]
          n1309 = while {
            tunnel: w2044 -> [w2056]
            tunnel: w2043 -> [w2055]
            tunnel: w2047 -> [w2049]
            tunnel: [w2057] -> w2045
            tunnel: [w2051] -> w2046
            stop <- w2058 stop-if-true
            n1310 = local read "stop"() -> (w2058:bool)
            n1311 = call <vilib>:"IMAQdx Grab.vi"("error in"=w2055, "Image In"=w2049, "Session In"=w2056) -> ("error out"=w2051:errorcluster, "Image Out"=w2050:T9, "Session Out"=w2057:T7)  [unwired: 5 in, 1 out]
            n1312 = call "imageQ_camera_hook.vi"("Image"=w2050) -> ()  [unwired: 11 in]
            n1313 = feedback #13() -> (w2053:T31)  [unwired: 1 in]
            n1314 = call "Smoothed Frame Rate.vi"("Feedback In"=w2053) -> ("Feedback Out"=w2054:T31, "Frame Rate"=w2052:dbl)  [unwired: 1 in, 4 out]
            n1315 = feedback-in #13(w2054) -> ()
            n1316 = global write "red_tweezers_globals_INTERNAL_VOLATILE.vi" "Video Frame Rate"(w2052) -> ()
          }
          n1317 = call <vilib>:"IMAQdx Close Camera.vi"("error in"=w2046, "Session In"=w2045) -> ()  [unwired: 9 in, 1 out]
        }
        frame condition #2 {
          # "This subdiagram acquires using the IMAQdx drivers.  This covers most FireWire and GigE cameras (at least the ones supporting the IIDC or GenICam standards)."
          n1318 = call <vilib>:"IMAQdx Open Camera.vi"("Session In"="Camera") -> ("error out"=w2070:errorcluster, "Session Out"=w2069:T7)  [unwired: 9 in]
          n1319 = call <vilib>:"IMAQdx Configure Grab.vi"("error in"=w2070, "Session In"=w2069) -> ("error out"=w2066:errorcluster, "Session Out"=w2067:T7)  [unwired: 8 in]
          n1320 = call "IMAQ Create"("Image Name"="Red Tweezers live image") -> ("New Image"=w2064:T9)  [unwired: 3 in, 2 out]
          n1321 = call "IMAQdx_get_ROI.vi"("Session In"=w2067) -> ("ROI"=w2063:u32[], "Session Out"=w2065:T7)  [unwired: 8 in]
          n1322 = while {
            shift-right: [w2079] -> w2059
            shift-left: w2066 -> [w2080]
            shift-right: [w2076] -> w2060
            shift-left: w2065 -> [w2077]
            tunnel: w2064 -> [w2075]
            tunnel: w2063 -> [w2074]
            tunnel: w2062 -> [w2073]
            tunnel: [w2072] -> w2061
            stop <- w2086 stop-if-true
            n1323 = event shown="[0] Timeout" {
              selector: _ -> [_ _ _]
              dyn-events: _ -> [_ _ _]
              timeout: 0 -> [_ _ _]
              tunnel: w2080 -> [w2093 w2100 w2115]
              tunnel: [w2092 w2100 w2115] -> w2079
              tunnel: w2077 -> [w2091 w2101 w2116]
              tunnel: [w2090 w2101 w2116] -> w2076
              tunnel: w2075 -> [w2089 _ _]
              tunnel: w2074 -> [w2088 _ _]
              tunnel: w2073 -> [_ w2099 w2114]
              event Timeout {
                w2087 = 0  # timeout in ms
                # "Use a timeout of a few hundred ms if you want to acquire just fast enough to update the image- or a timeout of zero to run the camera at full speed."
                # "This VI sends the image to the loop above for display.\nIt's better to do this than to display here, because it separates the camera loop from the front panel a bit, and increases speed without sacrificing responsiveness of the UI.  Of course, using the event structure removes some of those benefits- but it is possible to write a high-performance camera loop with fast particle tracking, and still use this mechanism to display images without slowing down acquisition."
                # "If we're not dealing with other events, acquire from the camera."
                n1324 = event-data() -> ("Time"=w2098:u32)  [unwired: 1 in]
                n1325 = call <vilib>:"IMAQdx Grab.vi"("error in"=w2093, "Image In"=w2089, "Session In"=w2091) -> ("error out"=w2092:errorcluster, "Image Out"=w2095:T9, "Session Out"=w2090:T7)  [unwired: 5 in, 1 out]
                n1326 = call "IMAQ Clear Overlay"("Image"=w2095) -> ("Image Out"=w2094:T9)  [unwired: 9 in, 1 out]
                n1327 = Multiply(x=w2098, y=u32 1000) -> (x*y=w2096:u32)
                n1328 = call "imageQ_camera_hook.vi"("timeout in ms (0=don't wait if there are no requests)"=w2087, "Timestamp/us"=w2096, "ROI"=w2088, "Image"=w2094) -> ()  [unwired: 8 in]
              }
              event "Draw ROI", "Zoom": Value Change {
                # "This changes the current mouse mode on the image, allowing zooming/drawing of ROI (which can be useful if you want to window down a camera for particle tracking)."
                n1329 = event-data() -> ("CtlRef"=w2106:refnum<vi>)  [unwired: 1 in]
                n1330 = control-ref of="Draw ROI"() -> (w2107:refnum<vi>)
                n1331 = Equal?(x=w2107, y=w2106) -> (x = y?=w2105:bool)
                n1332 = case shown="True" w2105 {
                  tunnel: [w2110 w2113] -> w2104
                  tunnel: [TRUE ("stop") FALSE ("stop")] -> w2102
                  tunnel: [FALSE ("Update Indicators?") TRUE ("Update Indicators?")] -> w2103
                  frame False {
                    w2110 = u32 8 items=["Zoom Tool"=8, "Selection Tool"=0, "Pan Tool"=9, "Point Tool"=1, "Line Tool"=2, "Rectangle Tool"=3, "Rotated Rectangle Tool"=12, "Polyline Tool"=10, "Polygon Tool"=5, "Freehand Tool"=11, "Closed Freehand Tool"=6, "Ellipse Tool"=4, "Annulus Tool"=7] ("Current ROI Tool")
                  }
                  frame True {
                    w2113 = u32 3 items=["Zoom Tool"=8, "Selection Tool"=0, "Pan Tool"=9, "Point Tool"=1, "Line Tool"=2, "Rectangle Tool"=3, "Rotated Rectangle Tool"=12, "Polyline Tool"=10, "Polygon Tool"=5, "Freehand Tool"=11, "Closed Freehand Tool"=6, "Ellipse Tool"=4, "Annulus Tool"=7] ("Current ROI Tool")
                  }
                }
                n1333 = local write "Draw ROI"(w2103) -> ()
                n1334 = local write "Zoom"(w2102) -> ()
                n1335 = property on="Property Node" class="ImageControl"(reference=w2099, "Current ROI Tool"=w2104) -> ()  [unwired: 1 in, 2 out]
              }
              event "Zoom to Fit": Value Change {
                # "The various ROI tools are hidden, so the image control resizes nicely as the Red Tweezers window is resized.  The zoom to fit button/mouse mode buttons return some of this functionality."
                n1336 = event-data() -> ("NewVal"=w2117:bool)  [unwired: 1 in]
                n1337 = property on="Property Node" class="ImageControl"(reference=w2114, "Zoom to Fit Mode"=w2117) -> ()  [unwired: 1 in, 2 out]
              }
            }
            n1338 = feedback #14() -> (w2085:T31)  [unwired: 1 in]
            n1339 = call "Smoothed Frame Rate.vi"("Feedback In"=w2085, "Alpha"=0.05) -> ("Feedback Out"=w2084:T31, "Frame Rate"=w2081:dbl)  [unwired: 4 out]
            n1340 = feedback-in #14(w2084) -> ()
            n1341 = global write "red_tweezers_globals_INTERNAL_VOLATILE.vi" "Video Frame Rate"(w2081) -> ()
            n1342 = local read "stop"() -> (w2082:bool)
            n1343 = Unbundle By Name(w2079) -> ("status"=w2072:bool)
            n1344 = Or(x=w2072, y=w2082) -> (x .or. y?=w2086:bool)
          }
          n1345 = call <vilib>:"IMAQdx Close Camera.vi"("error in"=w2059, "Session In"=w2060) -> ()  [unwired: 9 in, 1 out]
        }
        frame condition #3 (active) {
          w2119 = 0 ("element")
          w2121 = 1920 ("dimension size")
          w2120 = 1080 ("dimension size")
          w2122 = T17 0 items=["Grayscale (U8)", "Grayscale (I16)", "Grayscale (SGL)", "Complex (CSG)", "RGB (U32)", "HSL (U32)", "RGB (U64)", "Grayscale (U16)"] ("Image Type")
          (unwired) FALSE ("background subtraction")
          # "This subdiagram generates a blank white image- useful if you don't have a camera"
          n1346 = Build Array(w2119, w2119, w2121, w2120) -> (w2118:i32[])
          n1347 = Initialize Array(u8 255 ("element"), w2120, w2121) -> (w2123:u8[][])
          n1348 = global write "red_tweezers_globals_INTERNAL.vi" "Global ROI"(w2118) -> ()
          n1349 = call "IMAQ Create"("Image Name"="red tweezers camera stub", "Image Type"=w2122) -> ("New Image"=w2124:T9)  [unwired: 2 in, 2 out]
          n1350 = call "IMAQ ArrayToImage"("Image Pixels (U8)"=w2123, "Image"=w2124) -> ("Image Out"=w2127:T9)  [unwired: 8 in, 1 out]
          n1351 = call "IMAQ Create"("Image Name"="Red Tweezers live image") -> ("New Image"=w2128:T9)  [unwired: 3 in, 2 out]
          n1352 = while {
            tunnel: w2127 -> [w2131]
            tunnel: w2128 -> [_]
            stop <- w2135 stop-if-true
            n1353 = local read "stop"() -> (w2135:bool)
            n1354 = Wait Until Next ms Multiple(millisecond multiple=u32 20) -> ()  [unwired: 1 out]
            n1355 = call "imageQ_camera_hook.vi"("Image"=w2131) -> ()  [unwired: 11 in]
            n1356 = feedback #15() -> (w2133:T31)  [unwired: 1 in]
            n1357 = call "Smoothed Frame Rate.vi"("Feedback In"=w2133) -> ("Feedback Out"=w2134:T31, "Frame Rate"=w2132:dbl)  [unwired: 1 in, 4 out]
            n1358 = feedback-in #15(w2134) -> ()
            n1359 = global write "red_tweezers_globals_INTERNAL_VOLATILE.vi" "Video Frame Rate"(w2132) -> ()
          }
        }
        frame condition #4 {
          # "Use this subdiagram if you have an external camera VI which writes to the image queue (using imageQ_camera_hook.vi)"
        }
        frame condition #5 {
          w2136 = path "C:/Users/Tweezer Cube/Desktop/red_tweezers_1_4_rc0/camera_for_rt136.llb/Particle Tracking.vi"  # Path to camera VI
          # "Use this subdiagram if you have an external camera VI which writes to the image queue (using imageQ_camera_hook.vi).  This is the slightly more sophisticated version, which checks that said external VI is running, and runs it if not."
          n1360 = Open VI Reference(vi path=w2136) -> (vi reference=w2137:refnum<vi>, error out=w2139:errorcluster)  [unwired: 5 in]
          n1361 = property class="VI"(reference=w2137) -> ("Path"=w2138:path)  [unwired: 1 in, 2 out]
          n1362 = global write "red_tweezers_globals_INTERNAL_VOLATILE.vi" "Current Camera VI"(w2138) -> ()
          n1363 = property class="VI"(reference=w2137, error in=w2139) -> (reference out=w2144:refnum<vi>, error out=w2143:errorcluster, "Exec.State"=w2141:T33)
          n1364 = Equal?(x=w2141, y=T33."Idle") -> (x = y?=w2145:bool)
          n1365 = case shown="True" w2145 {
            tunnel: w2144 -> [w2149 w2158]
            tunnel: w2143 -> [w2148 w2155]
            tunnel: [w2147 w2154] -> w2140
            tunnel: w2141 -> [w2151 _]
            frame False {
              n1366 = Close Reference(reference=w2149, error in (no error)=w2148) -> (error out=w2147:errorcluster)
              n1367 = Equal?(x=w2151, y=T33."Bad") -> (x = y?=w2150:bool)
              n1368 = case shown="False" w2150 {
                frame False {
                }
                frame True {
                  n1369 = One Button Dialog(message="The external camera VI is not running and cannot be started- it's probably broken or missing.  Check the static/dynamically loaded VI reference in the bottom loop on the block diagram.") -> ()  [unwired: 1 in, 1 out]
                }
              }
            }
            frame True {
              n1370 = invoke class="VI" method="Run VI"(reference=w2158, error in=w2155, "Wait until done"=FALSE ("Wait Until Done"), "Auto Dispose Ref"=TRUE ("Auto Dispose Reference")) -> (error out=w2154:errorcluster)  [unwired: 1 in, 4 out]
            }
          }
          n1371 = call <vilib>:"Simple Error Handler.vi"("error source (\" \")"="External camera VI (see the bottom loop in the block diagram)" ("error source (\" \")"), "error in (no error)"=w2140) -> ()  [unwired: 3 in, 5 out]
        }
      }
    }
  }
  n1372 = while {
    tunnel: w9 -> [w2176]
    shift-right: [w2175] -> w8
    shift-left: w10 -> [w2177]
    shift-right: [w2172] -> _
    shift-left: _ -> [w2165]
    shift-right: [w2171] -> _
    shift-left: _ -> [w2169]
    shift-right: [w2170] -> _
    shift-left: FALSE ("Saving") -> [w2166]
    stop <- w2174 stop-if-true
    w2163 = u32 50 ("millisecond multiple")
    # "Start/stop saving data, if necessary"
    n1373 = Divide(x=u32 1000, y=w2163) -> (x/y=w2161:dbl)
    n1374 = Wait Until Next ms Multiple(millisecond multiple=w2163) -> ()  [unwired: 1 out]
    n1375 = call "imageQ_dequeue.vi"("timeout in ms (-1)"=2000, "Return queue"=w2177, "Image Dst"=w2176) -> ("Timestamp/us"=w2167:u64, "Return queue out"=w2175:refnum<queue>, "Image Dst Out"=w2178:T9, "timed out?"=w2181:bool, "ROI"=w2160:u64[])  [unwired: 4 in]
    n1376 = Not(x=w2181) -> (.not. x?=w2179:bool)
    n1377 = case shown="True" w2179 {
      tunnel: w2178 -> [_ w2215]
      tunnel: w2169 -> [w2208 w2218]
      tunnel: w2166 -> [_ w2212]
      tunnel: [w2208 w2213] -> w2168
      tunnel: w2167 -> [_ w2216]
      tunnel: w2165 -> [w2209 w2217]
      tunnel: [w2209 w2214] -> w2164
      tunnel: w2160 -> [_ w2211]
      frame False {
      }
      frame True {
        n1378 = global read "red_tweezers_globals_INTERNAL.vi" "Image Overlay (extras from control loop)"() -> (w2226:T19[])
        n1379 = case shown="True" w2212 {
          tunnel: w2218 -> [w2227 w2229]
          tunnel: w2217 -> [w2228 w2235]
          tunnel: w2216 -> [_ w2234]
          tunnel: w2215 -> [_ w2233]
          tunnel: [w2228 w2232] -> w2214
          tunnel: [w2227 w2231] -> w2213
          frame False {
          }
          frame True {
            n1380 = call "save_data_save.vi"("Image"=w2233, "Timestamp"=w2234, "Avi Refnum"=w2229, "Data refnum"=w2235) -> ("error out"=w2230:errorcluster, "Avi Refnum (duplicate)"=w2231:T34, "Data refnum (duplicate)"=w2232:refnum<file>)  [unwired: 5 in]
            n1381 = case shown="Error" w2230 {
              selector: w2230 -> [_ w2237]
              frame No Error {
              }
              frame Error {
                n1382 = call <vilib>:"Clear Errors.vi"("error in (no error)"=w2237) -> ()  [unwired: 5 in, 2 out]
                n1383 = local write "Save Video"(FALSE ("Save")) -> ()
              }
            }
          }
        }
        n1384 = global write "red_tweezers_globals_INTERNAL.vi" "Global ROI"(w2211) -> ()
        n1385 = global read "red_tweezers_globals_INTERNAL_VOLATILE.vi" "Tracked Spot Positions (3D)"() -> (w2219:cluster{"x":dbl, "y":dbl, "Z":dbl}[])
        n1386 = global read "red_tweezers_globals.vi" "Selection/Group"() -> (w2225:T8[])
        n1387 = global read "red_tweezers_globals.vi" "Spots"() -> (w2224:T2[])
        n1388 = call "overlay_positions.vi"("Positions"=w2219, "Image"=w2215) -> ("Image 2"=w2221:T9)  [unwired: 9 in]
        n1389 = call "render_overlay_elements.vi"("Image Overlay (extras from control loop)"=w2226, "Image"=w2221) -> ("Image Out"=w2223:T9)  [unwired: 5 in]
        n1390 = call "grid_and_guides.vi"("Operation"=T14."Render on image", "Image"=w2223) -> ("Image Out"=w2210:T9)  [unwired: 9 in]
        n1391 = call "overlay_spots_on_image.vi"("Selection and Groups"=w2225, "Spots"=w2224, "image"=w2210) -> ("Image"=→"Image":T9)  [unwired: 3 in, 1 out]
      }
    }
    n1392 = global read "red_tweezers_globals_INTERNAL_VOLATILE.vi" "Video Frame Rate"() -> (→"Video Frame Rate":dbl)
    n1393 = case shown="True" "Save Video" {
      tunnel: [w2184 w2199] -> w2172
      tunnel: [w2183 w2193] -> w2171
      tunnel: [FALSE ("Saving") w2198] -> w2170
      tunnel: w2166 -> [w2187 w2197]
      tunnel: w2168 -> [w2185 w2196]
      tunnel: w2164 -> [w2186 w2195]
      tunnel: w2161 -> [_ w2194]
      frame False {
        n1394 = case shown="True" w2187 {
          tunnel: w2186 -> [w2189 w2192]
          tunnel: w2185 -> [w2188 w2191]
          tunnel: [w2189 _] -> w2184
          tunnel: [w2188 _] -> w2183
          frame False {
          }
          frame True {
            n1395 = local write "Save Video"(FALSE ("Save")) -> ()
            n1396 = call "save_data_stop.vi"("Avi Refnum"=w2191, "Data refnum"=w2192) -> ()  [unwired: 10 in]
          }
        }
      }
      frame True {
        n1397 = case shown="False" w2197 {
          selector: w2197 -> [_ w2207]
          tunnel: [w2204 w2205] -> w2199
          tunnel: [w2203 w2206] -> w2193
          tunnel: [w2200 w2207] -> w2198
          tunnel: w2196 -> [_ w2206]
          tunnel: w2195 -> [_ w2205]
          tunnel: w2194 -> [w2202 _]
          frame False {
            n1398 = call "save_data_start.vi"("Save Video"=TRUE, "Frames Per Second"=w2202) -> ("Saving"=w2200:bool, "Avi Refnum"=w2203:T34, "Data Refnum"=w2204:refnum<file>)  [unwired: 3 in]
            n1399 = local write "Save Video"(w2200) -> ()
          }
          frame True {
          }
        }
      }
    }
    n1400 = local read "stop"() -> (w2174:bool)
  }
  n1401 = Release Queue(queue=w8) -> ()  [unwired: 2 in, 3 out]
  n1402 = case shown="True" w3 {
    frame False {
    }
    frame True {
      n1403 = One Button Dialog(message="Warning: there was a camera error.  You may need to restart Red Tweezers.") -> ()  [unwired: 1 in, 1 out]
    }
  }
  n1404 = flat-sequence {
    tunnel: w18 -> [w2243]
    tunnel: w17 -> [_]
    frame #0 {
      # "This autosaves when we stop.  The sequence structures are necessary so that:\n1. loading settings doesn't stop the VI\n2. plugins are still open (and hence saved) when we save settings"
      n1405 = local read "Plugins"() -> (w2246:T4)
      n1406 = global read "red_tweezers_globals_INTERNAL_VOLATILE.vi" "Current Settings File"() -> (w2240:path)
      n1407 = global read "red_tweezers_globals_INTERNAL_VOLATILE.vi" "Save Settings On Exit"() -> (w2239:bool)
      n1408 = flat-sequence {
        tunnel: w2243 -> [w2249]
        tunnel: [w2249] -> w2242
        frame #0 {
          n1409 = local write "stop"(FALSE ("STOP")) -> ()
        }
      }
      n1410 = case shown="True" w2239 {
        tunnel: w2240 -> [_ w2254]
        tunnel: w2242 -> [w2251 w2252]
        tunnel: [w2251 w2252] -> w2241
        frame False {
        }
        frame True {
          n1411 = Path To String(path=w2254) -> (string=w2253:string)
          n1412 = call "settings_save_to_file.vi"("XML File Path"=w2254) -> ()  [unwired: 11 in]
          n1413 = call "settings_filename_to_registry.vi"("Last Used Settings File"=w2253) -> ()  [unwired: 11 in]
        }
      }
      n1414 = flat-sequence {
        tunnel: w2241 -> [w2247]
        tunnel: [w2247] -> _
        frame #0 {
          n1415 = local write "stop"(TRUE ("STOP")) -> ()
        }
      }
      n1416 = control-ref of="Plugin Pnl"() -> (w2244:refnum<vi>)
      n1417 = control-ref of="Plugin:"() -> (w2245:refnum<vi>)
      n1418 = call "plugins_unload.vi"("error in (no error)"=w2241, "Plugins"=w2246, "Sub Panel"=w2244, "Plugin Chooser"=w2245) -> ()  [unwired: 2 in, 2 out]
    }
  }
